vi "myRIO_BRig_RT_v0,73__PortC.vi"() -> ()   [LabVIEW 2014]
uses:
  myRIO_BRig_RT__Case_Exp_stateList.ctl
  myRIO_BRig_RT__Case_NonExp_stateList.ctl
  <vilib>/Platform/TimedLoop/XDataNode/timing_clust.ctl
  <vilib>/Platform/TimedLoop/XDataNode/nitl_modes.ctl
  <vilib>/Platform/TimedLoop/XDataNode/wakeup.ctl
  <vilib>/WebDAVClient/Advanced/SessionHandle.ctl
  <vilib>/myRIO/Common/Instrument Driver Framework/myRIO v1.0/UART/vis/myRIO v1.0 Close UART.vi
  <vilib>/FPGAPlugInAG/myRIO-1900/niLvFpga_Open_myRIO-1900.vi
  <vilib>/rvi/interface/common/dynamic/niFpgaDynamicAddResources.vi
  <vilib>/Utility/error.llb/Error Cluster From Error Code.vi
  <vilib>/rvi/errors/niLvFpgaAdjustHostInterfaceError.vi
  <vilib>/FPGAPlugInAG/Dynamic/niLvFpga_Close_Dynamic.vi
  <vilib>/myRIO/Common/Instrument Driver Framework/Utilities/vis/FPGA Ref Manager.vi
  <vilib>/myRIO/Common/Instrument Driver Framework/myRIO v1.0/myRIO v1.0 Reset FPGA.vi
  <vilib>/myRIO/Common/Instrument Driver Framework/myRIO v1.0/IRQ/vis/myRIO v1.0 IRQ Info FGV.vi
  <vilib>/myRIO/Common/Instrument Driver Framework/myRIO v1.0/IRQ/vis/myRIO v1.0 Timer IRQ Info FGV.vi
  <vilib>/myRIO/Common/Instrument Driver Framework/myRIO v1.0/IRQ/vis/myRIO v1.0 ISR Agent.vi
  <vilib>/rvi/interface/nirviOpenFPGA/nirviOpenFPGA.xnode
  myRIO_BRig_FPGA_v3,60__PortC__build.lvbitx
  myRIO_BRig_FPGA_v3,60__PortC.vi
  <vilib>/rvi/interface/nirviReadWriteControl/nirviReadWriteControl.xnode
  <vilib>/Platform/TimedLoop/XDataNode/XDataNode.xnode
  <vilib>/rvi/interface/nirviCloseFPGA/nirviCloseFPGA.xnode
  <vilib>/Platform/TimedLoop/XDataNode/XDNodeRunTimeDep.lvlib
  <vilib>/rvi/interface/Simulation/niFpgaSimulationCallBeginRW.vi
  <vilib>/myRIO/Instrument Drivers/Utilities/Utilities.lvlib
  <vilib>/WebDAVClient/NI_WebDAV.lvlib
  NiFpgaLv.dll
panel:
  in  "LC_Sel_All_Count":u16
  in  "LC_Sel_First_Count":u16
  in  "LC_Sel_All_Probability":u16
  in  "LC_Sel_All_Block":u16(slide) max=2 step=1 scale=0.0..2.0
  in  "LC_Sel_All_OnOff":bool
  in  "LC_Sel_First_Probability":u16
  in  "LC_Sel_First_Block":u16(slide) max=2 step=1 scale=0.0..2.0
  in  "LC_Sel_First_OnOff":bool
  in  "LC_Sel_All_Tdelay":u16
  in  "LC_Sel_First_Tdelay":u16
  out "I_connect_TCP":bool
  out "tempAI0":i16
  out "error out 5":errorcluster
  in  "get_countPerMS":bool
  in  "count_warmup_R_reset":bool
  in  "count_warmup_L_reset":bool
  out "count_warmup_R":u16
  out "count_warmup_L":u16
  out "SolenoidReward":bool
  in  "SolenoidProbability_L":u16=50 caption="Reward Time [ms]" min=1 max=1000 step=1
  in  "SolenoidProbability_R":u16=50 caption="Reward Time [ms]" min=1 max=1000 step=1
  out "output_PortA":dbl caption="LaserPower"
  out "error out 4":errorcluster
  in  "laser_power_step":dbl
  in  "laser_power_max":dbl
  in  "Recording":bool
  out "error out 3":errorcluster
  out "error out 2":errorcluster
  in  "laser_power_min":dbl
  in  "f_millisec2count":dbl=159.0
  in  "laser_Tshutter":dbl=2.0
  in  "laser_Freq":dbl=10.0
  in  "laser_Tpeak":dbl=2.0
  in  "laser_duration":u16
  out "error out":errorcluster
  in  "LC_Cue1_All_Count":u16
  in  "LC_Cue1_First_Count":u16
  in  "LC_Cue1_All_delayOpt":bool
  in  "LC_ENL1_All_delayOpt":bool
  in  "LC_ENL1_All_Count":u16
  in  "LC_ENL1_First_Count":u16
  in  "LC_Cue1_First_delayOpt":bool
  in  "LC_ENL1_First_delayOpt":bool
  in  "Tcycle_Cue_max":u16=1000 caption="Max" min=5 max=5000 step=5
  in  "Tcycle_Cue_min":u16=1000 caption="Min" min=5 max=5000 step=5
  in  "SendData":bool
  out "cSpout":enum16{"Left", "Right"}(ring) caption="Left or Right Spout"
  out "A4":u32 caption="LickCounter_Right"
  out "A2":u32 caption="LickCounter_Left"
  in  "laserResponse_wrong_LED":bool
  out "error_initTrial":errorcluster
  out "error_Selection_pre":errorcluster
  out "error_Selection":errorcluster
  out "SelectWrong":bool
  out "SelectReward":bool
  in  "Left(F)_or_Right(T)":bool
  in  "ignoreWrong":bool
  in  "SelectionState":bool
  in  "laserResponse_wrong":bool
  in  "laserResponse_reward":bool
  in  "laserResponse_reward_LED":bool
  out "nRewards_Right":u16 caption="# Rewards Total (Right)"
  out "nRewards_Left":u16 caption="# Rewards Total (Left)"
  out "nRewards_cur":u16 caption="# Rewards in Current Block"
  out "TpB_target":u16 caption="Target Trials Per Block"
  out "cState_NonExp":T1 caption="WarmUp State"
  out "iBlock":u16 caption="Current Block"
  out "cState":T2 caption="Experimental State"
  out "iTrial":u16 caption="Current Trial"
  in  "warmupType":u8(slide) max=2 step=1 scale=0.0..2.0
  in  "TestConnection":bool
  in  "warmup":bool caption="WarmUp"
  in  "Data Set Prefix":string="Exp1_TM2"
  out "Connected To Host?":bool
  in  "Host Password":string="sabalab"
  in  "Host UserName":string="Test2"
  in  "sp_RightSpout":u16(slide)=2 max=2 step=1 scale=0.0..2.0
  in  "sp_LeftSpout":u16(slide)=2 max=2 step=1 scale=0.0..2.0
  in  "BUR_max":u16 caption="Count Reward Structure  (0 = off)"
  in  "LC_Wrong_Probability":u16
  in  "LC_Wrong_Trial":u16(slide) max=2 step=1 scale=0.0..2.0
  in  "LC_Wrong_Block":u16(slide) max=2 step=1 scale=0.0..2.0
  in  "LC_Wrong_OnOff":bool
  in  "LC_Reward_Probability":u16
  in  "LC_Reward_Trial":u16(slide) max=2 step=1 scale=0.0..2.0
  in  "LC_Reward_Block":u16(slide) max=2 step=1 scale=0.0..2.0
  in  "LC_Reward_OnOff":bool
  in  "LC_Cue1_All_Probability":u16
  in  "LC_Cue1_All_Block":u16(slide) max=2 step=1 scale=0.0..2.0
  in  "LC_Cue1_All_OnOff":bool
  in  "LC_Cue1_First_Probability":u16
  in  "LC_Cue1_First_Block":u16(slide) max=2 step=1 scale=0.0..2.0
  in  "LC_Cue1_First_OnOff":bool
  in  "LC_ENL1_All_Probability":u16 max=100 step=1
  in  "LC_ENL1_All_Block":u16(slide) max=2 step=1 scale=0.0..2.0
  in  "LC_ENL1_All_OnOff":bool
  in  "LC_ENL1_First_Probability":u16 max=100 step=1
  in  "LC_ENL1_First_Block":u16(slide) max=2 step=1 scale=0.0..2.0
  in  "Tcycle_Timeout":u16=1000 caption="Timeout Time [ms]" min=10 max=10000 step=1
  in  "Tcycle_Wrong":u16=1000 caption="Wrong Time [ms]" min=10 max=10000 step=1
  in  "Tcycle_Selection":u16=1000 caption="Answer Time [ms]" min=1 max=10000 step=1
  in  "Tcycle_RewardPost":u16=1000 caption="Consumption Time [ms]" min=250 max=10000 step=250
  in  "Tcycle_Reward_L":u16=500 caption="Reward Time [ms]" min=1 max=1000 step=1
  in  "Tcycle_Reward_R":u16=500 caption="Reward Time [ms]" min=1 max=1000 step=1
  in  "TpB_Max_R":u16=4 caption="Max TrialsPerBlock" min=1 max=12 step=1
  in  "TpB_Min_R":u16=4 caption="Min TrialsPerBlock" min=1 max=12 step=1
  in  "TpB_Max_L":u16=4 caption="Max TrialsPerBlock" min=1 max=12 step=1
  in  "TpB_Min_L":u16=4 caption="Min TrialsPerBlock" min=1 max=12 step=1
  in  "BUR_min":u16 caption="Count Reward Structure\n(0 = off)"
  in  "TrialUntilReward":bool caption="Ignore Wrong Selection"
  in  "CueCycles":u16=1 caption="Cue Structure" min=1 max=1 step=1
  in  "MTrig_Laser_Tcycle":u16=10 caption="Time [ms]"
  in  "MTrig_Laser_trig":bool
  in  "MTrig_Audio_trig__R":bool caption="Trigger Audio"
  in  "MTrig_Audio_trig__L":bool caption="Trigger Audio"
  in  "RewCalib_Trig_R":bool caption="Calibrate_R"
  in  "RewCalib_Trig_L":bool caption="Calibrate_L"
  in  "MTrig_Solenoid_Tcycle__R":u16=300 caption="Time [ms]"
  in  "MTrig_Solenoid_Tcycle__L":u16=300 caption="Time [ms]"
  in  "MTrig_Solenoid_trig__R":bool caption="Solenoid"
  in  "MTrig_Solenoid_trig__L":bool caption="Solenoid"
  in  "STOP_abort":bool caption="Stop LabView\n(Stops myRio and FPGA)"
  in  "STOP_endBlock":bool caption="Stop Experiment\n@ End of Block"
  in  "STOP_endTrial":bool caption="Stop Experiment\n@ End of Trial"
  in  "START":bool caption="Start Experiment"
  in  "Tcycle_CuePenalty":u16=1000 caption="Penalty" min=1 max=10000 step=1
  in  "Audio_Amp__R":u16=100 caption="Amp"
  in  "Audio_Freq__R":u8=5 caption="Freq [kHz]" max=14 step=1
  in  "Audio_Amp__L":u16=100 caption="Amp"
  in  "Audio_Freq__L":u8=5 caption="Freq [kHz]" max=14 step=1
  in  "LC_Wrong_Tdelay":u16
  in  "LC_Cue1_All_Tdelay":u16
  in  "LC_ENL1_All_Tdelay":u16
  in  "LC_Reward_Tdelay":u16
  in  "LC_Cue1_First_Tdelay":u16
  in  "LC_ENL1_First_Tdelay":u16
  in  "LC_ENL1_First_OnOff":bool
  in  "Tcycle_ENLPenalty":u16=100 caption="Penalty" min=10 max=10000 step=10
  in  "Tcycle_ENL_max":u16=1000 caption="Max" min=250 max=10000 step=250
  in  "Tcycle_ENL_min":u16=1000 caption="Min" min=250 max=10000 step=250
  # "Experimental Run"
  # "Experiment Task Structure"
  # "Current State"
  # "Timing [ms]"
  # "Global Parameters\n \n   WarmUp State                                            Lick Counter"
  # "Min            Max            Penalty"
  # "(1) = Switching\n(2) = Two Choice"
  # "Enforced\nNonLick"
  # "Left                    Right"
  # "Cue"
  # "Experimental State"
  # "Communication (Host PC)"
  # "WarmUp"
  # "Selection\n \n \nReward\n    Dispense\n    Time\n \n    Dispense\n    Probability\n \n    Consumption\n    Time\n \nWrong Choice\n \n \nTimeout Penalty"
  # "Trial Parameters\n \n   Left/Right        Give Reward?        Laser Power [V]"
  # "Left                  Right"
  # "Min"
  # "Max"
  # "Block                   Trial            Target Trials       # Rewards \n                                                            Per Block             Current"
  # "Trial Per Block Structure \n               Left                        Right"
  # "Min"
  # "# Rewards Total\n                                                                  Left                    Right"
  # "Recording Rig"
  # "FPGA Conv."
  # "Cue then reward (no lick)\n \nLeft                    Right"
  # "Max"
  # "FPGA count per ms"
  # "Laser Control\n\n                               On/Off      Block        Probability [%]   Delay [ms]                              Count"
  # "Manual Control"
  # "Enforced\nNonLick\n      1"
  # "Solenoid\n \nLeft              Right"
  # "Speaker\n \nLeft                    Right"
  # "Laser"
  # "from end"
  # "Switch\nTrial"
  # "from start"
  # "from end"
  # "NonSwitch\nTrials"
  # "Time\n[ms]"
  # "Time\n[ms]"
  # "from start"
  # "Time = Cue Min"
  # "Cue 1"
  # "Power = Min"
  # "from end"
  # "Switch\nTrial"
  # "from start"
  # "Speaker Parameters"
  # "Laser Parameters"
  # "Left                  Right"
  # "from end"
  # "Frequency\n[Hz]"
  # "NonSwitch\nTrials"
  # "Frequency\n[kHz]"
  # "from start"
  # "Timing [ms]\n Duration     Peak Width   Shutter"
  # "Selection"
  # "Amp\n(0 - 32,000)"
  # "Switch\nTrial"
  # "Laser Power [V]\nMin          Max              Step"
  # "Speaker\nPattern\nDuring Cue"
  # "NonSwitch\nTrials"
  # "Selection Reward"
  # "Selection Wrong"
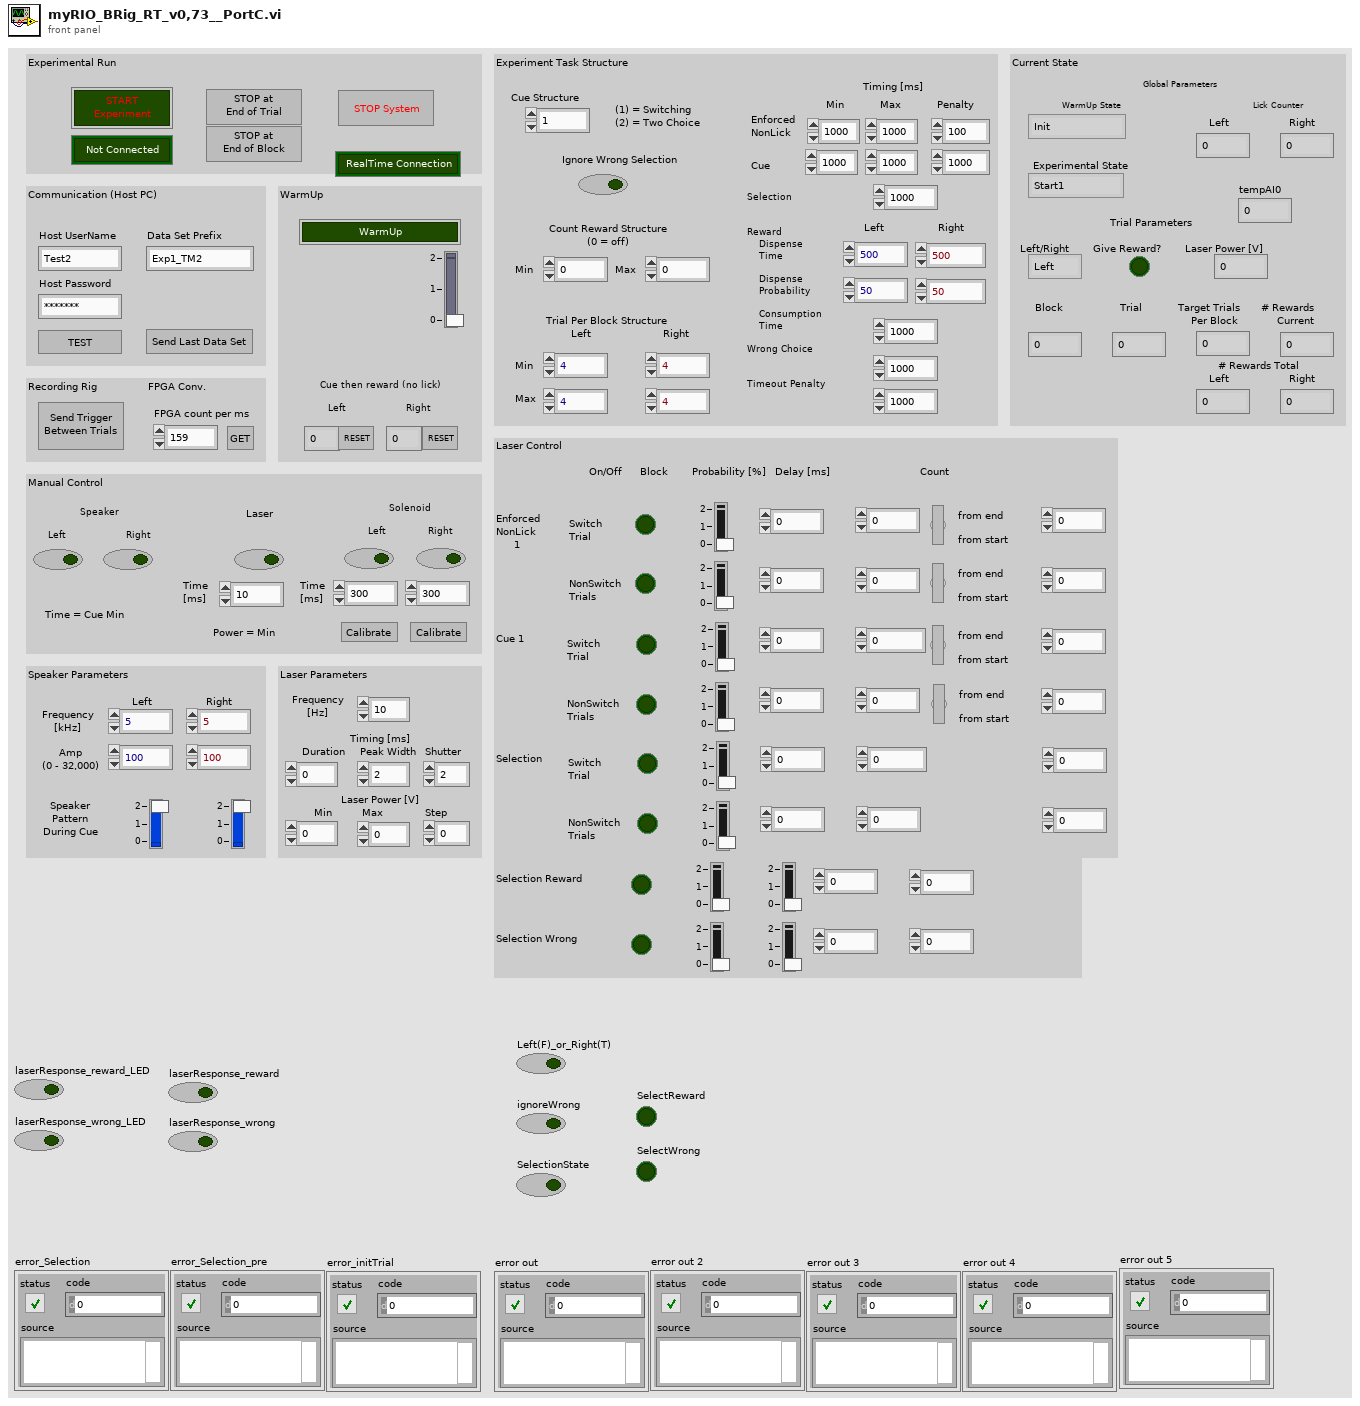
[diagram p1: front panel]
types:
  T1 = typedef "myRIO_BRig_RT__Case_NonExp_stateList.ctl" = enum16{"Init", "UploadSettings_pre", "UploadSettings_Read_dataExp", "UploadSettings_dataExp_1", "UploadSettings_Read_dataLC", "UploadSettings_dataLC_1", "UploadSettings_dataLC_2", "UploadSettings_Read_dataMTrig", "UploadSettings_dataMTrig_1", "UploadSettings_post", "Idle_pre", "IdleEmpty", "IdleEmpty2", "IdleEmpty3", "IdleEmpty4", "Idle", "Idle_2", "Idle_3", "Idle_4", "Idle_post", "Cue_pre__pre", "Cue_pre", "Cue", "Cue_post", "RewardCalibration_pre", "DispenseWater_pre__pre", "DispenseWater_pre", "DispenseWater", "DispenseWater_post", "TestConnection", "SendData", "Get_FPGA_count_per_ms", "End"}
  T2 = typedef "myRIO_BRig_RT__Case_Exp_stateList.ctl" = enum16{"Start1", "Start2", "Start3", "saveSettings1", "saveSettings2", "saveSettings3", "saveSettings4_LC_ENL", "saveSettings5_LC_Cue", "saveSettings6_LC_Other", "setSettings_Audio", "setSettings_Laser", "initBlock_pre", "initBlock", "initBlock2", "initBlock_post", "initTrial_pre", "initTrial", "initTrial2", "initTrial3", "initTrial4", "initTrial_LC_ENL1", "initTrial_LC_Cue1", "initTrial_LC_Sel", "initTrial_post", "ENL1_pre", "ENL1", "ENL1_post", "ENL1Penalty_pre", "ENL1Penalty", "ENL2_pre", "ENL2", "ENL2Penalty_pre", "ENL2Penalty", "Cue1_pre", "Cue1", "Cue1_post", "Cue1Penalty_pre", "Cue1Penalty", "Cue2_pre", "Cue2", "Cue2Penalty_pre", "Cue2Penalty", "Selection_pre", "Selection", "Select_post", "SelectReward_pre", "SelectReward", "SelectRewardPost_pre", "SelectRewardPost", "SelectWrong_pre", "SelectWrong", "SelectWrong_post", "SelectTimeout_pre", "SelectTimeout", "SelectTimeout_post", "endTrial_pre", "endTrial1", "endTrial2", "endTrial3", "endTrial_post", "endBlock_pre", "endBlock", "endBlock_post", "endExp", "commConnect", "commUpload_pre", "commUpload_dataBlock", "commUpload_dataCurrent", "commUpload_dataExp", "commUpload_dataLC", "commUpload_dataTrial", "commUpload_post", "saveData_pre", "saveData_dataBlock", "saveData_dataCurrent", "saveData_dataExp", "saveData_dataLC", "saveData_dataTrial", "saveData_post", "empty_endBlock1", "empty_endBlock2", "empty_endTrial1", "empty_endTrial2", "empty_endTrial3", "empty_endTrial4", "empty_endTrial5", "dummyState", "dummyState_endBlock"}
  T3 = typedef "XDNodeRunTimeDep.lvlib/timing_clust.ctl" = cluster{"Expected End [f-1]":u64, "Actual End [f-1]":u64, "Finished Late? [f-1]":bool, "Expected End [i-1]":u64, "Actual End [i-1]":u64, "Finished Late? [i-1]":bool, "Expected Start [i]":u64, "Actual Start [i]":u64, "Expected Start [f]":u64, "Actual Start [f]":u64, "Source Name":string, "Structure Name":string, "Period":i64, "Deadline":i64, "Offset":i64, "Start":i64, "Priority":i32, "Timeout":i32, "Mode":T4, "Wakeup Reason":T5, "Error":errorcluster, "Source Type":string, "Secondary Source Type":string, "Global End Time":u64, "Global Start Time":u64, "Frame Duration":u64, "Iteration Duration":u64, "Assigned CPU":i32, "I/O Scan Engine Mode":u32}
  T4 = typedef "XDNodeRunTimeDep.lvlib/nitl_modes.ctl" = enum32{"No Change", "Process missed periods, maintain original phase", "Discard missed periods, maintain original phase", "Process missed periods, ignore original phase", "Discard missed periods, ignore original phase"}
  T5 = typedef "XDNodeRunTimeDep.lvlib/wakeup.ctl" = enum32{"Normal", "Aborted", "Asynchronous wakeup", "Timing source error", "Timed loop error", "Timeout"}
  T6 = typedef "NI_WebDAV.lvlib/SessionHandle.ctl" = refnum<k1>
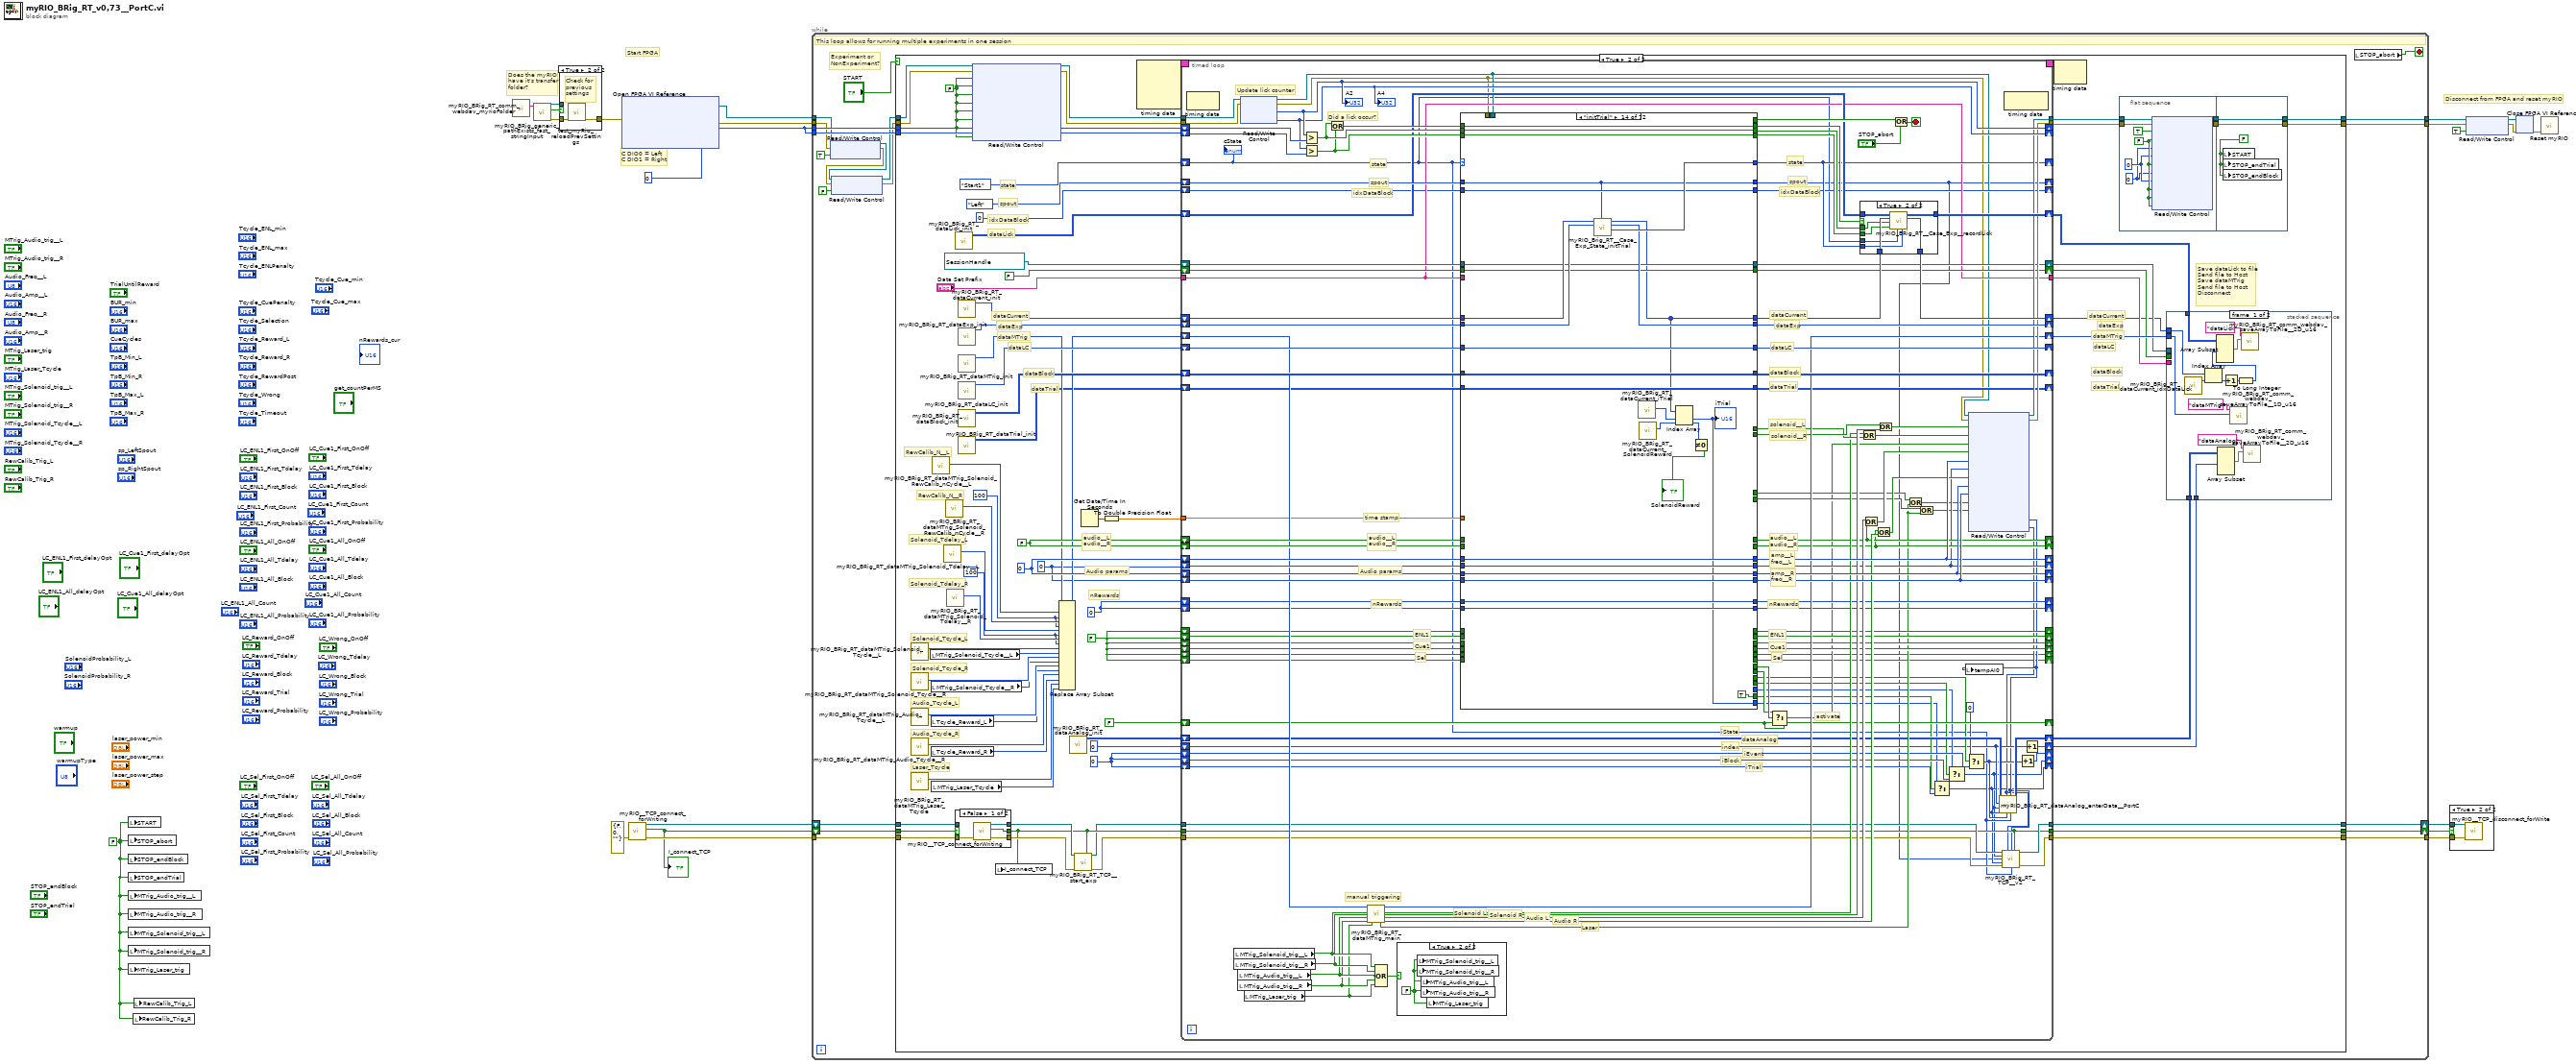
[diagram p0: block diagram]
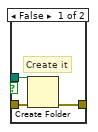
[diagram p3: hidden frame]
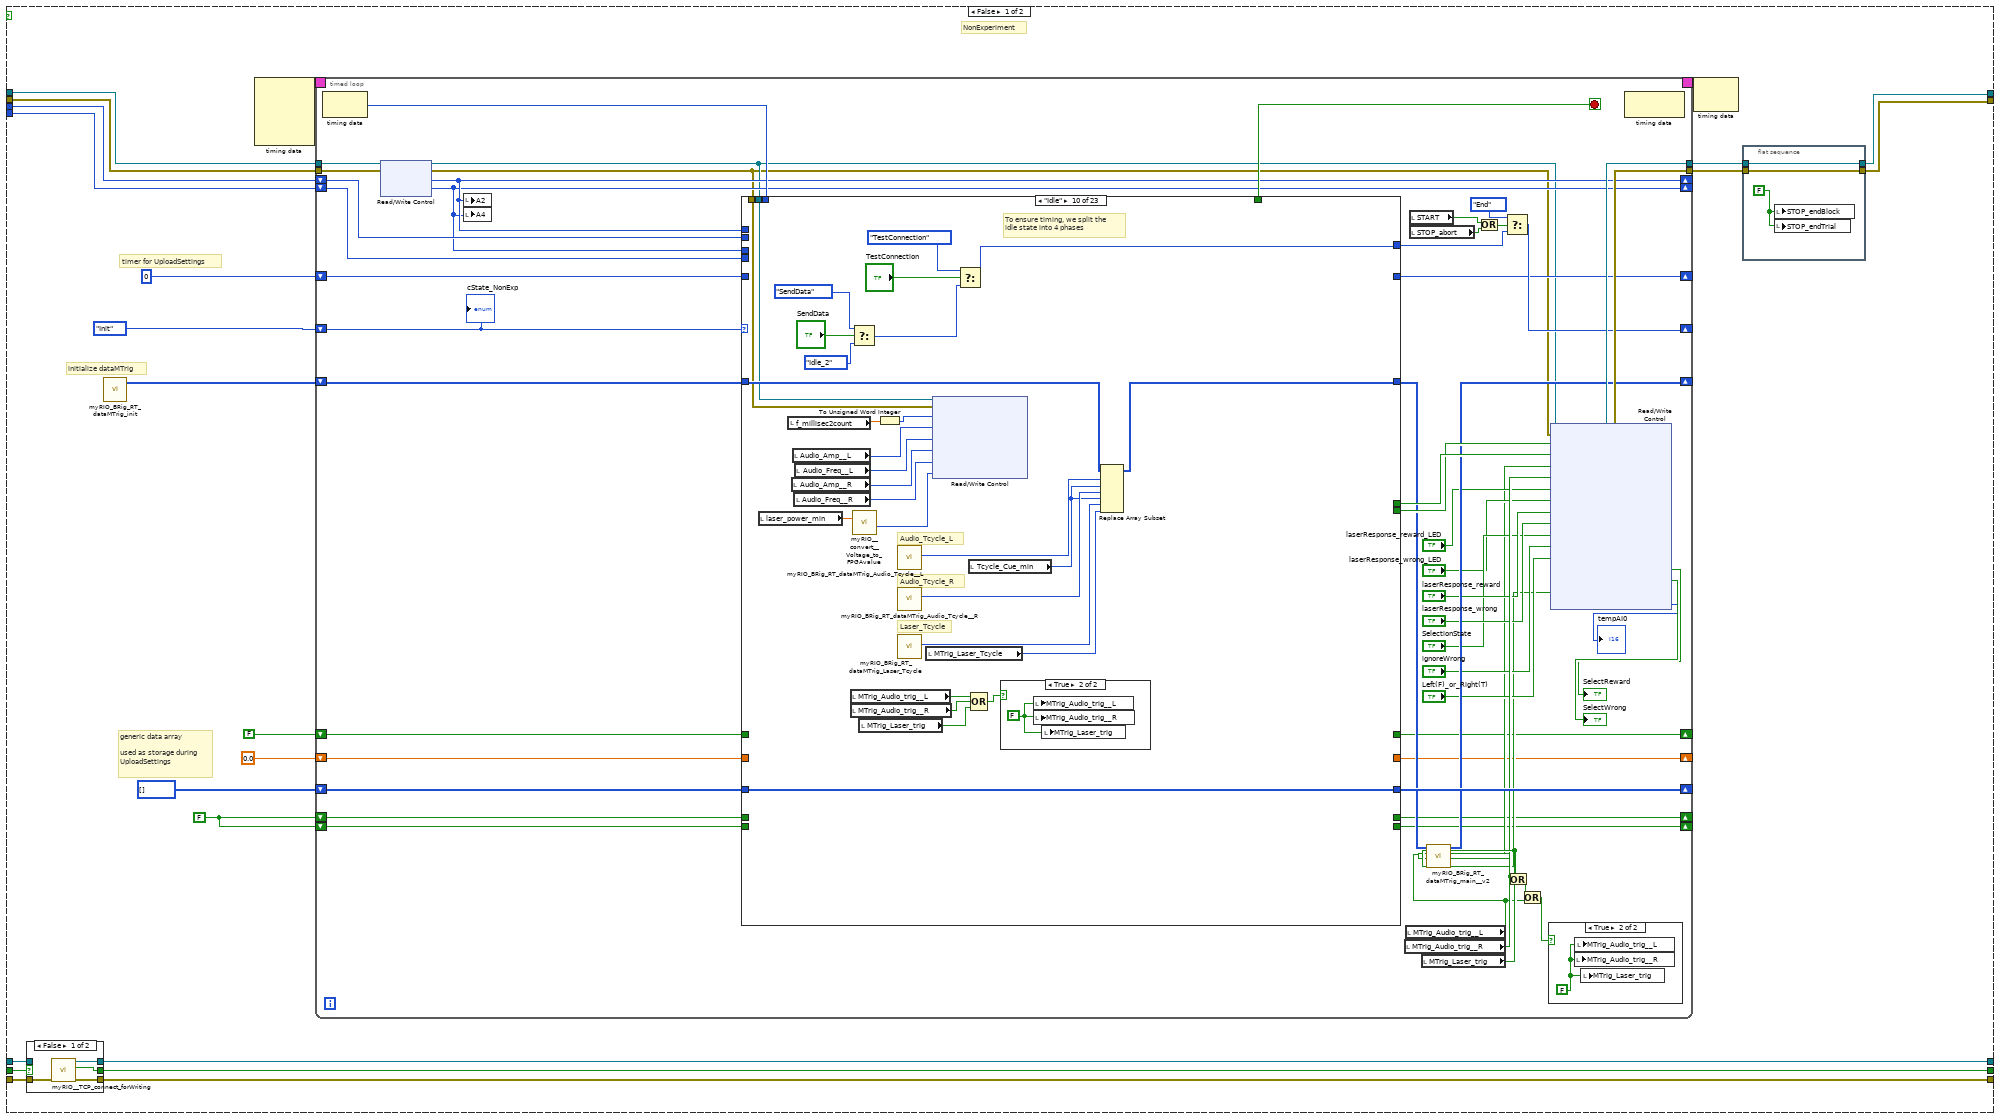
[diagram p4: hidden frame]
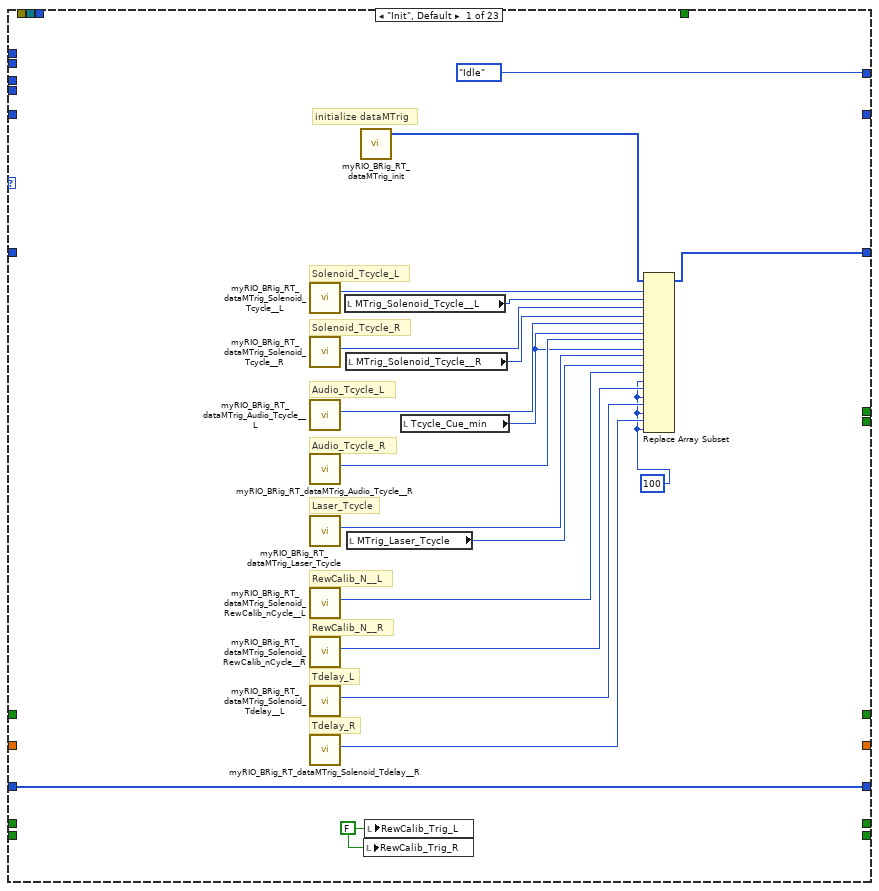
[diagram p7: hidden frame]
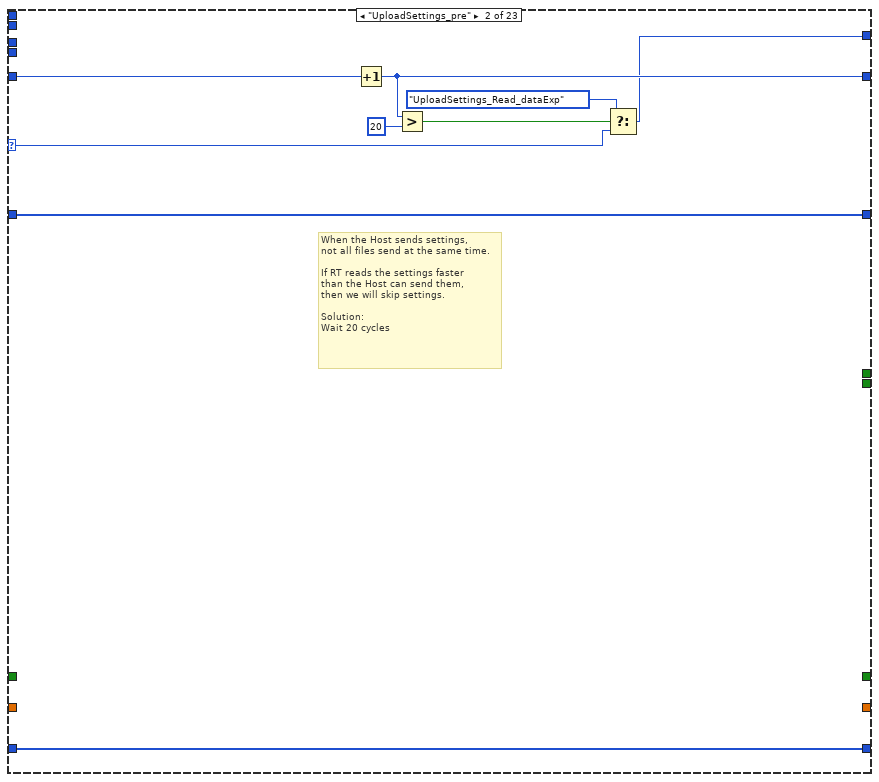
[diagram p8: hidden frame]
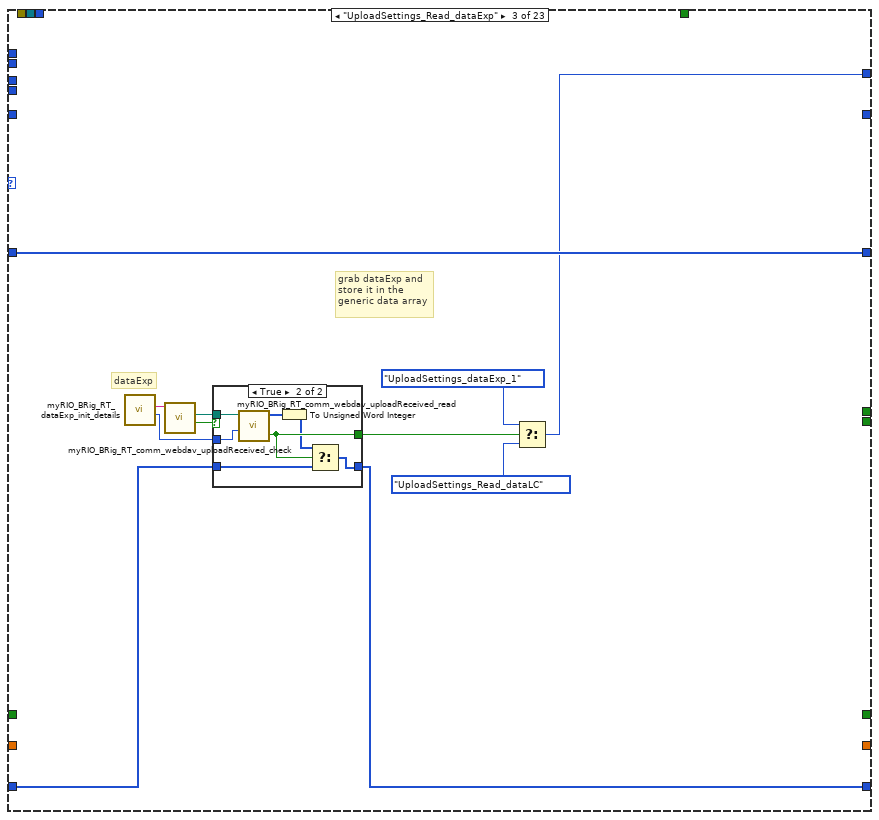
[diagram p9: hidden frame]
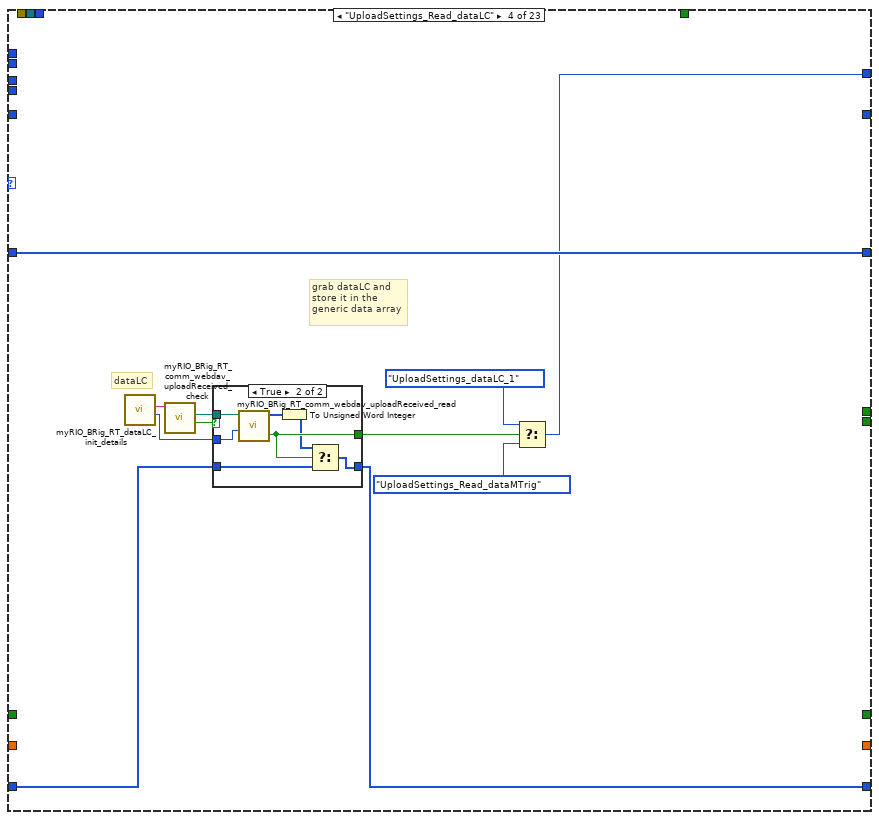
[diagram p11: hidden frame]
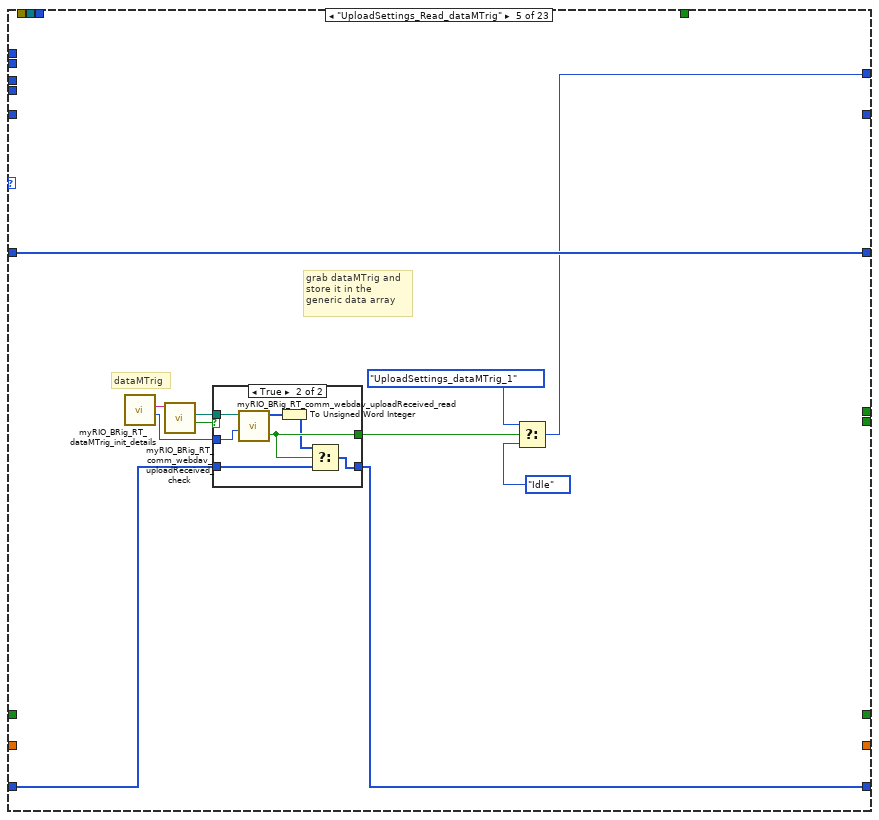
[diagram p13: hidden frame]
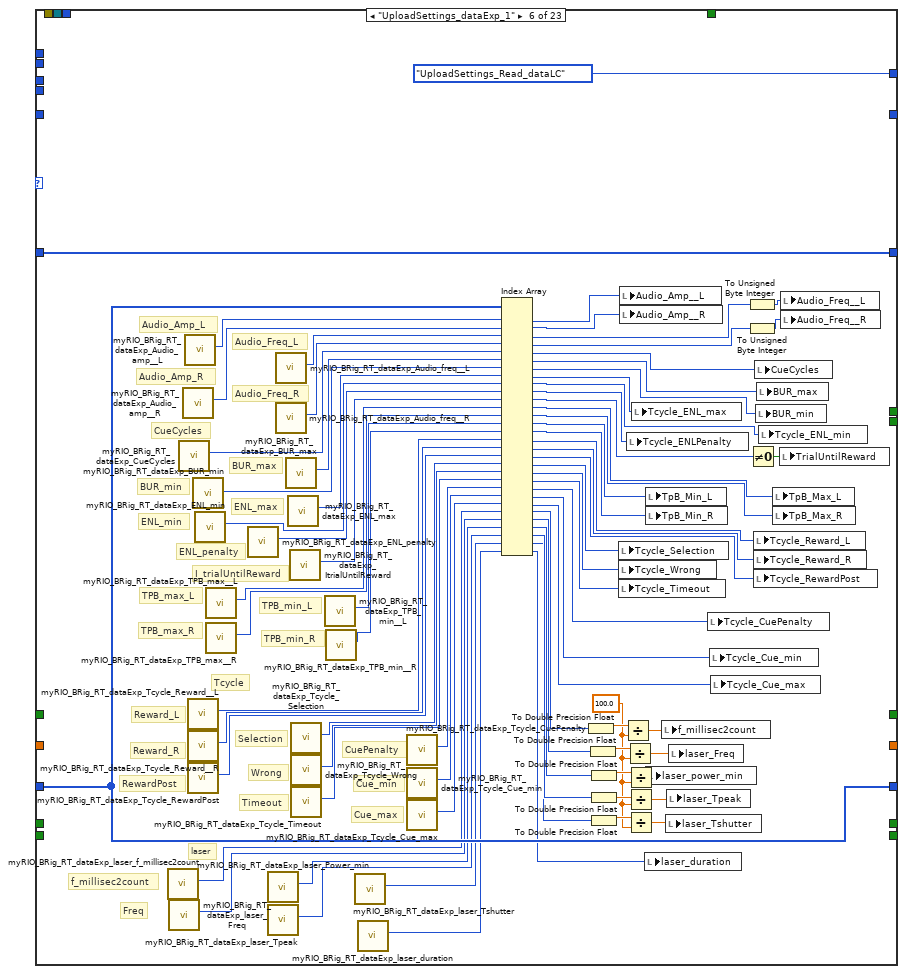
[diagram p15: hidden frame]
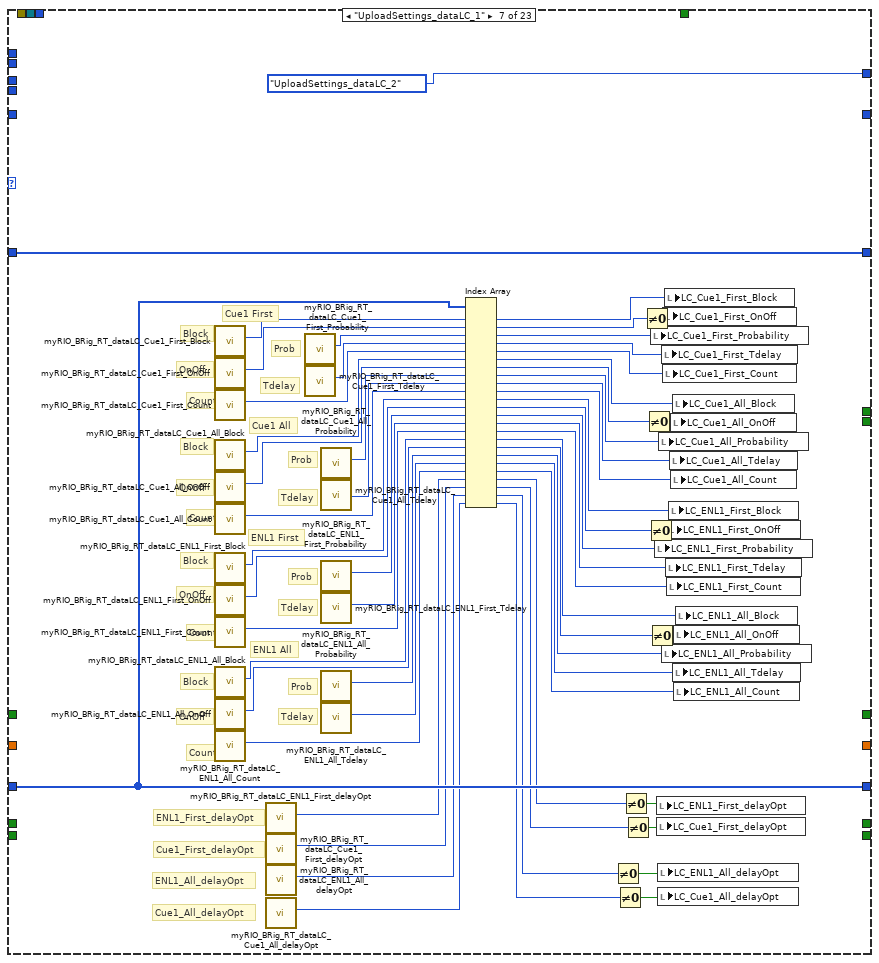
[diagram p16: hidden frame]
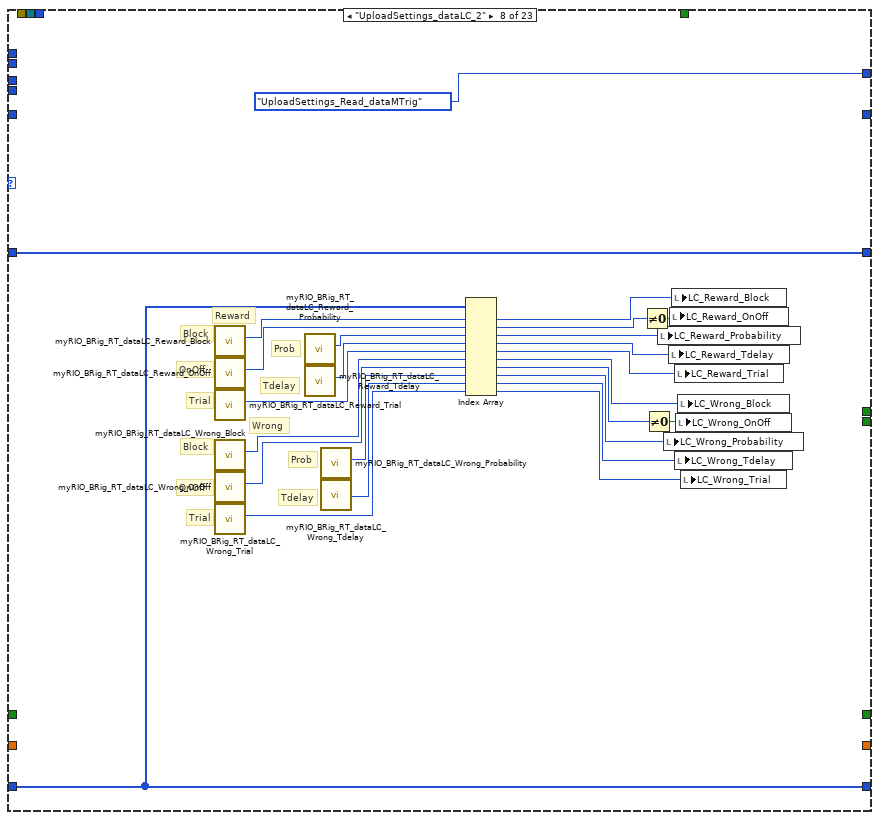
[diagram p17: hidden frame]
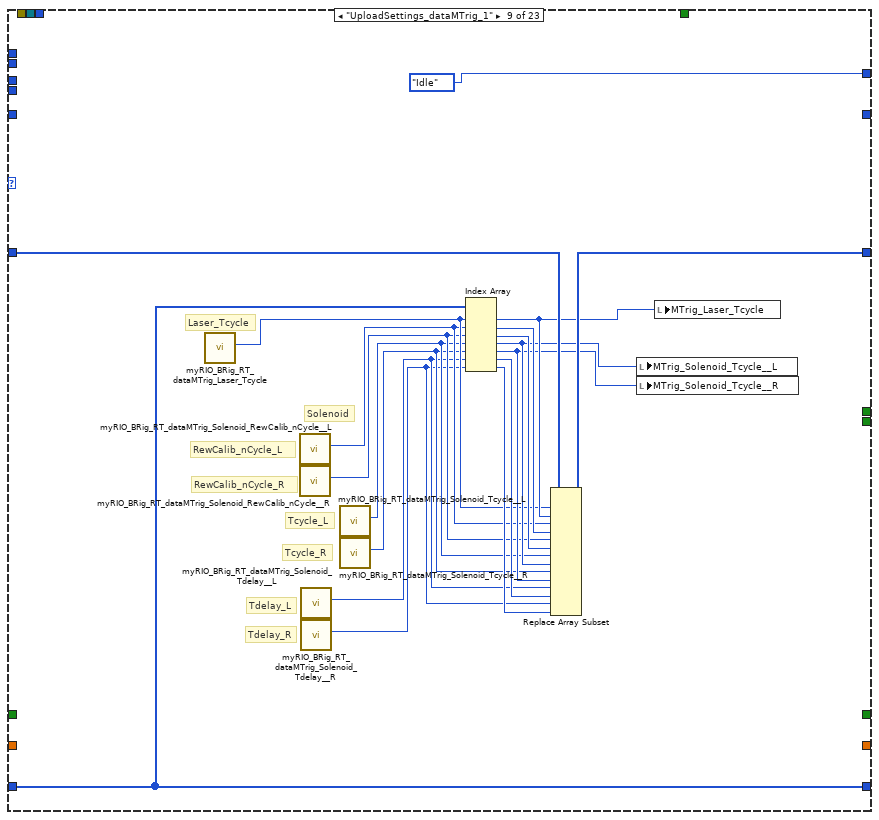
[diagram p18: hidden frame]
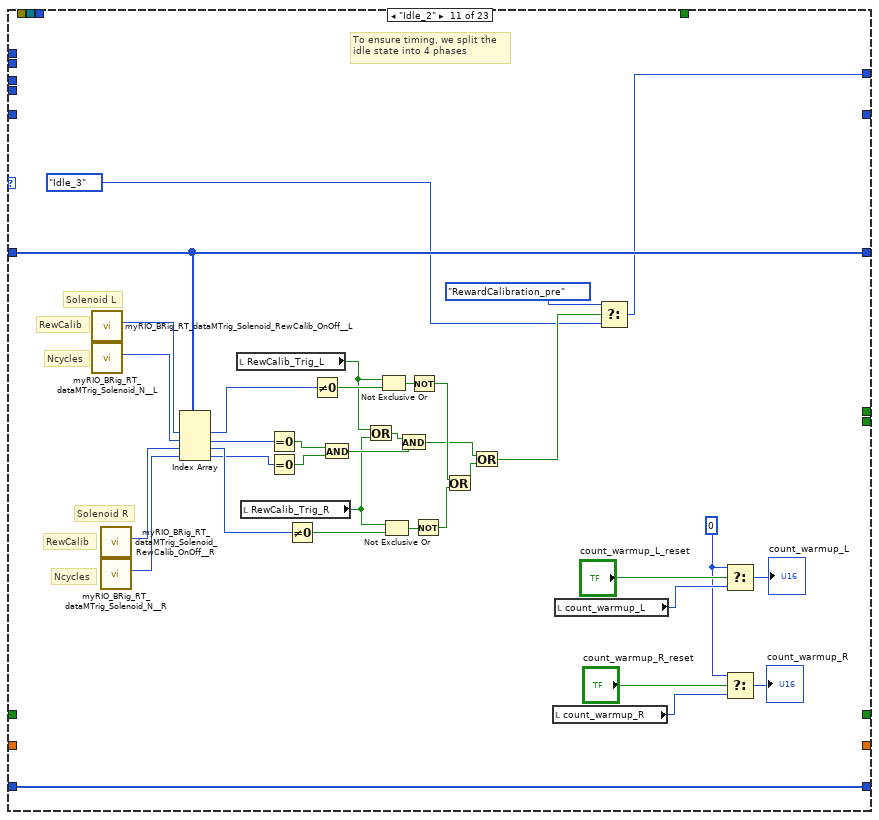
[diagram p20: hidden frame]
diagram:
  w16 = u32 0
  w13 = FALSE
  # "Does the myRIO\nhave it's transfer\nfolder?"
  # "C DIO0 = Left\nC DIO1 = Right"
  # "Start FPGA"
  # "Disconnect from FPGA and reset myRIO"
  n1 = local write "START"(w13) -> ()
  n2 = local write "STOP_abort"(w13) -> ()
  n3 = local write "STOP_endBlock"(w13) -> ()
  n4 = local write "STOP_endTrial"(w13) -> ()
  n5 = local write "MTrig_Audio_trig__L"(w13) -> ()
  n6 = local write "MTrig_Audio_trig__R"(w13) -> ()
  n7 = local write "MTrig_Solenoid_trig__L"(w13) -> ()
  n8 = local write "MTrig_Solenoid_trig__R"(w13) -> ()
  n9 = local write "MTrig_Laser_trig"(w13) -> ()
  n10 = local write "RewCalib_Trig_R"(w13) -> ()
  n11 = local write "RewCalib_Trig_L"(w13) -> ()
  n12 = call "myRIO_BRig_RT_comm_webdav_myrioFolder.vi"() -> ("output_myrioFolder"=w12:string)  [unwired: 11 in]
  n13 = call "myRIO_BRig_generic_pathExists_fast_stringInput.vi"("input_filePath"=w12) -> ("output_error"=w11:errorcluster, "output_Iexist"=w10:bool, "output_filePath"=w9:path)  [unwired: 8 in]
  n14 = case shown="True" w10 {
    tunnel: w9 -> [w25 _]
    tunnel: w11 -> [w24 w27]
    tunnel: [w23 w26] -> w7
    frame False {
      # "Create it"
      n15 = Create Folder(path (use dialog)=w25, error in=w24) -> (error out=w23:errorcluster)  [unwired: 1 in, 2 out]
    }
    frame True {
      # "Check for\nprevious\nsettings"
      n16 = call "test_myRio_reloadPrevSettings.vi"("input_error"=w27) -> ("output_error"=w26:errorcluster)  [unwired: 10 in]
    }
  }
  n17 = xnode "Open FPGA VI Reference"("error in"=w7) -> ("FPGA VI Reference Out"=w18:refnum<k20>, "error out"=w17:errorcluster)  [unwired: 1 in]
  n18 = call "myRIO__TCP_connect_forWriting.vi"("input_error"=errorcluster {"status"=FALSE, "code"=0, "source"=""}) -> ("output_error"=w5:errorcluster, "output_connected"=w4:bool, "output_hTCP"=w8:refnum<k5>)  [unwired: 8 in]
  "I_connect_TCP" <- w4
  n19 = while {
    tunnel: w18 -> [w37]
    tunnel: w17 -> [w42]
    tunnel: w16 -> [w45]
    tunnel: w16 -> [w44]
    tunnel: [w35] -> w15
    tunnel: [w34] -> w14
    shift-right: [w31] -> w3
    shift-left: w4 -> [w32]
    tunnel: w5 -> [w30]
    shift-right: [w29] -> w2
    shift-left: w8 -> [w33]
    tunnel: [w28] -> w1
    stop <- w43 stop-if-true
    # "Experiment or\nNonExperiment?"
    # "This loop allows for running multiple experiments in one session"
    n20 = xnode "Read/Write Control"("FPGA VI Reference In"=w37, "error in"=w42, "Counts_Reset"=TRUE) -> ("FPGA VI Reference Out"=w39:refnum<k20>, "error out"=w40:errorcluster)
    n21 = xnode "Read/Write Control"("FPGA VI Reference In"=w39, "error in"=w40, "Counts_Reset"=FALSE) -> ("FPGA VI Reference Out"=w36:refnum<k20>, "error out"=w38:errorcluster)
    n22 = case shown="True" "START" {
      tunnel: w45 -> [w66 w994]
      tunnel: w44 -> [w65 w993]
      tunnel: w38 -> [w63 w944]
      tunnel: w36 -> [w64 w943]
      tunnel: [w61 w990] -> w35
      tunnel: [w59 w985] -> w34
      tunnel: w33 -> [w52 w930]
      tunnel: [w50 w934] -> w29
      tunnel: w32 -> [w51 w932]
      tunnel: [w49 w933] -> w31
      tunnel: w30 -> [w53 w931]
      tunnel: [w48 w929] -> w28
      frame False {
        w56 = FALSE
        # "generic data array\n\nused as storage during\nUploadSettings"
        # "timer for UploadSettings"
        # "initialize dataMTrig"
        # "NonExperiment"
        n23 = case shown="False" w51 {
          selector: w51 -> [_ w75]
          tunnel: w53 -> [w72 w77]
          tunnel: [w73 w77] -> w48
          tunnel: w52 -> [_ w76]
          tunnel: [w74 w76] -> w50
          tunnel: [w71 w75] -> w49
          frame False {
            n24 = call "myRIO__TCP_connect_forWriting.vi"("input_error"=w72) -> ("output_error"=w73:errorcluster, "output_connected"=w71:bool, "output_hTCP"=w74:refnum<k5>)  [unwired: 8 in]
          }
          frame True {
          }
        }
        n25 = call "myRIO_BRig_RT_dataMTrig_init.vi"() -> ("output_dataMTrig"=w67:u16[])  [unwired: 5 in]
        n26 = node-c288() -> (w70:T3)  [unwired: 4 in]
        n27 = timed-loop {
          timing: w70 -> [_]
          timing-out: [_] -> w69
          shift-right: [w121] -> _
          shift-left: w67 -> [w133]
          shift-right: [w110] -> _
          shift-left: myRIO_BRig_RT__Case_NonExp_stateList."Init" ("Enum") -> [w127]
          shift-right: [w94] -> _
          shift-left: w66 -> [w95]
          shift-right: [w92] -> _
          shift-left: w65 -> [w93]
          tunnel: [w129] -> w62
          tunnel: [w128] -> w60
          tunnel: w63 -> [w131]
          tunnel: w64 -> [w130]
          shift-right: [w126] -> _
          shift-left: u16[] [] ("output_data") -> [w125]
          shift-right: [w96] -> _
          shift-left: u16 0 ("Audio_Amp__L") -> [w97]
          shift-right: [w89] -> _
          shift-left: w56 -> [w91]
          shift-right: [w88] -> _
          shift-left: w56 -> [w90]
          shift-right: [w84] -> _
          shift-left: FALSE -> [w85]
          shift-right: [w82] -> _
          shift-left: 0.0 -> [w83]
          stop <- w134 stop-if-true
          n28 = node-c288() -> (w132:i64)  [unwired: 1 in]
          n29 = xnode "Read/Write Control"("FPGA VI Reference In"=w130, "error in"=w131) -> ("FPGA VI Reference Out"=w87:refnum<k20>, "error out"=w86:errorcluster, "A2_LickL"=w94:u32, "A4_LickR"=w92:u32)
          n30 = local write "A2"(w94) -> ()
          n31 = local write "A4"(w92) -> ()
          n32 = case shown="\"Idle\"" w127 {
            selector: w127 -> [_ w159 _ _ _ _ _ _ _ _ _ _ _ _ w590 _ _ w798 _ _ _ w873 w917]
            tunnel: [myRIO_BRig_RT__Case_NonExp_stateList."Idle" ("Enum") w157 w164 w183 w202 myRIO_BRig_RT__Case_NonExp_stateList."UploadSettings_Read_dataLC" ("Enum") myRIO_BRig_RT__Case_NonExp_stateList."UploadSettings_dataLC_2" ("Enum") myRIO_BRig_RT__Case_NonExp_stateList."UploadSettings_Read_dataMTrig" ("f") myRIO_BRig_RT__Case_NonExp_stateList."Idle" ("Enum") w421 w438 w477 w558 myRIO_BRig_RT__Case_NonExp_stateList."Cue" ("t") w585 myRIO_BRig_RT__Case_NonExp_stateList."DispenseWater_pre" ("Enum") w743 w796 w819 myRIO_BRig_RT__Case_NonExp_stateList."Idle" ("Enum") myRIO_BRig_RT__Case_NonExp_stateList."Idle" ("Enum") w872 w917] -> w111
            tunnel: [w146 w156 w174 w193 w212 w297 w356 w381 w397 w425 w453 w482 w556 w574 w591 w653 w780 w803 w830 w865 w871 w884 w915] -> w122
            tunnel: [_ _ _ _ _ _ _ _ _ _ _ _ _ _ _ _ _ _ _ _ _ _ TRUE] -> w134
            tunnel: w133 -> [_ w156 w174 w193 w212 w297 w356 w381 w398 w424 w453 w483 w556 w575 w592 w639 w776 w804 w831 w865 w871 w884 w915]
            tunnel: w132 -> [_ _ _ _ _ _ _ _ _ _ _ _ _ _ _ _ _ w808 _ _ _ _ _]
            tunnel: [w139 w155 w165 w184 w203 w246 w312 w357 w382 w416 w437 w471 w555 w564 w599 w634 w728 w781 w812 w857 w869 w883 w914] -> w126
            tunnel: w125 -> [w139 w155 w166 w185 w204 w246 w312 w357 w382 w416 w437 w471 w555 w564 w599 w634 w728 w781 w812 w857 w869 w883 w914]
            tunnel: [_ _ _ _ _ _ _ _ _ _ _ _ _ _ _ _ _ w805 _ _ _ _ _] -> w124
            tunnel: [_ _ _ _ _ _ _ _ _ _ _ _ _ _ _ _ _ w787 _ _ _ _ _] -> w123
            tunnel: w97 -> [_ w163 _ _ _ _ _ _ _ _ _ _ _ _ _ _ _ _ _ _ _ _ _]
            tunnel: [_ w162 _ _ _ _ _ _ _ _ _ _ _ _ _ _ _ _ _ _ _ _ _] -> w96
            tunnel: w95 -> [_ _ _ _ _ _ _ _ _ _ _ _ _ _ w596 _ _ _ _ _ _ _ _]
            tunnel: w94 -> [_ _ _ _ _ _ _ _ _ _ _ _ _ _ w597 _ _ _ _ _ _ _ _]
            tunnel: w93 -> [_ _ _ _ _ _ _ _ _ _ _ _ _ _ w594 _ _ _ _ _ _ _ _]
            tunnel: w92 -> [_ _ _ _ _ _ _ _ _ _ _ _ _ _ w595 _ _ _ _ _ _ _ _]
            tunnel: w91 -> [_ _ _ _ _ _ _ _ _ _ _ _ _ _ w582 _ _ _ _ _ _ _ _]
            tunnel: w90 -> [_ _ _ _ _ _ _ _ _ _ _ _ _ _ w581 _ _ _ _ _ _ _ _]
            tunnel: [_ _ _ _ _ _ _ _ _ _ _ _ _ w563 w582 _ _ _ _ _ _ _ _] -> w89
            tunnel: [_ _ _ _ _ _ _ _ _ _ _ _ _ w562 w581 _ _ _ _ _ _ _ _] -> w88
            tunnel: w87 -> [_ _ _ _ _ _ _ _ _ w407 _ _ _ _ _ _ _ _ _ _ _ w878 _]
            tunnel: w86 -> [_ _ _ _ _ _ _ _ _ w406 _ _ _ _ _ _ _ _ _ _ _ w877 _]
            tunnel: w85 -> [_ _ _ _ _ _ _ _ _ _ _ _ _ _ _ _ _ _ _ _ _ w882 _]
            tunnel: [_ _ _ _ _ _ _ _ _ _ _ _ _ _ _ _ _ _ _ _ _ TRUE _] -> w84
            tunnel: w83 -> [_ _ _ _ _ _ _ _ _ _ _ _ _ _ _ _ _ _ _ _ _ w880 _]
            tunnel: [_ _ _ _ _ _ _ _ _ _ _ _ _ _ _ _ _ _ _ _ _ w879 _] -> w82
            frame "Init", Default {
              w140 = FALSE ("RewCalib_Trig_L")
              w136 = u16 100 ("new element/subarray")
              # "Tdelay_R"
              # "Tdelay_L"
              # "RewCalib_N__R"
              # "RewCalib_N__L"
              # "Solenoid_Tcycle_R"
              # "Solenoid_Tcycle_L"
              # "Laser_Tcycle"
              # "Audio_Tcycle_R"
              # "Audio_Tcycle_L"
              # "initialize dataMTrig"
              n33 = call "myRIO_BRig_RT_dataMTrig_Solenoid_Tcycle__L.vi"() -> ("output_Solenoid_Tcycle__L"=w148:i32)  [unwired: 11 in]
              n34 = call "myRIO_BRig_RT_dataMTrig_Solenoid_Tcycle__R.vi"() -> ("output_Solenoid_Tcycle__R"=w149:i32)  [unwired: 11 in]
              n35 = call "myRIO_BRig_RT_dataMTrig_Audio_Tcycle__L.vi"() -> ("output_Audio_Tcycle__L"=w150:i32)  [unwired: 11 in]
              n36 = call "myRIO_BRig_RT_dataMTrig_Audio_Tcycle__R.vi"() -> ("output_Audio_Tcycle__R"=w151:i32)  [unwired: 11 in]
              n37 = call "myRIO_BRig_RT_dataMTrig_Laser_Tcycle.vi"() -> ("output_Laser_Tcycle"=w152:i32)  [unwired: 11 in]
              n38 = call "myRIO_BRig_RT_dataMTrig_Solenoid_RewCalib_nCycle__L.vi"() -> ("output_Solenoid_RewCalib_nCycle__L"=w144:i32)  [unwired: 11 in]
              n39 = call "myRIO_BRig_RT_dataMTrig_Solenoid_RewCalib_nCycle__R.vi"() -> ("output_Solenoid_RewCalib_nCycle__R"=w143:i32)  [unwired: 11 in]
              n40 = call "myRIO_BRig_RT_dataMTrig_Solenoid_Tdelay__L.vi"() -> ("output_Solenoid_Tdelay__L"=w142:i32)  [unwired: 11 in]
              n41 = call "myRIO_BRig_RT_dataMTrig_Solenoid_Tdelay__R.vi"() -> ("output_Solenoid_Tdelay__R"=w141:i32)  [unwired: 11 in]
              n42 = local read "MTrig_Solenoid_Tcycle__L"() -> (w153:u16)
              n43 = local read "MTrig_Solenoid_Tcycle__R"() -> (w154:u16)
              n44 = local read "MTrig_Laser_Tcycle"() -> (w137:u16)
              n45 = call "myRIO_BRig_RT_dataMTrig_init.vi"() -> ("output_dataMTrig"=w147:u16[])  [unwired: 5 in]
              n46 = local write "RewCalib_Trig_R"(w140) -> ()
              n47 = local write "RewCalib_Trig_L"(w140) -> ()
              n48 = local read "Tcycle_Cue_min"() -> (w138:u16)
              n49 = Replace Array Subset(array=w147, new element #1=w153, index #1=w148, new element #2=w154, index #2=w149, new element #3=w138, index #3=w150, new element #4=w138, index #4=w151, new element #5=w137, index #5=w152, new element #6=w136, index #6=w144, new element #7=w136, index #7=w143, new element #8=w136, index #8=w142, new element #9=w136, index #9=w141) -> (w146:u16[])
            }
            frame "UploadSettings_pre" {
              # "When the Host sends settings,\nnot all files send at the same time.\n\nIf RT reads the settings faster\nthan the Host can send them,\nthen we will skip settings.\n\nSolution:\nWait 20 cycles"
              n50 = Increment(x=w163) -> (x+1=w162:u16)
              n51 = Greater?(x=w162, y=u16 20) -> (0:w160:bool)
              n52 = Select(t=myRIO_BRig_RT__Case_NonExp_stateList."UploadSettings_Read_dataExp", s=w160, f=w159) -> (s? t:f=w157:T1)
            }
            frame "UploadSettings_Read_dataExp" {
              # "grab dataExp and\nstore it in the\ngeneric data array"
              # "dataExp"
              n53 = call "myRIO_BRig_RT_dataExp_init_details.vi"() -> ("output_dataSize"=w170:i32, "output_dataName"=w173:string)  [unwired: 10 in]
              n54 = call "myRIO_BRig_RT_comm_webdav_uploadReceived_check.vi"("input_dataName"=w173) -> ("output_Iexist"=w172:bool, "output_dataPath"=w171:path)  [unwired: 9 in]
              n55 = case shown="True" w172 {
                tunnel: w171 -> [_ w182]
                tunnel: w170 -> [_ w181]
                tunnel: [_ w180] -> w169
                tunnel: w166 -> [w175 w179]
                tunnel: [w175 w176] -> w165
                frame False {
                }
                frame True {
                  n56 = call "myRIO_BRig_RT_comm_webdav_uploadReceived_read.vi"("input_dataSize"=w181, "input_filePath"=w182) -> ("output_Ivalid"=w180:bool, "output_data"=w178:i64[])  [unwired: 8 in]
                  n57 = To Unsigned Word Integer(number=w178) -> (unsigned 16bit integer=w177:u16[])
                  n58 = Select(t=w177, s=w180, f=w179) -> (s? t:f=w176:u16[])
                }
              }
              n59 = Select(t=myRIO_BRig_RT__Case_NonExp_stateList."UploadSettings_dataExp_1", s=w169, f=myRIO_BRig_RT__Case_NonExp_stateList."UploadSettings_Read_dataLC" ("t")) -> (s? t:f=w164:T1)
            }
            frame "UploadSettings_Read_dataLC" {
              # "grab dataLC and\nstore it in the\ngeneric data array"
              # "dataLC"
              n60 = call "myRIO_BRig_RT_dataLC_init_details.vi"() -> ("output_dataSize"=w189:i32, "output_dataName"=w192:string)  [unwired: 10 in]
              n61 = call "myRIO_BRig_RT_comm_webdav_uploadReceived_check.vi"("input_dataName"=w192) -> ("output_Iexist"=w191:bool, "output_dataPath"=w190:path)  [unwired: 9 in]
              n62 = case shown="True" w191 {
                tunnel: w190 -> [_ w201]
                tunnel: w189 -> [_ w200]
                tunnel: [_ w199] -> w188
                tunnel: w185 -> [w194 w198]
                tunnel: [w194 w195] -> w184
                frame False {
                }
                frame True {
                  n63 = call "myRIO_BRig_RT_comm_webdav_uploadReceived_read.vi"("input_dataSize"=w200, "input_filePath"=w201) -> ("output_Ivalid"=w199:bool, "output_data"=w197:i64[])  [unwired: 8 in]
                  n64 = To Unsigned Word Integer(number=w197) -> (unsigned 16bit integer=w196:u16[])
                  n65 = Select(t=w196, s=w199, f=w198) -> (s? t:f=w195:u16[])
                }
              }
              n66 = Select(t=myRIO_BRig_RT__Case_NonExp_stateList."UploadSettings_dataLC_1", s=w188, f=myRIO_BRig_RT__Case_NonExp_stateList."UploadSettings_Read_dataMTrig" ("t")) -> (s? t:f=w183:T1)
            }
            frame "UploadSettings_Read_dataMTrig" {
              # "grab dataMTrig and\nstore it in the\ngeneric data array"
              # "dataMTrig"
              n67 = call "myRIO_BRig_RT_dataMTrig_init_details.vi"() -> ("output_dataSize"=w208:i32, "output_dataName"=w211:string)  [unwired: 10 in]
              n68 = call "myRIO_BRig_RT_comm_webdav_uploadReceived_check.vi"("input_dataName"=w211) -> ("output_Iexist"=w210:bool, "output_dataPath"=w209:path)  [unwired: 9 in]
              n69 = case shown="True" w210 {
                tunnel: w209 -> [_ w220]
                tunnel: w208 -> [_ w219]
                tunnel: [_ w218] -> w207
                tunnel: w204 -> [w213 w217]
                tunnel: [w213 w214] -> w203
                frame False {
                }
                frame True {
                  n70 = call "myRIO_BRig_RT_comm_webdav_uploadReceived_read.vi"("input_dataSize"=w219, "input_filePath"=w220) -> ("output_Ivalid"=w218:bool, "output_data"=w216:i64[])  [unwired: 8 in]
                  n71 = To Unsigned Word Integer(number=w216) -> (unsigned 16bit integer=w215:u16[])
                  n72 = Select(t=w215, s=w218, f=w217) -> (s? t:f=w214:u16[])
                }
              }
              n73 = Select(t=myRIO_BRig_RT__Case_NonExp_stateList."UploadSettings_dataMTrig_1", s=w207, f=myRIO_BRig_RT__Case_NonExp_stateList."Idle" ("t")) -> (s? t:f=w202:T1)
            }
            frame "UploadSettings_dataExp_1" {
              w229 = 100.0 ("y")
              # "Freq"
              # "f_millisec2count"
              # "laser"
              # "Cue_max"
              # "Cue_min"
              # "CuePenalty"
              # "Timeout"
              # "Wrong"
              # "Selection"
              # "RewardPost"
              # "Reward_R"
              # "Reward_L"
              # "Tcycle"
              # "TPB_min_R"
              # "TPB_min_L"
              # "TPB_max_R"
              # "TPB_max_L"
              # "I_trialUntilReward"
              # "ENL_penalty"
              # "ENL_min"
              # "ENL_max"
              # "BUR_max"
              # "BUR_min"
              # "CueCycles"
              # "Audio_Freq_R"
              # "Audio_Freq_L"
              # "Audio_Amp_R"
              # "Audio_Amp_L"
              n74 = call "myRIO_BRig_RT_dataExp_laser_f_millisec2count.vi"() -> ("output_laser_f_millisec2count"=w243:i32)  [unwired: 11 in]
              n75 = call "myRIO_BRig_RT_dataExp_laser_Freq.vi"() -> ("output_laser_Freq"=w242:i32)  [unwired: 11 in]
              n76 = call "myRIO_BRig_RT_dataExp_CueCycles.vi"() -> ("output_CueCycles"=w289:i32)  [unwired: 11 in]
              n77 = call "myRIO_BRig_RT_dataExp_Audio_amp__R.vi"() -> ("output_Audio_amp__R"=w293:i32)  [unwired: 11 in]
              n78 = call "myRIO_BRig_RT_dataExp_Audio_amp__L.vi"() -> ("output_Audio_amp__L"=w295:i32)  [unwired: 11 in]
              n79 = call "myRIO_BRig_RT_dataExp_Tcycle_Reward__L.vi"() -> ("output_Tcycle_Reward__L"=w266:i32)  [unwired: 11 in]
              n80 = call "myRIO_BRig_RT_dataExp_Tcycle_Reward__R.vi"() -> ("output_Tcycle_Reward__R"=w265:i32)  [unwired: 11 in]
              n81 = call "myRIO_BRig_RT_dataExp_Tcycle_RewardPost.vi"() -> ("output_Tcycle_RewardPost"=w264:i32)  [unwired: 11 in]
              n82 = call "myRIO_BRig_RT_dataExp_BUR_min.vi"() -> ("output_BUR_min"=w286:i32)  [unwired: 11 in]
              n83 = call "myRIO_BRig_RT_dataExp_ENL_min.vi"() -> ("output_ENL_min"=w282:i32)  [unwired: 11 in]
              n84 = call "myRIO_BRig_RT_dataExp_TPB_max__L.vi"() -> ("output_TPB_max__L"=w274:i32)  [unwired: 11 in]
              n85 = call "myRIO_BRig_RT_dataExp_TPB_max__R.vi"() -> ("output_TPB_max__R"=w273:i32)  [unwired: 11 in]
              n86 = call "myRIO_BRig_RT_dataExp_ENL_penalty.vi"() -> ("output_ENL_penalty"=w281:i32)  [unwired: 11 in]
              n87 = call "myRIO_BRig_RT_dataExp_laser_Power_min.vi"() -> ("output_laser_Power_min"=w241:i32)  [unwired: 11 in]
              n88 = call "myRIO_BRig_RT_dataExp_laser_Tpeak.vi"() -> ("output_laser_Tpeak"=w240:i32)  [unwired: 11 in]
              n89 = call "myRIO_BRig_RT_dataExp_Audio_freq__L.vi"() -> ("output_Audio_freq__L"=w291:i32)  [unwired: 11 in]
              n90 = call "myRIO_BRig_RT_dataExp_Audio_freq__R.vi"() -> ("output_Audio_freq__R"=w290:i32)  [unwired: 11 in]
              n91 = call "myRIO_BRig_RT_dataExp_BUR_max.vi"() -> ("output_BUR_max"=w287:i32)  [unwired: 11 in]
              n92 = call "myRIO_BRig_RT_dataExp_ENL_max.vi"() -> ("output_ENL_max"=w283:i32)  [unwired: 11 in]
              n93 = call "myRIO_BRig_RT_dataExp_ItrialUntilReward.vi"() -> ("output_I_trialUntilReward"=w277:i32)  [unwired: 11 in]
              n94 = call "myRIO_BRig_RT_dataExp_Tcycle_Selection.vi"() -> ("output_Tcycle_Selection"=w263:i32)  [unwired: 11 in]
              n95 = call "myRIO_BRig_RT_dataExp_Tcycle_Wrong.vi"() -> ("output_Tcycle_Wrong"=w262:i32)  [unwired: 11 in]
              n96 = call "myRIO_BRig_RT_dataExp_Tcycle_Timeout.vi"() -> ("output_Tcycle_Timeout"=w261:i32)  [unwired: 11 in]
              n97 = call "myRIO_BRig_RT_dataExp_TPB_min__L.vi"() -> ("output_TPB_min__L"=w272:i32)  [unwired: 11 in]
              n98 = call "myRIO_BRig_RT_dataExp_TPB_min__R.vi"() -> ("output_TPB_min__R"=w271:i32)  [unwired: 11 in]
              n99 = call "myRIO_BRig_RT_dataExp_laser_Tshutter.vi"() -> ("output_laser_Tshutter"=w239:i32)  [unwired: 11 in]
              n100 = call "myRIO_BRig_RT_dataExp_laser_duration.vi"() -> ("output_laser_duration"=w238:i32)  [unwired: 11 in]
              n101 = call "myRIO_BRig_RT_dataExp_Tcycle_CuePenalty.vi"() -> ("output_Tcycle_CuePenalty"=w254:i32)  [unwired: 11 in]
              n102 = call "myRIO_BRig_RT_dataExp_Tcycle_Cue_min.vi"() -> ("output_Tcycle_Cue_min"=w253:i32)  [unwired: 11 in]
              n103 = call "myRIO_BRig_RT_dataExp_Tcycle_Cue_max.vi"() -> ("output_Tcycle_Cue_max"=w252:i32)  [unwired: 11 in]
              n104 = Index Array(array=w246, index #1=w295, index #2=w293, index #3=w291, index #4=w290, index #5=w289, index #6=w287, index #7=w286, index #8=w283, index #9=w282, index #10=w281, index #11=w277, index #12=w274, index #13=w273, index #14=w272, index #15=w271, index #16=w266, index #17=w265, index #18=w264, index #19=w263, index #20=w262, index #21=w261, index #22=w254, index #23=w253, index #24=w252, index #25=w243, index #26=w242, index #27=w241, index #28=w240, index #29=w239, index #30=w238) -> (element #1=w294:u16, element #2=w292:u16, element #3=w249:u16, element #4=w248:u16, element #5=w288:u16, element #6=w285:u16, element #7=w284:u16, element #8=w280:u16, element #9=w279:u16, element #10=w278:u16, element #11=w275:u16, element #12=w270:u16, element #13=w269:u16, element #14=w268:u16, element #15=w267:u16, element #16=w260:u16, element #17=w259:u16, element #18=w258:u16, element #19=w257:u16, element #20=w256:u16, element #21=w255:u16, element #22=w251:u16, element #23=w245:u16, element #24=w244:u16, element #25=w237:u16, element #26=w228:u16, element #27=w227:u16, element #28=w226:u16, element #29=w225:u16, element #30=w221:u16)
              n105 = To Double Precision Float(number=w237) -> (double precision float=w236:dbl)
              n106 = To Double Precision Float(number=w228) -> (double precision float=w234:dbl)
              n107 = To Double Precision Float(number=w227) -> (double precision float=w232:dbl)
              n108 = To Double Precision Float(number=w226) -> (double precision float=w231:dbl)
              n109 = To Double Precision Float(number=w225) -> (double precision float=w230:dbl)
              n110 = local write "Tcycle_Selection"(w257) -> ()
              n111 = local write "Tcycle_Wrong"(w256) -> ()
              n112 = local write "Tcycle_Timeout"(w255) -> ()
              n113 = local write "Audio_Amp__L"(w294) -> ()
              n114 = local write "Audio_Amp__R"(w292) -> ()
              n115 = Divide(x=w236, y=w229) -> (x/y=w235:dbl)
              n116 = Divide(x=w234, y=w229) -> (x/y=w233:dbl)
              n117 = Divide(x=w232, y=w229) -> (x/y=w224:dbl)
              n118 = Divide(x=w231, y=w229) -> (x/y=w223:dbl)
              n119 = Divide(x=w230, y=w229) -> (x/y=w222:dbl)
              n120 = local write "Tcycle_ENLPenalty"(w278) -> ()
              n121 = local write "Tcycle_ENL_max"(w280) -> ()
              n122 = local write "laser_duration"(w221) -> ()
              n123 = local write "TpB_Min_L"(w268) -> ()
              n124 = local write "TpB_Min_R"(w267) -> ()
              n125 = local write "laser_power_min"(w224) -> ()
              n126 = local write "f_millisec2count"(w235) -> ()
              n127 = local write "laser_Tshutter"(w222) -> ()
              n128 = local write "laser_Tpeak"(w223) -> ()
              n129 = local write "laser_Freq"(w233) -> ()
              n130 = local write "Tcycle_CuePenalty"(w251) -> ()
              n131 = local write "Tcycle_Cue_min"(w245) -> ()
              n132 = local write "Tcycle_Cue_max"(w244) -> ()
              n133 = To Unsigned Byte Integer(number=w249) -> (unsigned 8bit integer=w250:u8)
              n134 = To Unsigned Byte Integer(number=w248) -> (unsigned 8bit integer=w247:u8)
              n135 = Not Equal To 0?(x=w275) -> (x != 0?=w276:bool)
              n136 = local write "Tcycle_Reward_L"(w260) -> ()
              n137 = local write "Tcycle_Reward_R"(w259) -> ()
              n138 = local write "Tcycle_RewardPost"(w258) -> ()
              n139 = local write "CueCycles"(w288) -> ()
              n140 = local write "BUR_min"(w284) -> ()
              n141 = local write "BUR_max"(w285) -> ()
              n142 = local write "Tcycle_ENL_min"(w279) -> ()
              n143 = local write "TpB_Max_L"(w270) -> ()
              n144 = local write "TpB_Max_R"(w269) -> ()
              n145 = local write "TrialUntilReward"(w276) -> ()
              n146 = local write "Audio_Freq__L"(w250) -> ()
              n147 = local write "Audio_Freq__R"(w247) -> ()
            }
            frame "UploadSettings_dataLC_1" {
              # "Cue1_All_delayOpt"
              # "ENL1_All_delayOpt"
              # "Cue1_First_delayOpt"
              # "ENL1_First_delayOpt"
              # "ENL1 First"
              # "Cue1 All"
              # "Cue1 First"
              # "Count"
              # "Tdelay"
              # "Prob"
              # "OnOff"
              # "Block"
              # "ENL1 All"
              # "Count"
              # "Tdelay"
              # "Prob"
              # "OnOff"
              # "Block"
              # "Count"
              # "Tdelay"
              # "Prob"
              # "Block"
              # "OnOff"
              # "Count"
              # "Tdelay"
              # "Prob"
              # "OnOff"
              # "Block"
              n148 = call "myRIO_BRig_RT_dataLC_Cue1_First_Block.vi"() -> ("output_Cue1_First_Block"=w354:i32)  [unwired: 11 in]
              n149 = call "myRIO_BRig_RT_dataLC_Cue1_First_OnOff.vi"() -> ("output_Cue1_First_OnOff"=w352:i32)  [unwired: 11 in]
              n150 = call "myRIO_BRig_RT_dataLC_Cue1_First_Count.vi"() -> ("output_Cue1_First_Count"=w349:i32)  [unwired: 11 in]
              n151 = call "myRIO_BRig_RT_dataLC_Cue1_All_Block.vi"() -> ("output_Cue1_All_Block"=w336:i32)  [unwired: 11 in]
              n152 = call "myRIO_BRig_RT_dataLC_Cue1_All_OnOff.vi"() -> ("output_Cue1_All_OnOff"=w335:i32)  [unwired: 11 in]
              n153 = call "myRIO_BRig_RT_dataLC_Cue1_All_Count.vi"() -> ("output_Cue1_All_Count"=w346:i32)  [unwired: 11 in]
              n154 = call "myRIO_BRig_RT_dataLC_ENL1_First_Block.vi"() -> ("output_ENL1_First_Block"=w334:i32)  [unwired: 11 in]
              n155 = call "myRIO_BRig_RT_dataLC_ENL1_First_OnOff.vi"() -> ("output_ENL1_First_OnOff"=w345:i32)  [unwired: 11 in]
              n156 = call "myRIO_BRig_RT_dataLC_ENL1_First_Count.vi"() -> ("output_ENL1_First_Count"=w342:i32)  [unwired: 11 in]
              n157 = call "myRIO_BRig_RT_dataLC_ENL1_All_Block.vi"() -> ("output_ENL1_All_Block"=w341:i32)  [unwired: 11 in]
              n158 = call "myRIO_BRig_RT_dataLC_ENL1_All_OnOff.vi"() -> ("output_ENL1_All_OnOff"=w340:i32)  [unwired: 11 in]
              n159 = call "myRIO_BRig_RT_dataLC_ENL1_All_Count.vi"() -> ("output_ENL1_All_Count"=w337:i32)  [unwired: 11 in]
              n160 = call "myRIO_BRig_RT_dataLC_ENL1_First_delayOpt.vi"() -> ("output_ENL1_First_delayOpt"=w311:i32)  [unwired: 11 in]
              n161 = call "myRIO_BRig_RT_dataLC_Cue1_First_delayOpt.vi"() -> ("output_Cue1_First_delayOpt"=w310:i32)  [unwired: 11 in]
              n162 = call "myRIO_BRig_RT_dataLC_ENL1_All_delayOpt.vi"() -> ("output_ENL1_All_delayOpt"=w303:i32)  [unwired: 11 in]
              n163 = call "myRIO_BRig_RT_dataLC_Cue1_All_delayOpt.vi"() -> ("output_Cue1_All_delayOpt"=w302:i32)  [unwired: 11 in]
              n164 = call "myRIO_BRig_RT_dataLC_Cue1_First_Probability.vi"() -> ("output_Cue1_First_Probability"=w351:i32)  [unwired: 11 in]
              n165 = call "myRIO_BRig_RT_dataLC_Cue1_First_Tdelay.vi"() -> ("output_Cue1_First_Tdelay"=w350:i32)  [unwired: 11 in]
              n166 = call "myRIO_BRig_RT_dataLC_Cue1_All_Probability.vi"() -> ("output_Cue1_All_Probability"=w348:i32)  [unwired: 11 in]
              n167 = call "myRIO_BRig_RT_dataLC_Cue1_All_Tdelay.vi"() -> ("output_Cue1_All_Tdelay"=w347:i32)  [unwired: 11 in]
              n168 = call "myRIO_BRig_RT_dataLC_ENL1_First_Probability.vi"() -> ("output_ENL1_First_Probability"=w344:i32)  [unwired: 11 in]
              n169 = call "myRIO_BRig_RT_dataLC_ENL1_First_Tdelay.vi"() -> ("output_ENL1_First_Tdelay"=w343:i32)  [unwired: 11 in]
              n170 = call "myRIO_BRig_RT_dataLC_ENL1_All_Probability.vi"() -> ("output_ENL1_All_Probability"=w339:i32)  [unwired: 11 in]
              n171 = call "myRIO_BRig_RT_dataLC_ENL1_All_Tdelay.vi"() -> ("output_ENL1_All_Tdelay"=w338:i32)  [unwired: 11 in]
              n172 = Index Array(array=w312, index #1=w354, index #2=w352, index #3=w351, index #4=w350, index #5=w349, index #6=w336, index #7=w335, index #8=w348, index #9=w347, index #10=w346, index #11=w334, index #12=w345, index #13=w344, index #14=w343, index #15=w342, index #16=w341, index #17=w340, index #18=w339, index #19=w338, index #20=w337, index #21=w311, index #22=w310, index #23=w303, index #24=w302) -> (element #1=w353:u16, element #2=w332:u16, element #3=w331:u16, element #4=w330:u16, element #5=w329:u16, element #6=w325:u16, element #7=w324:u16, element #8=w323:u16, element #9=w322:u16, element #10=w321:u16, element #11=w320:u16, element #12=w319:u16, element #13=w318:u16, element #14=w317:u16, element #15=w304:u16, element #16=w316:u16, element #17=w315:u16, element #18=w314:u16, element #19=w313:u16, element #20=w305:u16, element #21=w308:u16, element #22=w306:u16, element #23=w299:u16, element #24=w298:u16)
              n173 = Not Equal To 0?(x=w299) -> (x != 0?=w301:bool)
              n174 = Not Equal To 0?(x=w298) -> (x != 0?=w300:bool)
              n175 = Not Equal To 0?(x=w308) -> (x != 0?=w309:bool)
              n176 = Not Equal To 0?(x=w306) -> (x != 0?=w307:bool)
              n177 = Not Equal To 0?(x=w332) -> (x != 0?=w333:bool)
              n178 = Not Equal To 0?(x=w324) -> (x != 0?=w328:bool)
              n179 = Not Equal To 0?(x=w319) -> (x != 0?=w327:bool)
              n180 = Not Equal To 0?(x=w315) -> (x != 0?=w326:bool)
              n181 = local write "LC_Cue1_First_Probability"(w331) -> ()
              n182 = local write "LC_ENL1_First_Probability"(w318) -> ()
              n183 = local write "LC_ENL1_First_delayOpt"(w309) -> ()
              n184 = local write "LC_Cue1_First_delayOpt"(w307) -> ()
              n185 = local write "LC_ENL1_All_delayOpt"(w301) -> ()
              n186 = local write "LC_Cue1_All_delayOpt"(w300) -> ()
              n187 = local write "LC_Cue1_All_Probability"(w323) -> ()
              n188 = local write "LC_Cue1_First_Tdelay"(w330) -> ()
              n189 = local write "LC_ENL1_All_Probability"(w314) -> ()
              n190 = local write "LC_Cue1_First_OnOff"(w333) -> ()
              n191 = local write "LC_Cue1_First_Count"(w329) -> ()
              n192 = local write "LC_Cue1_First_Block"(w353) -> ()
              n193 = local write "LC_ENL1_First_Tdelay"(w317) -> ()
              n194 = local write "LC_ENL1_First_OnOff"(w327) -> ()
              n195 = local write "LC_ENL1_First_Count"(w304) -> ()
              n196 = local write "LC_ENL1_First_Block"(w320) -> ()
              n197 = local write "LC_Cue1_All_Tdelay"(w322) -> ()
              n198 = local write "LC_Cue1_All_OnOff"(w328) -> ()
              n199 = local write "LC_Cue1_All_Count"(w321) -> ()
              n200 = local write "LC_Cue1_All_Block"(w325) -> ()
              n201 = local write "LC_ENL1_All_Tdelay"(w313) -> ()
              n202 = local write "LC_ENL1_All_OnOff"(w326) -> ()
              n203 = local write "LC_ENL1_All_Count"(w305) -> ()
              n204 = local write "LC_ENL1_All_Block"(w316) -> ()
            }
            frame "UploadSettings_dataLC_2" {
              # "Wrong"
              # "Reward"
              # "Trial"
              # "Tdelay"
              # "Prob"
              # "Block"
              # "OnOff"
              # "Trial"
              # "Tdelay"
              # "Prob"
              # "OnOff"
              # "Block"
              n205 = call "myRIO_BRig_RT_dataLC_Reward_Block.vi"() -> ("output_Reward_Block"=w379:i32)  [unwired: 11 in]
              n206 = call "myRIO_BRig_RT_dataLC_Reward_OnOff.vi"() -> ("output_Reward_OnOff"=w377:i32)  [unwired: 11 in]
              n207 = call "myRIO_BRig_RT_dataLC_Reward_Trial.vi"() -> ("output_Reward_Trial"=w374:i32)  [unwired: 11 in]
              n208 = call "myRIO_BRig_RT_dataLC_Wrong_Block.vi"() -> ("output_Wrong_Block"=w370:i32)  [unwired: 11 in]
              n209 = call "myRIO_BRig_RT_dataLC_Wrong_OnOff.vi"() -> ("output_Wrong_OnOff"=w369:i32)  [unwired: 11 in]
              n210 = call "myRIO_BRig_RT_dataLC_Wrong_Trial.vi"() -> ("output_Wrong_Trial"=w371:i32)  [unwired: 11 in]
              n211 = call "myRIO_BRig_RT_dataLC_Reward_Probability.vi"() -> ("output_Reward_Probability"=w376:i32)  [unwired: 11 in]
              n212 = call "myRIO_BRig_RT_dataLC_Reward_Tdelay.vi"() -> ("output_Reward_Tdelay"=w375:i32)  [unwired: 11 in]
              n213 = call "myRIO_BRig_RT_dataLC_Wrong_Probability.vi"() -> ("output_Wrong_Probability"=w373:i32)  [unwired: 11 in]
              n214 = call "myRIO_BRig_RT_dataLC_Wrong_Tdelay.vi"() -> ("output_Wrong_Tdelay"=w372:i32)  [unwired: 11 in]
              n215 = Index Array(array=w357, index #1=w379, index #2=w377, index #3=w376, index #4=w375, index #5=w374, index #6=w370, index #7=w369, index #8=w373, index #9=w372, index #10=w371) -> (element #1=w378:u16, element #2=w367:u16, element #3=w366:u16, element #4=w365:u16, element #5=w364:u16, element #6=w362:u16, element #7=w361:u16, element #8=w360:u16, element #9=w359:u16, element #10=w358:u16)
              n216 = Not Equal To 0?(x=w367) -> (x != 0?=w368:bool)
              n217 = Not Equal To 0?(x=w361) -> (x != 0?=w363:bool)
              n218 = local write "LC_Reward_Probability"(w366) -> ()
              n219 = local write "LC_Wrong_Probability"(w360) -> ()
              n220 = local write "LC_Reward_Tdelay"(w365) -> ()
              n221 = local write "LC_Reward_OnOff"(w368) -> ()
              n222 = local write "LC_Reward_Block"(w378) -> ()
              n223 = local write "LC_Reward_Trial"(w364) -> ()
              n224 = local write "LC_Wrong_Tdelay"(w359) -> ()
              n225 = local write "LC_Wrong_OnOff"(w363) -> ()
              n226 = local write "LC_Wrong_Block"(w362) -> ()
              n227 = local write "LC_Wrong_Trial"(w358) -> ()
            }
            frame "UploadSettings_dataMTrig_1" {
              # "Tdelay_R"
              # "Tdelay_L"
              # "Tcycle_R"
              # "Tcycle_L"
              # "RewCalib_nCycle_R"
              # "RewCalib_nCycle_L"
              # "Solenoid"
              # "Laser_Tcycle"
              n228 = call "myRIO_BRig_RT_dataMTrig_Laser_Tcycle.vi"() -> ("output_Laser_Tcycle"=w389:i32)  [unwired: 11 in]
              n229 = call "myRIO_BRig_RT_dataMTrig_Solenoid_RewCalib_nCycle__L.vi"() -> ("output_Solenoid_RewCalib_nCycle__L"=w388:i32)  [unwired: 11 in]
              n230 = call "myRIO_BRig_RT_dataMTrig_Solenoid_RewCalib_nCycle__R.vi"() -> ("output_Solenoid_RewCalib_nCycle__R"=w387:i32)  [unwired: 11 in]
              n231 = call "myRIO_BRig_RT_dataMTrig_Solenoid_Tdelay__L.vi"() -> ("output_Solenoid_Tdelay__L"=w384:i32)  [unwired: 11 in]
              n232 = call "myRIO_BRig_RT_dataMTrig_Solenoid_Tdelay__R.vi"() -> ("output_Solenoid_Tdelay__R"=w383:i32)  [unwired: 11 in]
              n233 = call "myRIO_BRig_RT_dataMTrig_Solenoid_Tcycle__L.vi"() -> ("output_Solenoid_Tcycle__L"=w386:i32)  [unwired: 11 in]
              n234 = call "myRIO_BRig_RT_dataMTrig_Solenoid_Tcycle__R.vi"() -> ("output_Solenoid_Tcycle__R"=w385:i32)  [unwired: 11 in]
              n235 = Index Array(array=w382, index #1=w389, index #2=w388, index #3=w387, index #4=w386, index #5=w385, index #6=w384, index #7=w383) -> (element #1=w396:u16, element #2=w395:u16, element #3=w394:u16, element #4=w393:u16, element #5=w392:u16, element #6=w391:u16, element #7=w390:u16)
              n236 = Replace Array Subset(array=w398, new element #1=w396, index #1=w389, new element #2=w395, index #2=w388, new element #3=w394, index #3=w387, new element #4=w393, index #4=w386, new element #5=w392, index #5=w385, new element #6=w391, index #6=w384, new element #7=w390, index #7=w383) -> (w397:u16[])
              n237 = local write "MTrig_Solenoid_Tcycle__L"(w393) -> ()
              n238 = local write "MTrig_Solenoid_Tcycle__R"(w392) -> ()
              n239 = local write "MTrig_Laser_Tcycle"(w396) -> ()
            }
            frame "Idle" {
              # "To ensure timing, we split the\nidle state into 4 phases"
              # "Laser_Tcycle"
              # "Audio_Tcycle_R"
              # "Audio_Tcycle_L"
              n240 = local read "laser_power_min"() -> (w401:dbl)
              n241 = local read "f_millisec2count"() -> (w409:dbl)
              n242 = local read "Audio_Amp__R"() -> (w403:u16)
              n243 = local read "Audio_Amp__L"() -> (w405:u16)
              n244 = local read "Audio_Freq__R"() -> (w402:u8)
              n245 = local read "Audio_Freq__L"() -> (w404:u8)
              n246 = local read "MTrig_Audio_trig__L"() -> (w417:bool)
              n247 = local read "MTrig_Audio_trig__R"() -> (w419:bool)
              n248 = Select(t=myRIO_BRig_RT__Case_NonExp_stateList."SendData" ("Enum"), s="SendData", f=myRIO_BRig_RT__Case_NonExp_stateList."Idle_2" ("Enum")) -> (s? t:f=w412:T1)
              n249 = call "myRIO__convert__Voltage_to_FPGAvalue.vi"("input_voltage"=w401) -> ("output_PortC"=w400:i16)  [unwired: 9 in, 1 out]
              n250 = local read "MTrig_Laser_trig"() -> (w418:bool)
              n251 = To Unsigned Word Integer(number=w409) -> (unsigned 16bit integer=w408:u16)
              n252 = call "myRIO_BRig_RT_dataMTrig_Audio_Tcycle__L.vi"() -> ("output_Audio_Tcycle__L"=w428:i32)  [unwired: 11 in]
              n253 = call "myRIO_BRig_RT_dataMTrig_Audio_Tcycle__R.vi"() -> ("output_Audio_Tcycle__R"=w427:i32)  [unwired: 11 in]
              n254 = call "myRIO_BRig_RT_dataMTrig_Laser_Tcycle.vi"() -> ("output_Laser_Tcycle"=w426:i32)  [unwired: 11 in]
              n255 = local read "MTrig_Laser_Tcycle"() -> (w410:u16)
              n256 = xnode "Read/Write Control"("FPGA VI Reference In"=w407, "error in"=w406, "k1__counter_per_ms"=w408, "audioAmp_L"=w405, "audioFreq_L_kHz"=w404, "audioAmp_R"=w403, "audioFreq_R_kHz"=w402, "AnaOut_0"=w400) -> ()  [unwired: 2 out]
              n257 = Select(t=myRIO_BRig_RT__Case_NonExp_stateList."TestConnection" ("Enum"), s="TestConnection", f=w412) -> (s? t:f=w421:T1)
              n258 = local read "Tcycle_Cue_min"() -> (w411:u16)
              n259 = Compound Arithmetic op=OR(w417, w419, w418) -> (w420:bool)
              n260 = case shown="True" w420 {
                frame False {
                }
                frame True {
                  w429 = FALSE
                  n261 = local write "MTrig_Audio_trig__L"(w429) -> ()
                  n262 = local write "MTrig_Audio_trig__R"(w429) -> ()
                  n263 = local write "MTrig_Laser_trig"(w429) -> ()
                }
              }
              n264 = Replace Array Subset(array=w424, new element #1=w411, index #1=w428, new element #2=w411, index #2=w427, new element #3=w410, index #3=w426) -> (w425:u16[])
            }
            frame "Idle_2" {
              w431 = u16 0 ("t")
              # "To ensure timing, we split the\nidle state into 4 phases"
              # "Ncycles"
              # "Ncycles"
              # "RewCalib"
              # "RewCalib"
              # "Solenoid R"
              # "Solenoid L"
              n265 = call "myRIO_BRig_RT_dataMTrig_Solenoid_RewCalib_OnOff__L.vi"() -> ("output_Solenoid_RewCalib_OnOff__L"=w462:i32)  [unwired: 11 in]
              n266 = call "myRIO_BRig_RT_dataMTrig_Solenoid_N__L.vi"() -> ("output_Solenoid_N__L"=w450:i32)  [unwired: 11 in]
              n267 = call "myRIO_BRig_RT_dataMTrig_Solenoid_RewCalib_OnOff__R.vi"() -> ("output_Solenoid_RewCalib_OnOff__R"=w447:i32)  [unwired: 11 in]
              n268 = call "myRIO_BRig_RT_dataMTrig_Solenoid_N__R.vi"() -> ("output_Solenoid_N__R"=w446:i32)  [unwired: 11 in]
              n269 = Index Array(array=w453, index #1=w462, index #2=w450, index #3=w447, index #4=w446) -> (element #1=w449:u16, element #2=w444:u16, element #3=w445:u16, element #4=w443:u16)
              n270 = local read "RewCalib_Trig_L"() -> (w442:bool)
              n271 = local read "RewCalib_Trig_R"() -> (w441:bool)
              n272 = Equal To 0?(x=w444) -> (x = 0?=w452:bool)
              n273 = Equal To 0?(x=w443) -> (x = 0?=w451:bool)
              n274 = Not Equal To 0?(x=w445) -> (x != 0?=w463:bool)
              n275 = Not Equal To 0?(x=w449) -> (x != 0?=w464:bool)
              n276 = And(x=w452, y=w451) -> (x .and. y?=w456:bool)
              n277 = Or(x=w442, y=w441) -> (x .or. y?=w457:bool)
              n278 = Not Exclusive Or(1:w464, 2:w442) -> (0:w459:bool)
              n279 = Not Exclusive Or(1:w463, 2:w441) -> (0:w461:bool)
              n280 = And(x=w457, y=w456) -> (x .and. y?=w439:bool)
              n281 = Not(x=w459) -> (.not. x?=w458:bool)
              n282 = Not(x=w461) -> (.not. x?=w460:bool)
              n283 = Or(x=w458, y=w460) -> (x .or. y?=w440:bool)
              n284 = Or(x=w439, y=w440) -> (x .or. y?=w455:bool)
              n285 = local read "count_warmup_R"() -> (w430:u16)
              n286 = local read "count_warmup_L"() -> (w435:u16)
              n287 = Select(t=myRIO_BRig_RT__Case_NonExp_stateList."RewardCalibration_pre" ("Enum"), s=w455, f=myRIO_BRig_RT__Case_NonExp_stateList."Idle_3" ("Enum")) -> (s? t:f=w438:T1)
              n288 = Select(t=w431, s="count_warmup_L_reset", f=w435) -> (s? t:f=→"count_warmup_L":u16)
              n289 = Select(t=w431, s="count_warmup_R_reset", f=w430) -> (s? t:f=→"count_warmup_R":u16)
            }
            frame "Idle_3" {
              w487 = u8 0 ("f")
              # "To ensure timing, we split the\nidle state into 4 phases"
              n290 = local read "MTrig_Solenoid_trig__L"() -> (w478:bool)
              n291 = local read "MTrig_Solenoid_trig__R"() -> (w488:bool)
              n292 = local read "warmupType"() -> (w470:u8)
              n293 = local read "warmup"() -> (w480:bool)
              n294 = Not Equal To 0?(x=w470) -> (x != 0?=w469:bool)
              n295 = Not(x=w469) -> (.not. x?=w481:bool)
              n296 = Select(t=u8 1, s=w478, f=w487) -> (s? t:f=w486:u8)
              n297 = Select(t=u8 2, s=w488, f=w487) -> (s? t:f=w485:u8)
              n298 = And(x=w480, y=w481) -> (x .and. y?=w479:bool)
              n299 = And(x=w480, y=w469) -> (x .and. y?=w474:bool)
              n300 = Add(x=w486, y=w485) -> (x+y=w484:u8)
              n301 = case shown="3" w484 {
                tunnel: w483 -> [w491 w495 w513 w531]
                tunnel: [w491 w494 w512 w530] -> w482
                tunnel: w479 -> [_ w493 w511 w529]
                tunnel: [_ TRUE TRUE TRUE] -> w476
                frame 0, Default {
                }
                frame 1 {
                  n302 = case shown="True" w493 {
                    tunnel: w495 -> [w504 w509]
                    tunnel: [w503 w508] -> w494
                    frame True {
                      # "Audio_L"
                      # "Solenoid_L"
                      n303 = call "myRIO_BRig_RT_dataMTrig_Solenoid_N__L.vi"() -> ("output_Solenoid_N__L"=w500:i32)  [unwired: 11 in]
                      n304 = call "myRIO_BRig_RT_dataMTrig_Audio_N__L.vi"() -> ("output_Audio_N__L"=w498:i32)  [unwired: 11 in]
                      n305 = Index Array(array=w504, index #1=w500, index #2=w498) -> (element #1=w502:u16, element #2=w501:u16)
                      n306 = Increment(x=w502) -> (x+1=w499:u16)
                      n307 = Increment(x=w501) -> (x+1=w497:u16)
                      n308 = Replace Array Subset(array=w504, new element #1=w499, index #1=w500, new element #2=w497, index #2=w498) -> (w503:u16[])
                    }
                    frame False {
                      # "Solenoid_L"
                      n309 = call "myRIO_BRig_RT_dataMTrig_Solenoid_N__L.vi"() -> ("output_Solenoid_N__L"=w506:i32)  [unwired: 11 in]
                      n310 = Index Array(array=w509, index=w506) -> (element=w507:u16)
                      n311 = Increment(x=w507) -> (x+1=w505:u16)
                      n312 = Replace Array Subset(array=w509, new element=w505, index=w506) -> (w508:u16[])
                    }
                  }
                  n313 = local write "MTrig_Solenoid_trig__L"(FALSE) -> ()
                }
                frame 2 {
                  n314 = case shown="True" w511 {
                    tunnel: w513 -> [w522 w527]
                    tunnel: [w521 w526] -> w512
                    frame True {
                      # "Audio_R"
                      # "Solenoid_R"
                      n315 = call "myRIO_BRig_RT_dataMTrig_Solenoid_N__R.vi"() -> ("output_Solenoid_N__R"=w518:i32)  [unwired: 11 in]
                      n316 = call "myRIO_BRig_RT_dataMTrig_Audio_N__R.vi"() -> ("output_Audio_N__R"=w517:i32)  [unwired: 11 in]
                      n317 = Index Array(array=w522, index #1=w518, index #2=w517) -> (element #1=w520:u16, element #2=w519:u16)
                      n318 = Increment(x=w519) -> (x+1=w515:u16)
                      n319 = Increment(x=w520) -> (x+1=w516:u16)
                      n320 = Replace Array Subset(array=w522, new element #1=w516, index #1=w518, new element #2=w515, index #2=w517) -> (w521:u16[])
                    }
                    frame False {
                      # "Solenoid_R"
                      n321 = call "myRIO_BRig_RT_dataMTrig_Solenoid_N__R.vi"() -> ("output_Solenoid_N__R"=w523:i32)  [unwired: 11 in]
                      n322 = Index Array(array=w527, index=w523) -> (element=w525:u16)
                      n323 = Increment(x=w525) -> (x+1=w524:u16)
                      n324 = Replace Array Subset(array=w527, new element=w524, index=w523) -> (w526:u16[])
                    }
                  }
                  n325 = local write "MTrig_Solenoid_trig__R"(FALSE) -> ()
                }
                frame 3 {
                  w532 = FALSE
                  n326 = case shown="True" w529 {
                    tunnel: w531 -> [w546 w554]
                    tunnel: [w545 w553] -> w530
                    frame True {
                      # "Audio_R"
                      # "Solenoid_R"
                      # "Audio_L"
                      # "Solenoid_L"
                      n327 = call "myRIO_BRig_RT_dataMTrig_Solenoid_N__L.vi"() -> ("output_Solenoid_N__L"=w540:i32)  [unwired: 11 in]
                      n328 = call "myRIO_BRig_RT_dataMTrig_Audio_N__L.vi"() -> ("output_Audio_N__L"=w538:i32)  [unwired: 11 in]
                      n329 = call "myRIO_BRig_RT_dataMTrig_Solenoid_N__R.vi"() -> ("output_Solenoid_N__R"=w536:i32)  [unwired: 11 in]
                      n330 = call "myRIO_BRig_RT_dataMTrig_Audio_N__R.vi"() -> ("output_Audio_N__R"=w535:i32)  [unwired: 11 in]
                      n331 = Index Array(array=w546, index #1=w540, index #2=w538, index #3=w536, index #4=w535) -> (element #1=w544:u16, element #2=w543:u16, element #3=w542:u16, element #4=w541:u16)
                      n332 = Increment(x=w541) -> (x+1=w533:u16)
                      n333 = Increment(x=w544) -> (x+1=w539:u16)
                      n334 = Increment(x=w543) -> (x+1=w537:u16)
                      n335 = Increment(x=w542) -> (x+1=w534:u16)
                      n336 = Replace Array Subset(array=w546, new element #1=w539, index #1=w540, new element #2=w537, index #2=w538, new element #3=w534, index #3=w536, new element #4=w533, index #4=w535) -> (w545:u16[])
                    }
                    frame False {
                      # "Solenoid_R"
                      # "Solenoid_L"
                      n337 = call "myRIO_BRig_RT_dataMTrig_Solenoid_N__L.vi"() -> ("output_Solenoid_N__L"=w550:i32)  [unwired: 11 in]
                      n338 = call "myRIO_BRig_RT_dataMTrig_Solenoid_N__R.vi"() -> ("output_Solenoid_N__R"=w547:i32)  [unwired: 11 in]
                      n339 = Index Array(array=w554, index #1=w550, index #2=w547) -> (element #1=w552:u16, element #2=w551:u16)
                      n340 = Increment(x=w552) -> (x+1=w549:u16)
                      n341 = Increment(x=w551) -> (x+1=w548:u16)
                      n342 = Replace Array Subset(array=w554, new element #1=w549, index #1=w550, new element #2=w548, index #2=w547) -> (w553:u16[])
                    }
                  }
                  n343 = local write "MTrig_Solenoid_trig__L"(w532) -> ()
                  n344 = local write "MTrig_Solenoid_trig__R"(w532) -> ()
                }
              }
              n345 = local read "get_countPerMS"() -> (w468:bool)
              n346 = Select(t=myRIO_BRig_RT__Case_NonExp_stateList."Get_FPGA_count_per_ms" ("Enum"), s=w468, f=myRIO_BRig_RT__Case_NonExp_stateList."Idle_4" ("Enum")) -> (s? t:f=w466:T1)
              n347 = Select(t=myRIO_BRig_RT__Case_NonExp_stateList."Cue_pre", s=w474, f=myRIO_BRig_RT__Case_NonExp_stateList."DispenseWater_pre" ("Enum")) -> (s? t:f=w472:T1)
              n348 = Select(t=w472, s=w476, f=w466) -> (s? t:f=w477:T1)
            }
            frame "Idle_4" {
              # "use dataMTrig as it is one of the last to transfer"
              # "To ensure timing, we split the\nidle state into 4 phases"
              n349 = call "myRIO_BRig_RT_comm_webdav_uploadReceived_check_v2,0.vi"("input_dataName"="dataMTrig") -> ("output_Iexist"=w560:bool)  [unwired: 9 in, 1 out]
              n350 = Select(t=myRIO_BRig_RT__Case_NonExp_stateList."UploadSettings_pre" ("Enum"), s=w560, f=myRIO_BRig_RT__Case_NonExp_stateList."Idle") -> (s? t:f=w558:T1)
            }
            frame "Cue_pre" {
              w570 = u16 1 ("t")
              w569 = u16 0 ("new element/subarray")
              w566 = u16 0 ("new element/subarray")
              # "Ncycle"
              # "count"
              # "Audio_R"
              # "Solenoid_R"
              # "Solenoid_L"
              # "Ncycle"
              # "count"
              # "Audio_L"
              n351 = call "myRIO_BRig_RT_dataMTrig_Solenoid_N__L.vi"() -> ("output_Solenoid_N__L"=w579:i32)  [unwired: 11 in]
              n352 = call "myRIO_BRig_RT_dataMTrig_Solenoid_N__R.vi"() -> ("output_Solenoid_N__R"=w578:i32)  [unwired: 11 in]
              n353 = Index Array(array=w575, index #1=w579, index #2=w578) -> (element #1=w577:u16, element #2=w576:u16)
              n354 = Not Equal To 0?(x=w576) -> (x != 0?=w562:bool)
              n355 = Not Equal To 0?(x=w577) -> (x != 0?=w563:bool)
              n356 = Select(t=w570, s=w563, f=w569) -> (s? t:f=w571:u16)
              n357 = Select(t=w570, s=w562, f=w569) -> (s? t:f=w565:u16)
              n358 = call "myRIO_BRig_RT_dataMTrig_Audio_c__L.vi"() -> ("output_Audio_c__L"=w573:i32)  [unwired: 11 in]
              n359 = call "myRIO_BRig_RT_dataMTrig_Audio_N__L.vi"() -> ("output_Audio_N__L"=w572:i32)  [unwired: 11 in]
              n360 = call "myRIO_BRig_RT_dataMTrig_Audio_c__R.vi"() -> ("output_Audio_c__R"=w568:i32)  [unwired: 11 in]
              n361 = call "myRIO_BRig_RT_dataMTrig_Audio_N__R.vi"() -> ("output_Audio_N__R"=w567:i32)  [unwired: 11 in]
              n362 = Replace Array Subset(array=w575, new element #1=w566, index #1=w573, new element #2=w571, index #2=w572, new element #3=w566, index #3=w568, new element #4=w565, index #4=w567) -> (w574:u16[])
            }
            frame "Cue" {
              # "lick did not occur or warmupType==1"
              # "lick occurred?"
              # "Ncycle"
              # "Audio_R"
              # "Ncycle"
              # "Audio_L"
              n363 = local read "warmupType"() -> (w589:u8)
              n364 = Greater?(x=w595, y=w594) -> (0:w598:bool)
              n365 = Greater?(x=w597, y=w596) -> (0:w593:bool)
              n366 = Or(x=w593, y=w598) -> (x .or. y?=w587:bool)
              n367 = Equal?(x=w589, y=u8 1) -> (x = y?=w583:bool)
              n368 = Not(x=w587) -> (.not. x?=w586:bool)
              n369 = call "myRIO_BRig_RT_dataMTrig_Audio_N__L.vi"() -> ("output_Audio_N__L"=w601:i32)  [unwired: 11 in]
              n370 = call "myRIO_BRig_RT_dataMTrig_Audio_N__R.vi"() -> ("output_Audio_N__R"=w600:i32)  [unwired: 11 in]
              n371 = Or(x=w586, y=w583) -> (x .or. y?=w584:bool)
              n372 = case shown="True" w584 {
                tunnel: w601 -> [w607 w625]
                tunnel: w600 -> [w606 w624]
                tunnel: w592 -> [w609 w619]
                tunnel: [w608 w619] -> w591
                tunnel: w590 -> [_ w617]
                tunnel: [myRIO_BRig_RT__Case_NonExp_stateList."Idle" ("t") w616] -> w585
                tunnel: w583 -> [_ w615]
                tunnel: w582 -> [_ w611]
                tunnel: w581 -> [_ w610]
                frame False {
                  w602 = u16 0 ("new element/subarray")
                  # "lick occurred and warmupType==2"
                  n373 = call "myRIO_BRig_RT_dataMTrig_Solenoid_N__R.vi"() -> ("output_Solenoid_N__R"=w603:i32)  [unwired: 11 in]
                  n374 = call "myRIO_BRig_RT_dataMTrig_Solenoid_N__L.vi"() -> ("output_Solenoid_N__L"=w604:i32)  [unwired: 11 in]
                  n375 = Replace Array Subset(array=w609, new element #1=w602, index #1=w607, new element #2=w602, index #2=w606, new element #3=w602, index #3=w604, new element #4=w602, index #4=w603) -> (w608:u16[])
                }
                frame True {
                  n376 = Not(x=w615) -> (.not. x?=w614:bool)
                  n377 = Index Array(array=w619, index #1=w625, index #2=w624) -> (element #1=w623:u16, element #2=w622:u16)
                  n378 = Equal To 0?(x=w623) -> (x = 0?=w621:bool)
                  n379 = Equal To 0?(x=w622) -> (x = 0?=w620:bool)
                  n380 = And(x=w621, y=w620) -> (x .and. y?=w613:bool)
                  n381 = And(x=w613, y=w614) -> (x .and. y?=w612:bool)
                  n382 = case shown="True" w612 {
                    tunnel: w611 -> [_ w633]
                    tunnel: w610 -> [_ w628]
                    frame False {
                    }
                    frame True {
                      n383 = local read "count_warmup_R"() -> (w626:u16)
                      n384 = local read "count_warmup_L"() -> (w631:u16)
                      n385 = Increment(x=w626) -> (x+1=w629:u16)
                      n386 = Increment(x=w631) -> (x+1=w632:u16)
                      n387 = Select(t=w629, s=w628, f=w626) -> (s? t:f=w627:u16)
                      n388 = Select(t=w632, s=w633, f=w631) -> (s? t:f=w630:u16)
                      n389 = local write "count_warmup_R"(w627) -> ()
                      n390 = local write "count_warmup_L"(w630) -> ()
                    }
                  }
                  n391 = Select(t=myRIO_BRig_RT__Case_NonExp_stateList."DispenseWater_pre", s=w613, f=w617) -> (s? t:f=w616:T1)
                }
              }
            }
            frame "RewardCalibration_pre" {
              (unwired) FALSE
              w635 = FALSE
              w646 = u8 0
              w662 = u8 0
              # "Are we starting a RewardCalibration?\nOr are we stopping a RewardCalibration?\nOr is a RewardCalibration over?"
              # "RewCalib\nOnOff"
              # "N"
              # "Solenoid R"
              # "RewCalib\nOnOff"
              # "N"
              # "Solenoid L"
              n392 = local read "RewCalib_Trig_L"() -> (w669:bool)
              n393 = local read "RewCalib_Trig_R"() -> (w638:bool)
              n394 = call "myRIO_BRig_RT_dataMTrig_Solenoid_N__R.vi"() -> ("output_Solenoid_N__R"=w640:i32)  [unwired: 11 in]
              n395 = call "myRIO_BRig_RT_dataMTrig_Solenoid_RewCalib_OnOff__R.vi"() -> ("output_Solenoid_RewCalib_OnOff__R"=w637:i32)  [unwired: 11 in]
              n396 = call "myRIO_BRig_RT_dataMTrig_Solenoid_N__L.vi"() -> ("output_Solenoid_N__L"=w655:i32)  [unwired: 11 in]
              n397 = call "myRIO_BRig_RT_dataMTrig_Solenoid_RewCalib_OnOff__L.vi"() -> ("output_Solenoid_RewCalib_OnOff__L"=w656:i32)  [unwired: 11 in]
              n398 = Index Array(array=w639, index #1=w640, index #2=w637) -> (element #1=w650:u16, element #2=w645:u16)
              n399 = Index Array(array=w639, index #1=w655, index #2=w656) -> (element #1=w666:u16, element #2=w661:u16)
              n400 = Equal To 0?(x=w650) -> (x = 0?=w651:bool)
              n401 = Not Equal To 0?(x=w645) -> (x != 0?=w648:bool)
              n402 = Equal To 0?(x=w666) -> (x = 0?=w667:bool)
              n403 = Not Equal To 0?(x=w661) -> (x != 0?=w664:bool)
              n404 = local write "MTrig_Solenoid_trig__L"(w635) -> ()
              n405 = local write "MTrig_Solenoid_trig__R"(w635) -> ()
              n406 = Select(t=u8 1, s=w638, f=w646) -> (s? t:f=w642:u8)
              n407 = Select(t=u8 1, s=w669, f=w662) -> (s? t:f=w658:u8)
              n408 = Select(t=u8 2, s=w651, f=w646) -> (s? t:f=w643:u8)
              n409 = Select(t=u8 4, s=w648, f=w646) -> (s? t:f=w644:u8)
              n410 = Select(t=u8 2, s=w667, f=w662) -> (s? t:f=w659:u8)
              n411 = Select(t=u8 4, s=w664, f=w662) -> (s? t:f=w660:u8)
              n412 = Compound Arithmetic op=ADD(w642, w643, w644) -> (w641:u8)
              n413 = Compound Arithmetic op=ADD(w658, w659, w660) -> (w657:u8)
              n414 = case shown="7" w657 {
                tunnel: w639 -> [w699 w704 w706 w711 w716 w718 w721 w726]
                tunnel: [w699 w705 w706 w712 w717 w718 w722 w727] -> w654
                tunnel: w656 -> [_ w702 _ w709 w714 _ w720 w725]
                tunnel: w655 -> [_ w703 _ w710 w715 _ _ _]
                frame 0, Default {
                }
                frame 1 {
                  n415 = Replace Array Subset(array=w704, new element #1=u16 100 ("new element/subarray"), index #1=w703, new element #2=u16 1 ("new element/subarray"), index #2=w702) -> (w705:u16[])
                }
                frame 2 {
                }
                frame 3 {
                  n416 = Replace Array Subset(array=w711, new element #1=u16 100 ("new element/subarray"), index #1=w710, new element #2=u16 1 ("new element/subarray"), index #2=w709) -> (w712:u16[])
                }
                frame 4 {
                  w713 = u16 0 ("new element/subarray")
                  n417 = Replace Array Subset(array=w716, new element #1=w713, index #1=w715, new element #2=w713, index #2=w714) -> (w717:u16[])
                }
                frame 5 {
                }
                frame 6 {
                  n418 = Replace Array Subset(array=w721, new element=u16 0 ("new element/subarray"), index=w720) -> (w722:u16[])
                }
                frame 7 {
                  n419 = local write "RewCalib_Trig_L"(FALSE ("RewCalib_Trig_L")) -> ()
                  n420 = Replace Array Subset(array=w726, new element=u16 0 ("new element/subarray"), index=w725) -> (w727:u16[])
                }
              }
              n421 = case shown="7" w641 {
                tunnel: w654 -> [w670 w675 w677 w682 w687 w689 w692 w697]
                tunnel: [w670 w676 w677 w683 w688 w689 w693 w698] -> w653
                tunnel: w637 -> [_ w673 _ w680 w685 _ w691 w696]
                tunnel: w640 -> [_ w674 _ w681 w686 _ _ _]
                frame 0, Default {
                }
                frame 1 {
                  n422 = Replace Array Subset(array=w675, new element #1=u16 100 ("new element/subarray"), index #1=w674, new element #2=u16 1 ("new element/subarray"), index #2=w673) -> (w676:u16[])
                }
                frame 2 {
                }
                frame 3 {
                  n423 = Replace Array Subset(array=w682, new element #1=u16 100 ("new element/subarray"), index #1=w681, new element #2=u16 1 ("new element/subarray"), index #2=w680) -> (w683:u16[])
                }
                frame 4 {
                  w684 = u16 0 ("new element/subarray")
                  n424 = Replace Array Subset(array=w687, new element #1=w684, index #1=w686, new element #2=w684, index #2=w685) -> (w688:u16[])
                }
                frame 5 {
                }
                frame 6 {
                  n425 = Replace Array Subset(array=w692, new element=u16 0 ("new element/subarray"), index=w691) -> (w693:u16[])
                }
                frame 7 {
                  n426 = local write "RewCalib_Trig_R"(FALSE ("RewCalib_Trig_L")) -> ()
                  n427 = Replace Array Subset(array=w697, new element=u16 0 ("new element/subarray"), index=w696) -> (w698:u16[])
                }
              }
            }
            frame "DispenseWater_pre" {
              w734 = u16 0 ("t")
              w777 = u16 0 ("new element/subarray")
              # "just trust me on this one"
              # "RewCalib\nOnOff"
              # "RewCalib\nOnOff"
              # "nCycle"
              # "Solenoid__R"
              # "Tdelay"
              # "delay"
              # "nCycle"
              # "Solenoid__L"
              # "Tdelay"
              # "delay"
              # "Solenoid__R"
              # "count"
              # "Solenoid_Tcycle_R"
              # "Solenoid_Tcycle_L"
              # "Solenoid__L"
              # "count"
              n428 = call "myRIO_BRig_RT_dataMTrig_Solenoid_RewCalib_OnOff__L.vi"() -> ("output_Solenoid_RewCalib_OnOff__L"=w741:i32)  [unwired: 11 in]
              n429 = call "myRIO_BRig_RT_dataMTrig_Solenoid_N__L.vi"() -> ("output_Solenoid_N__L"=w732:i32)  [unwired: 11 in]
              n430 = call "myRIO_BRig_RT_dataMTrig_Solenoid_delay__L.vi"() -> ("output_Solenoid_delay__L"=w775:i32)  [unwired: 11 in]
              n431 = call "myRIO_BRig_RT_dataMTrig_Solenoid_Tdelay__L.vi"() -> ("output_Solenoid_Tdelay__L"=w774:i32)  [unwired: 11 in]
              n432 = call "myRIO_BRig_RT_dataMTrig_Solenoid_N__R.vi"() -> ("output_Solenoid_N__R"=w730:i32)  [unwired: 11 in]
              n433 = call "myRIO_BRig_RT_dataMTrig_Solenoid_delay__R.vi"() -> ("output_Solenoid_delay__R"=w764:i32)  [unwired: 11 in]
              n434 = call "myRIO_BRig_RT_dataMTrig_Solenoid_Tdelay__R.vi"() -> ("output_Solenoid_Tdelay__R"=w763:i32)  [unwired: 11 in]
              n435 = call "myRIO_BRig_RT_dataMTrig_Solenoid_RewCalib_OnOff__R.vi"() -> ("output_Solenoid_RewCalib_OnOff__R"=w737:i32)  [unwired: 11 in]
              n436 = Index Array(array=w776, index #1=w732, index #2=w775, index #3=w774, index #4=w730, index #5=w764, index #6=w763, index #7=w741, index #8=w737) -> (element #1=w733:u16, element #2=w773:u16, element #3=w768:u16, element #4=w736:u16, element #5=w758:u16, element #6=w757:u16, element #7=w742:u16, element #8=w739:u16)
              n437 = Equal To 0?(x=w773) -> (x = 0?=w772:bool)
              n438 = Equal To 0?(x=w758) -> (x = 0?=w762:bool)
              n439 = local read "RewCalib_Trig_L"() -> (w753:bool)
              n440 = local read "RewCalib_Trig_R"() -> (w748:bool)
              n441 = Not Equal To 0?(x=w733) -> (x != 0?=w771:bool)
              n442 = Not Equal To 0?(x=w736) -> (x != 0?=w761:bool)
              n443 = local read "MTrig_Solenoid_Tcycle__L"() -> (w770:u16)
              n444 = local read "MTrig_Solenoid_Tcycle__R"() -> (w756:u16)
              n445 = Not Equal To 0?(x=w742) -> (x != 0?=w752:bool)
              n446 = Not Equal To 0?(x=w739) -> (x != 0?=w750:bool)
              n447 = Not(x=w753) -> (.not. x?=w751:bool)
              n448 = Not(x=w748) -> (.not. x?=w749:bool)
              n449 = And(x=w752, y=w751) -> (x .and. y?=w747:bool)
              n450 = And(x=w750, y=w749) -> (x .and. y?=w746:bool)
              n451 = call "myRIO_BRig_RT_dataMTrig_Solenoid_c__L.vi"() -> ("output_Solenoid_c__L"=w779:i32)  [unwired: 11 in]
              n452 = call "myRIO_BRig_RT_dataMTrig_Solenoid_c__R.vi"() -> ("output_Solenoid_c__R"=w778:i32)  [unwired: 11 in]
              n453 = Select(t=w770, s=w771, f=u16 0) -> (s? t:f=w767:u16)
              n454 = Or(x=w747, y=w746) -> (x .or. y?=w735:bool)
              n455 = Select(t=w756, s=w761, f=u16 0) -> (s? t:f=w759:u16)
              n456 = Select(t=w767, s=w772, f=w768) -> (s? t:f=w765:u16)
              n457 = Select(t=w759, s=w762, f=w757) -> (s? t:f=w754:u16)
              n458 = call "myRIO_BRig_RT_dataMTrig_Solenoid_Tcycle__L.vi"() -> ("output_Solenoid_Tcycle__L"=w766:i32)  [unwired: 11 in]
              n459 = call "myRIO_BRig_RT_dataMTrig_Solenoid_Tcycle__R.vi"() -> ("output_Solenoid_Tcycle__R"=w755:i32)  [unwired: 11 in]
              n460 = Select(t=w734, s=w735, f=w733) -> (s? t:f=w731:u16)
              n461 = Select(t=w734, s=w735, f=w736) -> (s? t:f=w729:u16)
              n462 = Select(t=myRIO_BRig_RT__Case_NonExp_stateList."Idle" ("Enum"), s=w735, f=myRIO_BRig_RT__Case_NonExp_stateList."DispenseWater" ("Enum")) -> (s? t:f=w743:T1)
              n463 = Select(t=w734, s=w735, f=w742) -> (s? t:f=w740:u16)
              n464 = Select(t=w734, s=w735, f=w739) -> (s? t:f=w738:u16)
              n465 = Replace Array Subset(array=w776, new element #1=w777, index #1=w779, new element #2=w777, index #2=w778, new element #3=w765, index #3=w766, new element #4=w754, index #4=w755, new element #5=w740, index #5=w741, new element #6=w738, index #6=w737, new element #7=w731, index #7=w732, new element #8=w729, index #8=w730) -> (w780:u16[])
            }
            frame "DispenseWater" {
              # "D"
              # "C"
              # "B"
              # "A"
              # "(A) Add COUNT and INCREMENT\n(B) Is (A) smaller than Tcycle?\n(C) Are we dispensing water or in the delay phase?\n(D) If (A) is smaller than Tcycle   AND   if we are dispensing water\n      then send TRUE to solenoid"
              # "delay"
              # "Tcycle"
              # "Solenoid__R"
              # "count"
              # "delay"
              # "Tcycle"
              # "Solenoid__L"
              # "count"
              n466 = To Unsigned Word Integer(number=w808) -> (unsigned 16bit integer=w790:u16)
              n467 = call "myRIO_BRig_RT_dataMTrig_Solenoid_delay__R.vi"() -> ("output_Solenoid_delay__R"=w794:i32)  [unwired: 11 in]
              n468 = call "myRIO_BRig_RT_dataMTrig_Solenoid_c__R.vi"() -> ("output_Solenoid_c__R"=w793:i32)  [unwired: 11 in]
              n469 = call "myRIO_BRig_RT_dataMTrig_Solenoid_Tcycle__R.vi"() -> ("output_Solenoid_Tcycle__R"=w795:i32)  [unwired: 11 in]
              n470 = call "myRIO_BRig_RT_dataMTrig_Solenoid_delay__L.vi"() -> ("output_Solenoid_delay__L"=w810:i32)  [unwired: 11 in]
              n471 = call "myRIO_BRig_RT_dataMTrig_Solenoid_c__L.vi"() -> ("output_Solenoid_c__L"=w802:i32)  [unwired: 11 in]
              n472 = call "myRIO_BRig_RT_dataMTrig_Solenoid_Tcycle__L.vi"() -> ("output_Solenoid_Tcycle__L"=w811:i32)  [unwired: 11 in]
              n473 = Index Array(array=w804, index #1=w802, index #2=w811, index #3=w810, index #4=w793, index #5=w795, index #6=w794) -> (element #1=w809:u16, element #2=w799:u16, element #3=w807:u16, element #4=w789:u16, element #5=w786:u16, element #6=w785:u16)
              n474 = Add(x=w809, y=w790) -> (x+y=w800:u16)
              n475 = Add(x=w789, y=w790) -> (x+y=w791:u16)
              n476 = Less?(x=w800, y=w799) -> (x < y?=w783:bool)
              n477 = Equal To 0?(x=w807) -> (x = 0?=w806:bool)
              n478 = Less?(x=w791, y=w786) -> (x < y?=w784:bool)
              n479 = Equal To 0?(x=w785) -> (x = 0?=w792:bool)
              n480 = And(x=w783, y=w806) -> (x .and. y?=w805:bool)
              n481 = Or(x=w783, y=w784) -> (x .or. y?=w782:bool)
              n482 = And(x=w784, y=w792) -> (x .and. y?=w787:bool)
              n483 = Select(t=w800, s=w783, f=w799) -> (s? t:f=w801:u16)
              n484 = Select(t=w791, s=w784, f=w786) -> (s? t:f=w788:u16)
              n485 = Replace Array Subset(array=w804, new element #1=w801, index #1=w802, new element #2=w788, index #2=w793) -> (w803:u16[])
              n486 = Select(t=w798, s=w782, f=myRIO_BRig_RT__Case_NonExp_stateList."DispenseWater_post" ("Enum")) -> (s? t:f=w796:T1)
            }
            frame "DispenseWater_post" {
              # "nCycle"
              # "delay"
              # "Solenoid__R"
              # "nCycle"
              # "delay"
              # "Solenoid__L"
              n487 = call "myRIO_BRig_RT_dataMTrig_Solenoid_N__L.vi"() -> ("output_Solenoid_N__L"=w829:i32)  [unwired: 11 in]
              n488 = call "myRIO_BRig_RT_dataMTrig_Solenoid_delay__L.vi"() -> ("output_Solenoid_delay__L"=w828:i32)  [unwired: 11 in]
              n489 = call "myRIO_BRig_RT_dataMTrig_Solenoid_N__R.vi"() -> ("output_Solenoid_N__R"=w825:i32)  [unwired: 11 in]
              n490 = call "myRIO_BRig_RT_dataMTrig_Solenoid_delay__R.vi"() -> ("output_Solenoid_delay__R"=w824:i32)  [unwired: 11 in]
              n491 = Index Array(array=w831, index #1=w829, index #2=w828, index #3=w825, index #4=w824) -> (element #1=w833:u16, element #2=w832:u16, element #3=w816:u16, element #4=w818:u16)
              n492 = Not Equal To 0?(x=w833) -> (x != 0?=w834:bool)
              n493 = Not Equal To 0?(x=w816) -> (x != 0?=w817:bool)
              n494 = case shown="True" w817 {
                selector: w817 -> [_ w838]
                tunnel: w816 -> [w836 w844]
                tunnel: w818 -> [_ w845]
                tunnel: [w836 w842] -> w815
                tunnel: [u16 0 w841] -> w814
                tunnel: [_ w838] -> w813
                frame False {
                }
                frame True {
                  n495 = Equal To 0?(x=w845) -> (x = 0?=w837:bool)
                  n496 = Decrement(x=w844) -> (x-1=w843:u16)
                  n497 = Select(t=w843, s=w837, f=w844) -> (s? t:f=w842:u16)
                  n498 = Select(t=u16 1, s=w837, f=u16 0) -> (s? t:f=w841:u16)
                }
              }
              n499 = case shown="True" w834 {
                selector: w834 -> [_ w849]
                tunnel: w833 -> [w847 w855]
                tunnel: w832 -> [_ w856]
                tunnel: [w847 w853] -> w827
                tunnel: [u16 0 w852] -> w826
                tunnel: [_ w849] -> w823
                frame False {
                }
                frame True {
                  n500 = Equal To 0?(x=w856) -> (x = 0?=w848:bool)
                  n501 = Decrement(x=w855) -> (x-1=w854:u16)
                  n502 = Select(t=w854, s=w848, f=w855) -> (s? t:f=w853:u16)
                  n503 = Select(t=u16 1, s=w848, f=u16 0) -> (s? t:f=w852:u16)
                }
              }
              n504 = Or(x=w823, y=w813) -> (x .or. y?=w822:bool)
              n505 = Replace Array Subset(array=w831, new element #1=w827, index #1=w829, new element #2=w826, index #2=w828, new element #3=w815, index #3=w825, new element #4=w814, index #4=w824) -> (w830:u16[])
              n506 = Select(t=myRIO_BRig_RT__Case_NonExp_stateList."DispenseWater_pre" ("Enum"), s=w822, f=myRIO_BRig_RT__Case_NonExp_stateList."Idle" ("Enum")) -> (s? t:f=w819:T1)
            }
            frame "TestConnection" {
              n507 = local read "Host Password"() -> (w863:string)
              n508 = local read "Host UserName"() -> (w864:string)
              n509 = call "myRIO_BRig_RT_comm_webdav_testConnect.vi"("input_password"=w863, "input_username"=w864) -> ("output_Iconnected"=w861:bool)  [unwired: 9 in]
              n510 = Select(t="Connection accepted!" ("message"), s=w861, f="Error!") -> (s? t:f=w859:string)
              n511 = One Button Dialog(message=w859) -> ()  [unwired: 1 in, 1 out]
            }
            frame "SendData" {
              n512 = local read "Data Set Prefix"() -> (w866:string)
              n513 = local read "Host Password"() -> (w867:string)
              n514 = local read "Host UserName"() -> (w868:string)
              n515 = call "myRIO_BRig_RT_comm_webdav_sendData_all.vi"("Host Filename Prefix"=w866, "Host Password"=w867, "Host UserName"=w868) -> ()  [unwired: 9 in]
            }
            frame "Get_FPGA_count_per_ms" {
              n516 = case shown="False" w882 {
                selector: w882 -> [w885 _]
                tunnel: w880 -> [_ w898]
                tunnel: [w889 w898] -> w879
                tunnel: w878 -> [w888 w896]
                tunnel: w877 -> [w887 w895]
                tunnel: [w886 w893] -> w876
                tunnel: [w885 w892] -> w875
                frame False {
                  n517 = Get Date/Time In Seconds() -> (seconds since 1Jan1904=w890:timestamp)
                  n518 = xnode "Read/Write Control"("FPGA VI Reference In"=w888, "error in"=w887, "timeTrial"=TRUE) -> ("error out"=w886:errorcluster)  [unwired: 1 out]
                  n519 = To Double Precision Float(number=w890) -> (double precision float=w889:dbl)
                  n520 = local write "get_countPerMS"(w885) -> ()
                }
                frame True {
                  w894 = 1.0
                  n521 = Get Date/Time In Seconds() -> (seconds since 1Jan1904=w899:timestamp)
                  n522 = To Double Precision Float(number=w899) -> (double precision float=w900:dbl)
                  n523 = Subtract(x=w900, y=w898) -> (x-y=w897:dbl)
                  n524 = Less Or Equal?(x=w894, y=w897) -> (x <= y?=w892:bool)
                  n525 = case shown="True" w892 {
                    tunnel: w896 -> [_ w913]
                    tunnel: w895 -> [w901 w912]
                    tunnel: w894 -> [_ w903]
                    tunnel: [w901 w902] -> w893
                    frame False {
                    }
                    frame True {
                      n526 = xnode "Read/Write Control"("FPGA VI Reference In"=w913, "error in"=w912) -> ("FPGA VI Reference Out"=w910:refnum<k20>, "error out"=w909:errorcluster, "count_timeTrial"=w904:u32)
                      n527 = Multiply(x=w903, y=1000.0) -> (x*y=w907:dbl)
                      n528 = To Double Precision Float(number=w904) -> (double precision float=w906:dbl)
                      n529 = Divide(x=w906, y=w907) -> (x/y=w908:dbl)
                      n530 = local write "f_millisec2count"(w908) -> ()
                      n531 = xnode "Read/Write Control"("FPGA VI Reference In"=w910, "error in"=w909, "timeTrial"=FALSE) -> ("error out"=w902:errorcluster)  [unwired: 1 out]
                    }
                  }
                }
              }
              "error out 5" <- w876
              n532 = Select(t=myRIO_BRig_RT__Case_NonExp_stateList."Idle" ("Enum"), s=w875, f=w873) -> (s? t:f=w872:T1)
            }
            frame "End" {
            }
          }
          n533 = local read "MTrig_Audio_trig__R"() -> (w119:bool)
          n534 = local read "MTrig_Audio_trig__L"() -> (w118:bool)
          n535 = local read "START"() -> (w114:bool)
          n536 = local read "STOP_abort"() -> (w113:bool)
          n537 = local read "MTrig_Laser_trig"() -> (w120:bool)
          n538 = call "myRIO_BRig_RT_dataMTrig_main__v2.vi"("input_dataMTrig"=w122, "input_Audio_trig_L"=w118, "input_Audio_trig_R"=w119, "input_Laser_trig"=w120) -> ("output_dataMTrig"=w121:u16[], "output_Audio_L"=w98:bool, "output_Audio_R"=w109:bool, "output_Laser"=w101:bool)  [unwired: 12 in]
          n539 = Or(x=w114, y=w113) -> (x .or. y?=w112:bool)
          n540 = Select(t=myRIO_BRig_RT__Case_NonExp_stateList."End" ("Enum"), s=w112, f=w111) -> (s? t:f=w110:T1)
          n541 = Or(x=w119, y=w120) -> (x .or. y?=w117:bool)
          n542 = Or(x=w117, y=w118) -> (x .or. y?=w116:bool)
          n543 = case shown="True" w116 {
            frame False {
            }
            frame True {
              w135 = FALSE
              n544 = local write "MTrig_Audio_trig__R"(w135) -> ()
              n545 = local write "MTrig_Audio_trig__L"(w135) -> ()
              n546 = local write "MTrig_Laser_trig"(w135) -> ()
            }
          }
          n547 = xnode "Read/Write Control"("FPGA VI Reference In"=w87, "error in"=w86, "A1_SR"=w123, "A3_SL"=w124, "audioTrigger_L"=w98, "audioTrigger_R"=w109, "laserResponse_reward_LED"="laserResponse_reward_LED", "laserResponse_wrong_LED"="laserResponse_wrong_LED", "laserResponse_reward"="laserResponse_reward", "laserResponse_wrong"="laserResponse_wrong", "SelectionState"="SelectionState", "ignoreWrong"="ignoreWrong", "Left(F)_or_Right(T)"="Left(F)_or_Right(T)", "laserMTrig"=w101) -> ("FPGA VI Reference Out"=w129:refnum<k20>, "error out"=w128:errorcluster, "SelectReward"=→"SelectReward":bool, "SelectWrong"=→"SelectWrong":bool, "AnaIn_0"=→"tempAI0":i16)
          n548 = node-c288() -> ()  [unwired: 1 in, 1 out]
          "cState_NonExp" <- w127
        }
        n549 = node-c288(w69) -> ()  [unwired: 1 out]
        n550 = flat-sequence {
          tunnel: w62 -> [w80]
          tunnel: [w80] -> w61
          tunnel: w60 -> [w79]
          tunnel: [w79] -> w59
          frame #0 {
            w78 = FALSE
            n551 = local write "STOP_endBlock"(w78) -> ()
            n552 = local write "STOP_endTrial"(w78) -> ()
          }
        }
      }
      frame True {
        w938 = u16 0
        w941 = u8 0
        w942 = FALSE ("SelectionState")
        w947 = u16 0 ("idxDataBlock")
        w949 = u16 100 ("new element/subarray")
        w950 = u16 100 ("new element/subarray")
        w970 = T6 refnum items=["Session NI_WebDAV"] ("output_hSession")
        w979 = FALSE
        w980 = u16 0
        w928 = FALSE
        # "audio__L\naudio__R"
        # "Audio params"
        # "nRewards"
        # "idxDataBlock"
        # "Solenoid_Tdelay_R"
        # "Solenoid_Tdelay_L"
        # "RewCalib_N__R"
        # "RewCalib_N__L"
        # "Save dataLick to file\nSend file to Host\nSave dataMTrig\nSend file to Host\nDisconnect"
        # "dataTrial"
        # "dataTrial"
        # "Solenoid_Tcycle_R"
        # "Solenoid_Tcycle_L"
        # "Laser_Tcycle"
        # "Audio_Tcycle_R"
        # "Audio_Tcycle_L"
        # "dataLick"
        # "dataLC"
        # "dataLC"
        # "dataBlock"
        # "dataBlock"
        # "dataMTrig"
        # "dataMTrig"
        # "dataExp"
        # "dataCurrent"
        # "dataExp"
        # "dataCurrent"
        # "spout"
        # "state"
        n553 = call "myRIO_BRig_RT_dataMTrig_Solenoid_Tcycle__L.vi"() -> ("output_Solenoid_Tcycle__L"=w976:i32)  [unwired: 11 in]
        n554 = call "myRIO_BRig_RT_dataMTrig_Solenoid_Tcycle__R.vi"() -> ("output_Solenoid_Tcycle__R"=w975:i32)  [unwired: 11 in]
        n555 = call "myRIO_BRig_RT_dataMTrig_Audio_Tcycle__L.vi"() -> ("output_Audio_Tcycle__L"=w974:i32)  [unwired: 11 in]
        n556 = call "myRIO_BRig_RT_dataMTrig_Audio_Tcycle__R.vi"() -> ("output_Audio_Tcycle__R"=w973:i32)  [unwired: 11 in]
        n557 = call "myRIO_BRig_RT_dataMTrig_Laser_Tcycle.vi"() -> ("output_Laser_Tcycle"=w972:i32)  [unwired: 11 in]
        n558 = local read "MTrig_Solenoid_Tcycle__L"() -> (w955:u16)
        n559 = local read "MTrig_Solenoid_Tcycle__R"() -> (w954:u16)
        n560 = local read "Tcycle_Reward_L"() -> (w951:u16)
        n561 = local read "Tcycle_Reward_R"() -> (w952:u16)
        n562 = local read "MTrig_Laser_Tcycle"() -> (w953:u16)
        n563 = call "myRIO_BRig_RT_dataMTrig_Solenoid_RewCalib_nCycle__L.vi"() -> ("output_Solenoid_RewCalib_nCycle__L"=w958:i32)  [unwired: 11 in]
        n564 = call "myRIO_BRig_RT_dataMTrig_Solenoid_Tdelay__L.vi"() -> ("output_Solenoid_Tdelay__L"=w960:i32)  [unwired: 11 in]
        n565 = call "myRIO_BRig_RT_dataMTrig_Solenoid_RewCalib_nCycle__R.vi"() -> ("output_Solenoid_RewCalib_nCycle__R"=w959:i32)  [unwired: 11 in]
        n566 = call "myRIO_BRig_RT_dataMTrig_Solenoid_Tdelay__R.vi"() -> ("output_Solenoid_Tdelay__R"=w961:i32)  [unwired: 11 in]
        n567 = case shown="False" w932 {
          selector: w932 -> [_ w1002]
          tunnel: w931 -> [w999 w1004]
          tunnel: [w1000 w1004] -> w926
          tunnel: w930 -> [_ w1003]
          tunnel: [w1001 w1003] -> w927
          tunnel: [w998 w1002] -> w925
          frame False {
            n568 = call "myRIO__TCP_connect_forWriting.vi"("input_error"=w999) -> ("output_error"=w1000:errorcluster, "output_connected"=w998:bool, "output_hTCP"=w1001:refnum<k5>)  [unwired: 8 in]
          }
          frame True {
          }
        }
        n569 = call "myRIO_BRig_RT_dataLick_init.vi"() -> ("output_dataLick"=w982:u16[][])  [unwired: 11 in]
        n570 = call "myRIO_BRig_RT_dataCurrent_init.vi"() -> ("output_dataCurrent"=w989:u16[])  [unwired: 11 in]
        n571 = call "myRIO_BRig_RT_dataExp_init.vi"() -> ("output_dataExp"=w988:u16[])  [unwired: 11 in]
        n572 = call "myRIO_BRig_RT_dataMTrig_init.vi"() -> ("output_dataMTrig"=w978:u16[])  [unwired: 5 in]
        n573 = call "myRIO_BRig_RT_dataLC_init.vi"() -> ("output_dataLC"=w986:u16[])  [unwired: 11 in]
        n574 = call "myRIO_BRig_RT_dataBlock_init.vi"() -> ("output_dataBlock"=w987:u16[][])  [unwired: 11 in]
        n575 = call "myRIO_BRig_RT_dataTrial_init.vi"() -> ("output_dataTrial"=w971:u16[][])  [unwired: 11 in]
        n576 = xnode "Read/Write Control"("FPGA VI Reference In"=w943, "error in"=w944, "SelectionState"=w942, "laserResponse_reward"=w942, "laserResponse_wrong"=w942, "laserResponse_reward_LED"=w942, "laserResponse_wrong_LED"=w942, "Left(F)_or_Right(T)"=w942, "ignoreWrong"=w942, "SelectionState"=w942) -> ("FPGA VI Reference Out"=w945:refnum<k20>, "error out"=w946:errorcluster)
        n577 = local write "I_connect_TCP"(w925) -> ()
        n578 = Replace Array Subset(array=w978, new element #1=w950, index #1=w958, new element #2=w950, index #2=w959, new element #3=w949, index #3=w960, new element #4=w949, index #4=w961, new element #5=w955, index #5=w976, new element #6=w954, index #6=w975, new element #7=w951, index #7=w974, new element #8=w952, index #8=w973, new element #9=w953, index #9=w972) -> (w977:u16[])
        n579 = call "myRIO_BRig_RT_dataAnalog_init.vi"() -> ("output_dataAnalog"=w937:u16[][])  [unwired: 11 in]
        n580 = call "myRIO_BRig_RT_TCP__start_exp.vi"("input_hTCP"=w927, "input_I_connected_TCP"=w925, "input_error"=w926) -> ("output_hTCP"=w924:refnum<k5>, "output_error"=w923:errorcluster)  [unwired: 11 in]
        n581 = Get Date/Time In Seconds() -> (seconds since 1Jan1904=w957:timestamp)
        n582 = To Double Precision Float(number=w957) -> (double precision float=w956:dbl)
        n583 = node-c288() -> (w997:T3)  [unwired: 4 in]
        n584 = timed-loop {
          timing: w997 -> [_]
          timing-out: [_] -> w996
          shift-right: [w1117] -> _
          shift-left: myRIO_BRig_RT__Case_Exp_stateList."Start1" ("Enum") -> [w1049]
          shift-right: [w1046] -> _
          shift-left: enum16{"Left", "Right"}."Left" -> [w1168]
          tunnel: w945 -> [w1166]
          tunnel: w946 -> [w1165]
          shift-right: [w1160] -> _
          shift-left: w994 -> [w1164]
          shift-right: [w1159] -> _
          shift-left: w993 -> [w1163]
          tunnel: [w1142] -> w991
          tunnel: [w1143] -> w992
          shift-right: [w1144] -> w962
          shift-left: w989 -> [w1109]
          shift-right: [w1158] -> _
          shift-left: w988 -> [w1104]
          shift-right: [w1131] -> w966
          shift-left: w977 -> [w1132]
          shift-right: [w1156] -> _
          shift-left: w987 -> [w1157]
          shift-right: [w1154] -> _
          shift-left: w986 -> [w1155]
          shift-right: [w1146] -> w968
          shift-left: w982 -> [w1147]
          shift-right: [w1133] -> _
          shift-left: w980 -> [w1141]
          shift-right: [w1101] -> _
          shift-left: w941 -> [w1140]
          shift-right: [w1134] -> _
          shift-left: w980 -> [w1139]
          shift-right: [w1135] -> _
          shift-left: w941 -> [w1138]
          shift-right: [w1102] -> _
          shift-left: w979 -> [w1136]
          shift-right: [w1103] -> _
          shift-left: w979 -> [w1137]
          shift-right: [w1115] -> _
          shift-left: w971 -> [w1116]
          shift-right: [w1114] -> w964
          shift-left: w970 -> [w1112]
          shift-right: [w1113] -> w965
          shift-left: FALSE ("output_Iconnected") -> [w1111]
          tunnel: "Data Set Prefix" -> [w1110]
          tunnel: [w1110] -> w963
          shift-right: [w1086] -> _
          shift-left: w928 -> [w1108]
          tunnel: w956 -> [w1105]
          shift-right: [w1099] -> _
          shift-left: 0 ("idxDataBlock") -> [w1100]
          shift-right: [w1096] -> _
          shift-left: w947 -> [w1098]
          shift-right: [w1095] -> _
          shift-left: w947 -> [w1097]
          shift-right: [w1085] -> _
          shift-left: w928 -> [w1091]
          shift-right: [w1088] -> _
          shift-left: w928 -> [w1090]
          shift-right: [w1087] -> _
          shift-left: w928 -> [w1089]
          shift-right: [w1073] -> w935
          shift-left: 0 -> [w1057]
          shift-right: [w1047] -> _
          shift-left: w938 -> [w1068]
          shift-right: [w1048] -> _
          shift-left: w938 -> [w1064]
          shift-right: [w1077] -> _
          shift-left: FALSE -> [w1077]
          shift-right: [w1063] -> _
          shift-left: w938 -> [w1071]
          shift-right: [w1074] -> w936
          shift-left: w937 -> [w1075]
          tunnel: w924 -> [w1062]
          tunnel: [w1061] -> w934
          tunnel: w925 -> [w1058]
          tunnel: [w1058] -> w933
          tunnel: w923 -> [w1060]
          tunnel: [w1059] -> w929
          shift-right: [w1052] -> _
          shift-left: w928 -> [w1053]
          shift-right: [w1050] -> _
          shift-left: w928 -> [w1051]
          stop <- w1153 stop-if-true
          # "Sel"
          # "Sel"
          # "Cue1"
          # "Cue1"
          # "ENL1"
          # "ENL1"
          # "iState"
          # "dataAnalog"
          # "index"
          # "iEvent"
          # "iBlock"
          # "iTrial"
          # "Laser"
          # "Audio R"
          # "Audio L"
          # "Solenoid R"
          # "Solenoid L"
          # "manual triggering"
          # "dataTrial"
          # "dataBlock"
          # "nRewards"
          # "dataExp"
          # "dataCurrent"
          # "audio__L\naudio__R"
          # "time stamp"
          # "Audio params"
          # "nRewards"
          # "idxDataBlock"
          # "idxDataBlock"
          # "activate"
          # "audio__L\naudio__R"
          # "amp__R\nfreq__R"
          # "amp__L\nfreq__L"
          # "dataLC"
          # "solenoid__R"
          # "solenoid__L"
          # "Did a lick occur?"
          # "Update lick counter"
          # "spout"
          # "spout"
          # "state"
          # "state"
          n585 = node-c288() -> ()  [unwired: 1 in, 1 out]
          n586 = local read "MTrig_Solenoid_trig__L"() -> (w1129:bool)
          n587 = local read "MTrig_Solenoid_trig__R"() -> (w1128:bool)
          n588 = local read "MTrig_Audio_trig__L"() -> (w1127:bool)
          n589 = local read "MTrig_Audio_trig__R"() -> (w1126:bool)
          n590 = xnode "Read/Write Control"("FPGA VI Reference In"=w1166, "error in"=w1165) -> ("FPGA VI Reference Out"=w1094:refnum<k20>, "error out"=w1093:errorcluster, "A2_LickL"=w1160:u32, "A4_LickR"=w1159:u32)
          "A2" <- w1160
          "A4" <- w1159
          n591 = local read "MTrig_Laser_trig"() -> (w1125:bool)
          n592 = Greater?(x=w1160, y=w1164) -> (0:w1162:bool)
          n593 = Greater?(x=w1159, y=w1163) -> (0:w1161:bool)
          n594 = Or(x=w1162, y=w1161) -> (x .or. y?=w1167:bool)
          n595 = call "myRIO_BRig_RT_dataMTrig_main.vi"("input_dataMTrig"=w1132, "input_Solenoid_trig_L"=w1129, "input_Solenoid_trig_R"=w1128, "input_Audio_trig_L"=w1127, "input_Audio_trig_R"=w1126, "input_Laser_trig"=w1125) -> ("output_Laser"=w1083:bool, "output_dataMTrig"=w1131:u16[], "output_Solenoid_L"=w1119:bool, "output_Solenoid_R"=w1121:bool, "output_Audio_L"=w1123:bool, "output_Audio_R"=w1124:bool)  [unwired: 8 in]
          n596 = Compound Arithmetic op=OR(w1129, w1128, w1127, w1126, w1125) -> (w1130:bool)
          n597 = case shown="True" w1130 {
            frame False {
            }
            frame True {
              w1169 = FALSE
              n598 = local write "MTrig_Solenoid_trig__L"(w1169) -> ()
              n599 = local write "MTrig_Solenoid_trig__R"(w1169) -> ()
              n600 = local write "MTrig_Audio_trig__L"(w1169) -> ()
              n601 = local write "MTrig_Audio_trig__R"(w1169) -> ()
              n602 = local write "MTrig_Laser_trig"(w1169) -> ()
            }
          }
          n603 = case shown="\"initTrial\"" w1049 {
            selector: w1049 -> [_ _ _ _ _ _ _ _ _ _ _ _ _ _ _ _ _ _ _ _ _ w1962 _ w2027 _ _ _ _ _ w2168 _ w2245 _ _ _ _ _ w2400 _ w2474 _ w2538 _ w2582 _ _ w2652 _ _ _ _ _ w2823 _ _ _ _ _ _ _ _ _ _ _ _ _ _ _ _ _ _ _]
            tunnel: [myRIO_BRig_RT__Case_Exp_stateList."Start2" ("Enum") myRIO_BRig_RT__Case_Exp_stateList."Start3" ("Enum") myRIO_BRig_RT__Case_Exp_stateList."saveSettings1" ("Enum") myRIO_BRig_RT__Case_Exp_stateList."saveSettings2" ("Enum") myRIO_BRig_RT__Case_Exp_stateList."saveSettings3" ("Enum") myRIO_BRig_RT__Case_Exp_stateList."saveSettings4_LC_ENL" ("Enum") myRIO_BRig_RT__Case_Exp_stateList."saveSettings5_LC_Cue" ("Enum") myRIO_BRig_RT__Case_Exp_stateList."saveSettings6_LC_Other" ("Enum") myRIO_BRig_RT__Case_Exp_stateList."setSettings_Audio" ("Enum") myRIO_BRig_RT__Case_Exp_stateList."setSettings_Laser" ("Enum") myRIO_BRig_RT__Case_Exp_stateList."commConnect" ("Enum") w1692 myRIO_BRig_RT__Case_Exp_stateList."initTrial" ("Enum") w1737 myRIO_BRig_RT__Case_Exp_stateList."initTrial3" ("Enum") myRIO_BRig_RT__Case_Exp_stateList."initTrial_LC_ENL1" ("Enum") myRIO_BRig_RT__Case_Exp_stateList."ENL1_pre" ("Enum") myRIO_BRig_RT__Case_Exp_stateList."initTrial_LC_Cue1" ("Enum") myRIO_BRig_RT__Case_Exp_stateList."initTrial_LC_Sel" ("Enum") myRIO_BRig_RT__Case_Exp_stateList."initTrial4" ("Enum") w1922 w1959 myRIO_BRig_RT__Case_Exp_stateList."ENL1Penalty" ("Enum") w2028 myRIO_BRig_RT__Case_Exp_stateList."endExp" ("Enum") myRIO_BRig_RT__Case_Exp_stateList."endExp" ("Enum") myRIO_BRig_RT__Case_Exp_stateList."endExp" ("Enum") myRIO_BRig_RT__Case_Exp_stateList."endExp" ("Enum") w2123 w2167 myRIO_BRig_RT__Case_Exp_stateList."Cue1Penalty" ("Enum") w2243 myRIO_BRig_RT__Case_Exp_stateList."endExp" ("Enum") myRIO_BRig_RT__Case_Exp_stateList."endExp" ("Enum") myRIO_BRig_RT__Case_Exp_stateList."endExp" ("Enum") myRIO_BRig_RT__Case_Exp_stateList."endExp" ("Enum") w2340 w2406 myRIO_BRig_RT__Case_Exp_stateList."SelectReward" ("Enum") w2475 myRIO_BRig_RT__Case_Exp_stateList."SelectRewardPost" ("Enum") w2539 myRIO_BRig_RT__Case_Exp_stateList."SelectWrong" ("Enum") w2578 myRIO_BRig_RT__Case_Exp_stateList."endTrial1" ("Enum") myRIO_BRig_RT__Case_Exp_stateList."SelectTimeout" ("Enum") w2654 myRIO_BRig_RT__Case_Exp_stateList."endTrial1" ("Enum") myRIO_BRig_RT__Case_Exp_stateList."endTrial2" ("Enum") myRIO_BRig_RT__Case_Exp_stateList."saveData_dataBlock" ("Enum") w2736 w2806 w2823 myRIO_BRig_RT__Case_Exp_stateList."initBlock" ("Enum") w2850 myRIO_BRig_RT__Case_Exp_stateList."commUpload_dataCurrent" ("Enum") myRIO_BRig_RT__Case_Exp_stateList."commUpload_dataExp" ("Enum") myRIO_BRig_RT__Case_Exp_stateList."commUpload_dataLC" ("Enum") myRIO_BRig_RT__Case_Exp_stateList."commUpload_dataTrial" ("Enum") myRIO_BRig_RT__Case_Exp_stateList."endTrial3" ("Enum") myRIO_BRig_RT__Case_Exp_stateList."saveData_dataCurrent" ("Enum") myRIO_BRig_RT__Case_Exp_stateList."saveData_dataExp" ("Enum") myRIO_BRig_RT__Case_Exp_stateList."saveData_dataLC" ("Enum") myRIO_BRig_RT__Case_Exp_stateList."saveData_dataTrial" ("Enum") myRIO_BRig_RT__Case_Exp_stateList."commUpload_pre" ("Enum") myRIO_BRig_RT__Case_Exp_stateList."initBlock" ("Enum") myRIO_BRig_RT__Case_Exp_stateList."initBlock" ("Enum") myRIO_BRig_RT__Case_Exp_stateList."empty_endTrial2" ("Enum") myRIO_BRig_RT__Case_Exp_stateList."empty_endTrial3" ("Enum") myRIO_BRig_RT__Case_Exp_stateList."empty_endTrial4" ("Enum") myRIO_BRig_RT__Case_Exp_stateList."initTrial" ("Enum") myRIO_BRig_RT__Case_Exp_stateList."initTrial" ("Enum")] -> w1117
            tunnel: [w1195 w1214 w1236 w1291 w1339 w1406 w1470 w1534 w1578 w1604 w1663 w1669 w1700 w1719 w1753 w1783 w1818 w1842 w1868 w1897 w1938 w1975 w2005 w2032 w2048 w2070 w2089 w2108 w2142 w2189 w2214 w2242 w2263 w2284 w2303 w2322 w2351 w2424 w2449 w2472 w2486 w2536 w2560 w2592 w2613 w2633 w2664 w2687 w2699 w2718 w2760 w2779 w2822 w2839 w2853 w2887 w2908 w2929 w2950 w2971 w2999 w3019 w3046 w3066 w3091 w3110 w3129 w3148 w3167 w3186 w3205 w3224] -> w1046
            tunnel: w1168 -> [w1195 w1214 w1236 w1291 w1339 w1406 w1470 w1534 w1578 w1604 w1663 w1691 w1700 w1719 w1753 w1783 w1818 w1842 w1868 w1897 w1938 w1975 w2005 w2032 w2048 w2070 w2089 w2108 w2142 w2189 w2214 w2242 w2263 w2284 w2303 w2322 w2351 w2424 w2449 w2472 w2486 w2536 w2560 w2592 w2613 w2633 w2664 w2687 w2699 w2718 w2760 w2779 w2822 w2839 w2853 w2887 w2908 w2929 w2950 w2971 w2999 w3019 w3046 w3066 w3091 w3110 w3129 w3148 w3167 w3186 w3205 w3224]
            tunnel: w1167 -> [w1198 w1217 w1233 w1294 w1342 w1409 w1473 w1537 w1581 w1607 w1666 w1685 w1711 w1738 w1771 w1799 w1832 w1855 w1881 w1910 w1925 w1956 w2008 w2035 w2054 w2073 w2092 w2111 w2122 w2166 w2222 w2249 w2268 w2287 w2306 w2325 w2349 w2422 w2459 w2482 w2517 w2544 w2571 w2595 w2612 w2645 w2669 w2684 w2707 w2717 w2771 w2805 w2826 w2836 w2862 w2890 w2911 w2932 w2953 w2974 w3002 w3022 w3049 w3069 w3094 w3113 w3132 w3151 w3170 w3189 w3208 w3227]
            tunnel: w1162 -> [w1197 w1216 w1234 w1293 w1341 w1408 w1472 w1536 w1580 w1606 w1665 w1684 w1710 w1739 w1770 w1800 w1833 w1856 w1882 w1911 w1948 w1977 w2007 w2034 w2053 w2072 w2091 w2110 w2156 w2190 w2221 w2248 w2267 w2286 w2305 w2324 w2350 w2421 w2458 w2481 w2516 w2543 w2570 w2594 w2611 w2644 w2668 w2685 w2708 w2716 w2770 w2804 w2825 w2837 w2863 w2889 w2910 w2931 w2952 w2973 w3001 w3021 w3048 w3068 w3093 w3112 w3131 w3150 w3169 w3188 w3207 w3226]
            tunnel: w1161 -> [w1196 w1215 w1235 w1292 w1340 w1407 w1471 w1535 w1579 w1605 w1664 w1683 w1709 w1740 w1769 w1801 w1834 w1857 w1883 w1912 w1947 w1976 w2006 w2033 w2052 w2071 w2090 w2109 w2155 w2191 w2220 w2247 w2266 w2285 w2304 w2323 w2368 w2425 w2457 w2480 w2515 w2542 w2569 w2593 w2610 w2643 w2667 w2686 w2709 w2715 w2769 w2803 w2824 w2838 w2864 w2888 w2909 w2930 w2951 w2972 w3000 w3020 w3047 w3067 w3092 w3111 w3130 w3149 w3168 w3187 w3206 w3225]
            tunnel: [w1198 w1217 w1233 w1294 w1342 w1409 w1473 w1537 w1581 w1607 w1666 w1685 w1711 w1738 w1771 w1799 w1832 w1855 w1881 w1910 w1925 w1956 w2008 w2035 w2054 w2073 w2092 w2111 w2122 w2166 w2222 w2249 w2268 w2287 w2306 w2325 w2349 w2422 w2459 w2482 w2517 w2544 w2571 w2595 w2612 w2645 w2669 w2684 w2707 w2717 w2771 w2805 w2826 w2836 w2862 w2890 w2911 w2932 w2953 w2974 w3002 w3022 w3049 w3069 w3094 w3113 w3132 w3151 w3170 w3189 w3208 w3227] -> w1150
            tunnel: [w1197 w1216 w1234 w1293 w1341 w1408 w1472 w1536 w1580 w1606 w1665 w1684 w1710 w1739 w1770 w1800 w1833 w1856 w1882 w1911 w1948 w1977 w2007 w2034 w2053 w2072 w2091 w2110 w2156 w2190 w2221 w2248 w2267 w2286 w2305 w2324 w2350 w2421 w2458 w2481 w2516 w2543 w2570 w2594 w2611 w2644 w2668 w2685 w2708 w2716 w2770 w2804 w2825 w2837 w2863 w2889 w2910 w2931 w2952 w2973 w3001 w3021 w3048 w3068 w3093 w3112 w3131 w3150 w3169 w3188 w3207 w3226] -> w1149
            tunnel: [w1196 w1215 w1235 w1292 w1340 w1407 w1471 w1535 w1579 w1605 w1664 w1683 w1709 w1740 w1769 w1801 w1834 w1857 w1883 w1912 w1947 w1976 w2006 w2033 w2052 w2071 w2090 w2109 w2155 w2191 w2220 w2247 w2266 w2285 w2304 w2323 w2368 w2425 w2457 w2480 w2515 w2542 w2569 w2593 w2610 w2643 w2667 w2686 w2709 w2715 w2769 w2803 w2824 w2838 w2864 w2888 w2909 w2930 w2951 w2972 w3000 w3020 w3047 w3067 w3092 w3111 w3130 w3149 w3168 w3187 w3206 w3225] -> w1148
            tunnel: w1109 -> [w1194 w1213 w1232 w1258 w1315 w1383 w1469 w1533 w1577 w1602 w1623 w1690 w1699 w1736 w1742 w1784 w1813 w1839 w1867 w1896 w1937 w1961 w1999 w2031 w2049 w2069 w2088 w2107 w2126 w2186 w2213 w2246 w2264 w2283 w2302 w2321 w2335 w2402 w2441 w2477 w2488 w2541 w2561 w2591 w2609 w2634 w2666 w2683 w2696 w2720 w2740 w2777 w2821 w2840 w2865 w2884 w2905 w2926 w2947 w2958 w2988 w3007 w3031 w3063 w3080 w3100 w3119 w3138 w3157 w3176 w3195 w3214]
            tunnel: w1104 -> [w1193 w1212 w1231 w1289 w1337 w1403 w1467 w1531 w1575 w1595 w1659 w1689 w1708 w1735 w1750 w1782 w1820 w1845 w1871 w1900 w1940 w1974 w1998 w2029 w2051 w2068 w2087 w2106 w2144 w2188 w2211 w2241 w2265 w2282 w2301 w2320 w2361 w2423 w2455 w2479 w2509 w2537 w2562 w2589 w2608 w2636 w2663 w2682 w2706 w2723 w2739 w2796 w2820 w2841 w2866 w2883 w2904 w2925 w2946 w2959 w2996 w3016 w3027 w3062 w3088 w3107 w3126 w3145 w3164 w3183 w3202 w3221]
            tunnel: [w1194 w1213 w1232 w1258 w1315 w1382 w1469 w1533 w1577 w1602 w1645 w1674 w1699 w1724 w1742 w1784 w1813 w1838 w1866 w1895 w1941 w1960 w2000 w2030 w2049 w2069 w2088 w2107 w2151 w2185 w2212 w2244 w2264 w2283 w2302 w2321 w2362 w2399 w2456 w2476 w2510 w2540 w2563 w2590 w2609 w2637 w2665 w2683 w2695 w2719 w2740 w2775 w2821 w2840 w2865 w2884 w2905 w2926 w2947 w2958 w2988 w3007 w3031 w3063 w3080 w3100 w3119 w3138 w3157 w3176 w3195 w3214] -> w1145
            tunnel: [w1193 w1212 w1231 w1288 w1336 w1398 w1467 w1531 w1575 w1595 w1659 w1688 w1708 w1734 w1750 w1782 w1820 w1845 w1871 w1900 w1940 w1974 w1998 w2029 w2051 w2068 w2087 w2106 w2144 w2188 w2211 w2241 w2265 w2282 w2301 w2320 w2361 w2423 w2455 w2479 w2509 w2537 w2562 w2589 w2608 w2636 w2663 w2682 w2706 w2723 w2739 w2796 w2820 w2841 w2866 w2883 w2904 w2925 w2946 w2959 w2996 w3016 w3030 w3062 w3088 w3107 w3126 w3145 w3164 w3183 w3202 w3221] -> w1158
            tunnel: [_ _ _ _ _ _ _ _ _ _ _ _ _ _ _ _ _ _ _ _ _ _ _ _ _ _ _ _ _ _ _ _ _ _ _ _ _ _ _ w2470 _ _ _ _ _ _ _ _ _ _ _ _ _ _ _ _ _ _ _ _ _ _ _ _ _ _ _ _ _ _ _ _] -> w1120
            tunnel: [_ _ _ _ _ _ _ _ _ _ _ _ _ _ _ _ _ _ _ _ _ _ _ _ _ _ _ _ _ _ _ _ _ _ _ _ _ _ _ w2471 _ _ _ _ _ _ _ _ _ _ _ _ _ _ _ _ _ _ _ _ _ _ _ _ _ _ _ _ _ _ _ _] -> w1122
            tunnel: w1157 -> [w1191 w1210 w1229 w1260 w1317 w1404 w1468 w1532 w1576 w1600 w1660 w1686 w1701 w1732 w1762 w1797 w1830 w1835 w1863 w1892 w1939 w1973 w1995 w2025 w2050 w2066 w2085 w2104 w2150 w2187 w2210 w2239 w2261 w2280 w2299 w2318 w2360 w2419 w2447 w2478 w2490 w2534 w2559 w2587 w2606 w2635 w2662 w2680 w2698 w2725 w2767 w2788 w2818 w2843 w2868 w2881 w2902 w2923 w2944 w2968 w2982 w3009 w3037 w3056 w3082 w3101 w3120 w3139 w3158 w3177 w3196 w3215]
            tunnel: [w1191 w1210 w1229 w1260 w1317 w1404 w1468 w1532 w1576 w1600 w1660 w1686 w1698 w1732 w1762 w1797 w1830 w1835 w1863 w1892 w1939 w1973 w1995 w2025 w2050 w2066 w2085 w2104 w2150 w2187 w2210 w2239 w2261 w2280 w2299 w2318 w2360 w2419 w2447 w2478 w2489 w2534 w2559 w2587 w2606 w2635 w2662 w2680 w2697 w2725 w2767 w2788 w2818 w2843 w2868 w2881 w2902 w2923 w2944 w2968 w2982 w3009 w3037 w3056 w3082 w3101 w3120 w3139 w3158 w3177 w3196 w3215] -> w1156
            tunnel: w1155 -> [w1192 w1211 w1230 w1259 w1316 w1405 w1465 w1529 w1573 w1601 w1661 w1687 w1707 w1733 w1741 w1798 w1831 w1843 w1869 w1898 w1936 w1955 w1996 w2026 w2047 w2067 w2086 w2105 w2149 w2165 w2209 w2240 w2262 w2281 w2300 w2319 w2359 w2420 w2448 w2473 w2507 w2535 w2558 w2588 w2607 w2632 w2661 w2681 w2705 w2724 w2768 w2795 w2819 w2842 w2867 w2882 w2903 w2924 w2945 w2969 w2995 w3015 w3043 w3054 w3087 w3106 w3125 w3144 w3163 w3182 w3201 w3220]
            tunnel: [w1192 w1211 w1230 w1259 w1316 w1405 w1466 w1530 w1574 w1601 w1661 w1687 w1707 w1733 w1741 w1798 w1831 w1843 w1869 w1898 w1936 w1955 w1996 w2026 w2047 w2067 w2086 w2105 w2149 w2165 w2209 w2240 w2262 w2281 w2300 w2319 w2359 w2420 w2448 w2473 w2507 w2535 w2558 w2588 w2607 w2632 w2661 w2681 w2705 w2724 w2768 w2795 w2819 w2842 w2867 w2882 w2903 w2924 w2945 w2969 w2995 w3015 w3043 w3054 w3087 w3106 w3125 w3144 w3163 w3182 w3201 w3220] -> w1154
            tunnel: [_ _ _ _ _ _ _ _ _ _ _ _ _ _ _ _ _ _ _ _ _ _ _ _ _ _ _ _ _ _ _ _ _ _ _ _ _ _ _ _ _ _ _ _ _ _ _ _ _ _ _ _ TRUE _ _ _ _ _ _ _ _ _ _ _ _ _ _ _ _ _ _ _] -> w1151
            tunnel: w1141 -> [w1189 w1208 w1227 w1250 w1310 w1393 w1452 w1516 w1545 _ w1651 w1682 w1706 w1731 w1761 w1796 w1829 w1854 w1880 w1909 w1935 w1972 w1993 w2024 w2045 w2064 w2083 w2102 w2148 w2182 w2207 w2238 w2259 w2278 w2297 w2316 w2358 w2418 w2437 w2469 w2505 w2533 w2556 w2586 w2605 w2630 w2660 w2679 w2703 w2729 w2766 w2792 w2816 w2834 w2861 w2879 w2900 w2921 w2942 w2966 w2993 w3013 w3041 w3060 w3086 w3105 w3124 w3143 w3162 w3181 w3200 w3219]
            tunnel: w1140 -> [w1188 w1207 w1226 w1249 w1309 w1392 w1451 w1515 w1546 _ w1650 w1681 w1705 w1730 w1760 w1795 w1828 w1853 w1879 w1908 w1934 w1971 w1992 w2023 w2044 w2063 w2082 w2101 w2147 w2181 w2206 w2237 w2258 w2277 w2296 w2315 w2357 w2417 w2436 w2468 w2504 w2532 w2555 w2585 w2604 w2629 w2659 w2678 w2702 w2728 w2765 w2791 w2815 w2833 w2860 w2878 w2899 w2920 w2941 w2965 w2992 w3012 w3040 w3059 w3085 w3104 w3123 w3142 w3161 w3180 w3199 w3218]
            tunnel: w1139 -> [w1187 w1206 w1225 w1248 w1308 w1391 w1450 w1514 w1547 _ w1649 w1680 w1704 w1729 w1759 w1794 w1827 w1852 w1878 w1907 w1933 w1970 w1991 w2022 w2043 w2062 w2081 w2100 w2146 w2180 w2205 w2236 w2257 w2276 w2295 w2314 w2356 w2416 w2435 w2467 w2503 w2531 w2554 w2584 w2603 w2628 w2658 w2677 w2701 w2727 w2764 w2790 w2814 w2832 w2859 w2877 w2898 w2919 w2940 w2964 w2991 w3011 w3039 w3058 w3084 w3103 w3122 w3141 w3160 w3179 w3198 w3217]
            tunnel: w1138 -> [w1186 w1205 w1224 w1247 w1307 w1390 w1449 w1513 w1548 _ w1648 w1679 w1703 w1728 w1758 w1793 w1826 w1851 w1877 w1906 w1932 w1969 w1990 w2021 w2042 w2061 w2080 w2099 w2145 w2179 w2204 w2235 w2256 w2275 w2294 w2313 w2355 w2415 w2434 w2466 w2502 w2530 w2553 w2583 w2602 w2627 w2657 w2676 w2700 w2726 w2763 w2789 w2813 w2831 w2858 w2876 w2897 w2918 w2939 w2963 w2990 w3010 w3038 w3057 w3083 w3102 w3121 w3140 w3159 w3178 w3197 w3216]
            tunnel: w1137 -> [_ _ _ _ _ _ _ _ _ _ _ _ _ _ _ _ _ _ _ _ _ _ _ _ _ _ _ _ _ w2184 _ _ _ _ _ _ _ _ _ _ _ _ _ _ _ _ _ _ _ _ _ _ _ _ _ _ _ _ _ _ _ _ _ _ _ _ _ _ _ _ _ _]
            tunnel: w1136 -> [_ _ _ _ _ _ _ _ _ _ _ _ _ _ _ _ _ _ _ _ _ _ _ _ _ _ _ _ _ w2183 _ _ _ _ _ _ _ _ _ _ _ _ _ _ _ _ _ _ _ _ _ _ _ _ _ _ _ _ _ _ _ _ _ _ _ _ _ _ _ _ _ _]
            tunnel: [w1189 w1208 w1227 w1250 w1310 w1393 w1452 w1516 w1545 w1594 w1651 w1682 w1706 w1731 w1761 w1796 w1829 w1854 w1880 w1909 w1935 w1972 w1993 w2024 w2045 w2064 w2083 w2102 w2148 w2182 w2207 w2238 w2259 w2278 w2297 w2316 w2358 w2418 w2437 w2469 w2505 w2533 w2556 w2586 w2605 w2630 w2660 w2679 w2703 w2729 w2766 w2792 w2816 w2834 w2861 w2879 w2900 w2921 w2942 w2966 w2993 w3013 w3041 w3060 w3086 w3105 w3124 w3143 w3162 w3181 w3200 w3219] -> w1133
            tunnel: [w1188 w1207 w1226 w1249 w1309 w1392 w1451 w1515 w1546 w1585 w1650 w1681 w1705 w1730 w1760 w1795 w1828 w1853 w1879 w1908 w1934 w1971 w1992 w2023 w2044 w2063 w2082 w2101 w2147 w2181 w2206 w2237 w2258 w2277 w2296 w2315 w2357 w2417 w2436 w2468 w2504 w2532 w2555 w2585 w2604 w2629 w2659 w2678 w2702 w2728 w2765 w2791 w2815 w2833 w2860 w2878 w2899 w2920 w2941 w2965 w2992 w3012 w3040 w3059 w3085 w3104 w3123 w3142 w3161 w3180 w3199 w3218] -> w1101
            tunnel: [w1187 w1206 w1225 w1248 w1308 w1391 w1450 w1514 w1547 w1593 w1649 w1680 w1704 w1729 w1759 w1794 w1827 w1852 w1878 w1907 w1933 w1970 w1991 w2022 w2043 w2062 w2081 w2100 w2146 w2180 w2205 w2236 w2257 w2276 w2295 w2314 w2356 w2416 w2435 w2467 w2503 w2531 w2554 w2584 w2603 w2628 w2658 w2677 w2701 w2727 w2764 w2790 w2814 w2832 w2859 w2877 w2898 w2919 w2940 w2964 w2991 w3011 w3039 w3058 w3084 w3103 w3122 w3141 w3160 w3179 w3198 w3217] -> w1134
            tunnel: [w1186 w1205 w1224 w1247 w1307 w1390 w1449 w1513 w1548 w1583 w1648 w1679 w1703 w1728 w1758 w1793 w1826 w1851 w1877 w1906 w1932 w1969 w1990 w2021 w2042 w2061 w2080 w2099 w2145 w2179 w2204 w2235 w2256 w2275 w2294 w2313 w2355 w2415 w2434 w2466 w2502 w2530 w2553 w2583 w2602 w2627 w2657 w2676 w2700 w2726 w2763 w2789 w2813 w2831 w2858 w2876 w2897 w2918 w2939 w2963 w2990 w3010 w3038 w3057 w3083 w3102 w3121 w3140 w3159 w3178 w3197 w3216] -> w1135
            tunnel: [_ _ _ _ _ _ _ _ _ _ _ _ _ _ _ _ _ _ _ _ _ _ _ _ _ _ _ _ w2135 w2184 _ _ _ _ _ _ _ _ _ _ _ _ _ _ _ _ _ _ _ _ _ _ _ _ _ _ _ _ _ _ _ _ _ _ _ _ _ _ _ _ _ _] -> w1103
            tunnel: [_ _ _ _ _ _ _ _ _ _ _ _ _ _ _ _ _ _ _ _ _ _ _ _ _ _ _ _ w2134 w2183 _ _ _ _ _ _ _ _ _ _ _ _ _ _ _ _ _ _ _ _ _ _ _ _ _ _ _ _ _ _ _ _ _ _ _ _ _ _ _ _ _ _] -> w1102
            tunnel: w1116 -> [w1185 w1204 w1223 w1246 w1306 w1389 w1448 w1512 w1544 w1592 w1658 w1678 w1702 w1727 w1744 w1786 w1812 w1837 w1865 w1894 w1931 w1968 w1989 w2020 w2041 w2060 w2079 w2098 w2133 w2178 w2203 w2234 w2255 w2274 w2293 w2312 w2354 w2414 w2431 w2465 w2501 w2529 w2550 w2577 w2601 w2624 w2651 w2675 w2694 w2722 w2756 w2787 w2812 w2844 w2869 w2880 w2901 w2922 w2943 w2967 w2994 w3014 w3042 w3061 w3077 w3099 w3118 w3137 w3156 w3175 w3194 w3213]
            tunnel: [w1185 w1204 w1223 w1246 w1306 w1389 w1448 w1512 w1544 w1592 w1658 w1678 w1702 w1727 w1743 w1785 w1805 w1836 w1864 w1893 w1931 w1968 w1989 w2020 w2041 w2060 w2079 w2098 w2133 w2178 w2203 w2234 w2255 w2274 w2293 w2312 w2354 w2414 w2431 w2465 w2501 w2529 w2550 w2577 w2601 w2624 w2651 w2675 w2694 w2721 w2756 w2787 w2812 w2844 w2869 w2880 w2901 w2922 w2943 w2967 w2994 w3014 w3042 w3061 w3077 w3099 w3118 w3137 w3156 w3175 w3194 w3213] -> w1115
            tunnel: [w1184 w1203 w1222 w1245 w1305 w1388 w1447 w1511 w1543 w1591 w1657 w1677 w1713 w1726 w1764 w1792 w1825 w1850 w1876 w1905 w1930 w1967 w1988 w2019 w2040 w2059 w2078 w2097 w2132 w2177 w2202 w2233 w2254 w2273 w2292 w2311 w2353 w2413 w2430 w2464 w2500 w2528 w2549 w2576 w2600 w2623 w2650 w2674 w2693 w2714 w2762 w2786 w2810 w2845 w2855 w2875 w2896 w2917 w2938 w2962 w2998 w3018 w3045 w3065 w3090 w3109 w3128 w3147 w3166 w3185 w3204 w3223] -> w1114
            tunnel: [w1183 w1202 w1221 w1244 w1304 w1387 w1446 w1510 w1542 w1590 w1656 w1676 w1712 w1725 w1763 w1791 w1824 w1849 w1875 w1904 w1929 w1966 w1987 w2018 w2039 w2058 w2077 w2096 w2131 w2176 w2201 w2232 w2253 w2272 w2291 w2310 w2352 w2412 w2429 w2463 w2499 w2527 w2548 w2575 w2599 w2622 w2649 w2673 w2692 w2713 w2761 w2785 w2811 w2827 w2852 w2885 w2906 w2927 w2948 w2970 w2997 w3017 w3044 w3064 w3089 w3108 w3127 w3146 w3165 w3184 w3203 w3222] -> w1113
            tunnel: w1112 -> [w1184 w1203 w1222 w1245 w1305 w1388 w1447 w1511 w1543 w1591 w1657 w1677 w1713 w1726 w1764 w1792 w1825 w1850 w1876 w1905 w1930 w1967 w1988 w2019 w2040 w2059 w2078 w2097 w2132 w2177 w2202 w2233 w2254 w2273 w2292 w2311 w2353 w2413 w2430 w2464 w2500 w2528 w2549 w2576 w2600 w2623 w2650 w2674 w2693 w2714 w2762 w2786 w2810 _ w2855 w2875 w2896 w2917 w2938 w2962 w2998 w3018 w3045 w3065 w3090 w3109 w3128 w3147 w3166 w3185 w3204 w3223]
            tunnel: w1111 -> [w1183 w1202 w1221 w1244 w1304 w1387 w1446 w1510 w1542 w1590 w1656 w1676 w1712 w1725 w1763 w1791 w1824 w1849 w1875 w1904 w1929 w1966 w1987 w2018 w2039 w2058 w2077 w2096 w2131 w2176 w2201 w2232 w2253 w2272 w2291 w2310 w2352 w2412 w2429 w2463 w2499 w2527 w2548 w2575 w2599 w2622 w2649 w2673 w2692 w2713 w2761 w2785 w2811 _ w2852 w2885 w2906 w2927 w2948 w2970 w2997 w3017 w3044 w3064 w3089 w3108 w3127 w3146 w3165 w3184 w3203 w3222]
            tunnel: w1110 -> [_ _ _ _ _ _ _ _ _ _ _ _ _ _ _ _ _ _ _ _ _ _ _ _ _ _ _ _ _ _ _ _ _ _ _ _ _ _ _ _ _ _ _ _ _ _ _ _ _ _ _ _ _ _ _ w2873 w2894 w2915 w2936 w2960 _ _ _ _ _ _ _ _ _ _ _ _]
            tunnel: w1108 -> [_ _ _ _ _ _ _ _ _ _ _ _ _ _ _ _ w1817 _ w1860 w1891 w1919 w1954 w1981 w2011 _ _ _ _ w2115 w2160 w2197 w2226 _ _ _ _ _ _ _ _ _ _ _ _ _ _ _ _ _ _ _ _ _ _ _ _ _ _ _ _ _ _ _ _ _ _ _ _ _ _ _ _]
            tunnel: w1105 -> [_ _ _ _ _ _ _ _ _ _ _ _ _ _ _ _ _ _ _ _ _ _ _ _ _ _ _ _ _ _ _ _ _ _ _ _ _ _ _ _ _ _ _ _ _ _ _ _ _ _ _ _ _ _ _ _ _ _ _ _ _ _ w3032 _ _ _ _ _ _ _ _ _]
            tunnel: [w1182 w1201 w1220 w1243 w1303 w1386 w1445 w1509 w1541 w1589 w1655 w1672 w1696 w1722 w1765 w1790 w1823 w1848 w1874 w1903 w1928 w1965 w1986 w2017 w2038 w2057 w2076 w2095 w2130 w2175 w2200 w2231 w2252 w2271 w2290 w2309 w2348 w2411 w2428 w2462 w2484 w2526 w2547 w2574 w2598 w2621 w2648 w2672 w2691 w2712 w2759 w2772 w2809 w2830 w2854 w2872 w2893 w2914 w2935 w2957 w2977 w3006 w3026 w3053 w3073 w3098 w3117 w3136 w3155 w3174 w3193 w3212] -> w1099
            tunnel: w1100 -> [w1182 w1201 w1220 w1243 w1303 w1386 w1445 w1509 w1541 w1589 w1655 w1672 _ w1722 w1765 w1790 w1823 w1848 w1874 w1903 w1928 w1965 w1986 w2017 w2038 w2057 w2076 w2095 w2130 w2175 w2200 w2231 w2252 w2271 w2290 w2309 w2348 w2411 w2428 w2462 w2484 w2526 w2547 w2574 w2598 w2621 w2648 w2672 w2691 w2712 w2759 w2773 w2809 w2830 w2854 w2872 w2893 w2914 w2935 w2957 w2977 w3006 w3026 w3053 w3073 w3098 w3117 w3136 w3155 w3174 w3193 w3212]
            tunnel: w1098 -> [w1181 w1200 w1219 w1242 w1302 w1385 w1444 w1508 w1540 w1588 w1654 w1671 w1695 w1721 w1757 w1789 w1822 w1847 w1873 w1902 w1927 w1964 w1985 w2016 w2037 w2056 w2075 w2094 w2129 w2174 w2199 w2230 w2251 w2270 w2289 w2308 w2347 w2410 w2427 w2461 w2498 w2525 w2546 w2573 w2597 w2620 w2647 w2671 w2690 w2711 w2758 w2784 w2808 w2829 w2857 w2871 w2892 w2913 w2934 w2956 w2976 w3005 w3025 w3052 w3072 w3097 w3116 w3135 w3154 w3173 w3192 w3211]
            tunnel: w1097 -> [w1180 w1199 w1218 w1241 w1301 w1384 w1443 w1507 w1539 w1587 w1653 w1670 w1694 w1720 w1756 w1788 w1821 w1846 w1872 w1901 w1926 w1963 w1984 w2015 w2036 w2055 w2074 w2093 w2128 w2173 w2198 w2229 w2250 w2269 w2288 w2307 w2346 w2409 w2426 w2460 w2495 w2524 w2545 w2572 w2596 w2619 w2646 w2670 w2689 w2710 w2757 w2783 w2807 w2828 w2856 w2870 w2891 w2912 w2933 w2955 w2975 w3004 w3024 w3051 w3071 w3096 w3115 w3134 w3153 w3172 w3191 w3210]
            tunnel: [w1181 w1200 w1219 w1242 w1302 w1385 w1444 w1508 w1540 w1588 w1654 w1671 w1695 w1721 w1757 w1789 w1822 w1847 w1873 w1902 w1927 w1964 w1985 w2016 w2037 w2056 w2075 w2094 w2129 w2174 w2199 w2230 w2251 w2270 w2289 w2308 w2347 w2410 w2427 w2461 w2497 w2525 w2546 w2573 w2597 w2620 w2647 w2671 w2690 w2711 w2758 w2784 w2808 w2829 w2857 w2871 w2892 w2913 w2934 w2956 w2976 w3005 w3025 w3052 w3072 w3097 w3116 w3135 w3154 w3173 w3192 w3211] -> w1096
            tunnel: [w1180 w1199 w1218 w1241 w1301 w1384 w1443 w1507 w1539 w1587 w1653 w1670 w1694 w1720 w1756 w1788 w1821 w1846 w1872 w1901 w1926 w1963 w1984 w2015 w2036 w2055 w2074 w2093 w2128 w2173 w2198 w2229 w2250 w2269 w2288 w2307 w2346 w2409 w2426 w2460 w2496 w2524 w2545 w2572 w2596 w2619 w2646 w2670 w2689 w2710 w2757 w2783 w2807 w2828 w2856 w2870 w2891 w2912 w2933 w2955 w2975 w3004 w3024 w3051 w3071 w3096 w3115 w3134 w3153 w3172 w3191 w3210] -> w1095
            tunnel: w1094 -> [_ _ _ _ _ _ _ _ _ _ w1646 _ _ _ w1768 w1778 _ _ _ _ _ _ _ _ _ _ _ _ _ w2170 _ _ _ _ _ _ w2344 w2408 _ _ _ _ _ _ _ w2618 _ _ _ _ w2734 _ _ _ _ _ _ _ _ _ _ _ _ _ _ _ _ _ _ _ _ _]
            tunnel: w1093 -> [_ _ _ _ _ _ _ _ _ _ w1647 _ _ _ w1767 w1777 _ _ _ _ _ _ _ _ _ _ _ _ _ w2169 _ _ _ _ _ _ w2345 w2407 _ _ _ _ _ _ _ w2617 _ _ _ _ w2733 _ _ _ _ _ _ _ _ _ _ _ _ _ _ _ _ _ _ _ _ _]
            tunnel: w1091 -> [_ _ _ _ _ _ _ _ _ _ _ _ _ _ _ _ w1816 _ w1859 w1890 w1918 w1953 w1980 w2012 _ _ _ _ w2114 w2159 w2196 w2225 _ _ _ _ _ _ _ _ _ _ _ _ _ _ _ _ _ _ _ _ _ _ _ _ _ _ _ _ _ _ _ _ _ _ _ _ _ _ _ _]
            tunnel: w1090 -> [_ _ _ _ _ _ _ _ _ _ _ _ _ _ _ _ w1815 _ _ w1887 w1921 w1958 w1983 w2013 _ _ _ _ w2120 w2164 w2195 w2228 _ _ _ _ _ _ _ _ _ _ _ _ _ _ _ _ _ _ _ _ _ _ _ _ _ _ _ _ _ _ _ _ _ _ _ _ _ _ _ _]
            tunnel: w1089 -> [_ _ _ _ _ _ _ _ _ _ _ _ _ _ _ _ w1814 _ _ w1886 w1920 w1957 w1982 w2014 _ _ _ _ w2119 w2163 w2194 w2227 _ _ _ _ _ _ _ _ _ _ _ _ _ _ _ _ _ _ _ _ _ _ _ _ _ _ _ _ _ _ _ _ _ _ _ _ _ _ _ _]
            tunnel: [_ _ _ _ _ _ _ _ _ _ _ _ _ _ _ _ w1815 _ w1862 w1887 w1921 w1958 w1983 w2013 _ _ _ _ w2120 w2164 w2195 w2228 _ _ _ _ _ _ _ _ _ _ _ _ _ _ _ _ _ _ _ _ _ _ _ _ _ _ _ _ _ _ _ _ _ _ _ _ _ _ _ _] -> w1088
            tunnel: [_ _ _ _ _ _ _ _ _ _ _ _ _ _ _ _ w1814 _ w1861 w1886 w1920 w1957 w1982 w2014 _ _ _ _ w2119 w2163 w2194 w2227 _ _ _ _ _ _ _ _ _ _ _ _ _ _ _ _ _ _ _ _ _ _ _ _ _ _ _ _ _ _ _ _ _ _ _ _ _ _ _ _] -> w1087
            tunnel: [_ _ _ _ _ _ _ _ _ _ _ _ _ _ _ _ w1817 w1840 w1860 w1891 w1919 w1954 w1981 w2011 _ _ _ _ w2115 w2160 w2197 w2226 _ _ _ _ _ _ _ _ _ _ _ _ _ _ _ _ _ _ _ _ _ _ _ _ _ _ _ _ _ _ _ _ _ _ _ _ _ _ _ _] -> w1086
            tunnel: [_ _ _ _ _ _ _ _ _ _ _ _ _ _ _ _ w1816 w1841 w1859 w1890 w1918 w1953 w1980 w2012 _ _ _ _ w2114 w2159 w2196 w2225 _ _ _ _ _ _ _ _ _ _ _ _ _ _ _ _ _ _ _ _ _ _ _ _ _ _ _ _ _ _ _ _ _ _ _ _ _ _ _ _] -> w1085
            tunnel: [_ _ _ _ _ _ _ _ _ _ _ _ _ _ _ _ _ _ _ _ _ w1952 _ _ _ _ _ _ _ w2161 _ _ _ _ _ _ w2327 w2386 _ _ _ _ _ _ _ _ _ _ _ _ _ _ _ _ _ _ _ _ _ _ _ _ _ _ _ _ _ _ _ _ _ _] -> w1082
            tunnel: [_ _ _ _ _ _ _ _ _ _ _ _ _ _ _ _ _ _ _ _ _ w1951 _ _ _ _ _ _ _ w2162 _ _ _ _ _ _ w2326 w2387 _ _ _ _ _ _ _ _ _ _ _ _ _ _ _ _ _ _ _ _ _ _ _ _ _ _ _ _ _ _ _ _ _ _] -> w1084
            tunnel: [_ _ _ _ _ _ _ _ _ _ _ _ _ _ _ _ _ _ w1858 w1889 _ _ _ _ _ _ _ _ _ _ _ _ _ _ _ _ _ _ _ _ _ _ _ _ _ _ _ _ _ _ _ _ _ _ _ _ _ _ _ _ _ _ _ _ _ _ _ _ _ _ _ _] -> w1079
            tunnel: [_ _ _ _ _ _ _ _ _ _ _ _ _ _ _ _ _ _ _ TRUE ("Recording") _ _ _ _ _ _ _ _ _ _ _ _ _ _ _ _ _ _ _ _ _ _ _ _ _ _ _ _ _ _ _ _ _ _ _ _ _ _ _ _ _ _ _ _ _ _ _ _ _ _ _ _] -> w1076
            tunnel: [_ _ _ _ _ _ _ _ _ _ _ _ _ _ _ _ _ _ w1858 _ _ _ _ _ _ _ _ _ _ _ _ _ _ _ _ _ _ _ _ _ _ _ _ _ _ _ _ _ _ _ _ _ _ _ _ _ _ _ _ _ _ _ _ _ _ _ _ _ _ _ _ _] -> w1072
            tunnel: [_ _ _ _ _ _ _ _ _ _ _ TRUE _ _ _ _ _ _ _ _ _ _ _ _ _ _ _ _ _ _ _ _ _ _ _ _ _ _ _ _ _ _ _ _ _ _ _ _ _ _ _ _ _ _ _ _ _ _ _ _ _ _ _ _ _ _ _ _ _ _ _ _] -> w1069
            tunnel: [_ _ _ _ _ _ _ _ _ _ _ w1667 _ _ _ _ _ _ _ _ _ _ _ _ _ _ _ _ _ _ _ _ _ _ _ _ _ _ _ _ _ _ _ _ _ _ _ _ _ _ _ _ _ _ _ _ _ _ _ _ _ _ _ _ _ _ _ _ _ _ _ _] -> w1067
            tunnel: [_ _ _ _ _ _ _ _ _ _ _ _ _ TRUE _ _ _ _ _ _ _ _ _ _ _ _ _ _ _ _ _ _ _ _ _ _ _ _ _ _ _ _ _ _ _ _ _ _ _ _ _ _ _ _ _ _ _ _ _ _ _ _ _ _ _ _ _ _ _ _ _ _] -> w1066
            tunnel: [_ _ _ _ _ _ _ _ _ _ _ _ _ w1714 _ _ _ _ _ _ _ _ _ _ _ _ _ _ _ _ _ _ _ _ _ _ _ _ _ _ _ _ _ _ _ _ _ _ _ _ _ _ _ _ _ _ _ _ _ _ _ _ _ _ _ _ _ _ _ _ _ _] -> w1065
            tunnel: w1053 -> [_ _ _ _ _ _ _ _ _ _ _ _ _ _ _ _ w1803 _ _ _ w1914 w1950 w1979 w2010 _ _ _ _ w2113 w2158 w2193 w2224 _ _ _ _ w2330 w2381 _ _ _ _ _ _ _ _ _ _ _ _ _ _ _ _ _ _ _ _ _ _ _ _ _ _ _ _ _ _ _ _ _ _]
            tunnel: [_ _ _ _ _ _ _ _ _ _ _ _ _ _ _ _ w1803 _ _ w1885 w1914 w1950 w1979 w2010 _ _ _ _ w2113 w2158 w2193 w2224 _ _ _ _ w2330 w2381 _ _ _ _ _ _ _ _ _ _ _ _ _ _ _ _ _ _ _ _ _ _ _ _ _ _ _ _ _ _ _ _ _ _] -> w1052
            tunnel: w1051 -> [_ _ _ _ _ _ _ _ _ _ _ _ _ _ _ _ w1802 _ _ _ w1913 w1949 w1978 w2009 _ _ _ _ w2112 w2157 w2192 w2223 _ _ _ _ w2328 w2385 _ _ _ _ _ _ _ _ _ _ _ _ _ _ _ _ _ _ _ _ _ _ _ _ _ _ _ _ _ _ _ _ _ _]
            tunnel: [_ _ _ _ _ _ _ _ _ _ _ _ _ _ _ _ w1802 _ _ w1884 w1913 w1949 w1978 w2009 _ _ _ _ w2112 w2157 w2192 w2223 _ _ _ _ w2328 w2385 _ _ _ _ _ _ _ _ _ _ _ _ _ _ _ _ _ _ _ _ _ _ _ _ _ _ _ _ _ _ _ _ _ _] -> w1050
            frame "Start1", Default {
            }
            frame "Start2" {
            }
            frame "Start3" {
            }
            frame "saveSettings1" {
              n604 = call "myRIO_BRig_RT_dataExp_Audio_freq__L.vi"() -> ("output_Audio_freq__L"=w1266:i32)  [unwired: 11 in]
              n605 = call "myRIO_BRig_RT_dataExp_Audio_freq__R.vi"() -> ("output_Audio_freq__R"=w1265:i32)  [unwired: 11 in]
              n606 = call "myRIO_BRig_RT_dataExp_Audio_amp__L.vi"() -> ("output_Audio_amp__L"=w1264:i32)  [unwired: 11 in]
              n607 = call "myRIO_BRig_RT_dataExp_Audio_amp__R.vi"() -> ("output_Audio_amp__R"=w1262:i32)  [unwired: 11 in]
              n608 = call "myRIO_BRig_RT_dataExp_TPB_min__L.vi"() -> ("output_TPB_min__L"=w1274:i32)  [unwired: 11 in]
              n609 = call "myRIO_BRig_RT_dataExp_TPB_min__R.vi"() -> ("output_TPB_min__R"=w1272:i32)  [unwired: 11 in]
              n610 = call "myRIO_BRig_RT_dataExp_TPB_max__L.vi"() -> ("output_TPB_max__L"=w1270:i32)  [unwired: 11 in]
              n611 = call "myRIO_BRig_RT_dataExp_TPB_max__R.vi"() -> ("output_TPB_max__R"=w1268:i32)  [unwired: 11 in]
              n612 = call "myRIO_BRig_RT_dataExp_ItrialUntilReward.vi"() -> ("output_I_trialUntilReward"=w1287:i32)  [unwired: 11 in]
              n613 = call "myRIO_BRig_RT_dataExp_IblockUntilReward.vi"() -> ("output_I_blockUntilReward"=w1283:i32)  [unwired: 11 in]
              n614 = call "myRIO_BRig_RT_dataExp_CueCycles.vi"() -> ("output_CueCycles"=w1282:i32)  [unwired: 11 in]
              n615 = call "myRIO_BRig_RT_dataExp_ENL_min.vi"() -> ("output_ENL_min"=w1280:i32)  [unwired: 11 in]
              n616 = call "myRIO_BRig_RT_dataExp_ENL_max.vi"() -> ("output_ENL_max"=w1278:i32)  [unwired: 11 in]
              n617 = call "myRIO_BRig_RT_dataExp_ENL_penalty.vi"() -> ("output_ENL_penalty"=w1276:i32)  [unwired: 11 in]
              n618 = local read "Audio_Freq__L"() -> (w1240:u8)
              n619 = local read "Audio_Freq__R"() -> (w1238:u8)
              n620 = local read "Audio_Amp__L"() -> (w1263:u16)
              n621 = local read "TpB_Min_L"() -> (w1273:u16)
              n622 = local read "TpB_Min_R"() -> (w1271:u16)
              n623 = local read "TpB_Max_L"() -> (w1269:u16)
              n624 = local read "TpB_Max_R"() -> (w1267:u16)
              n625 = local read "Audio_Amp__R"() -> (w1261:u16)
              n626 = local read "TrialUntilReward"() -> (w1286:bool)
              n627 = local read "CueCycles"() -> (w1281:u16)
              n628 = local read "Tcycle_ENL_min"() -> (w1279:u16)
              n629 = local read "Tcycle_ENL_max"() -> (w1277:u16)
              n630 = local read "Tcycle_ENLPenalty"() -> (w1275:u16)
              n631 = To Unsigned Word Integer(number=w1238) -> (unsigned 16bit integer=w1237:u16)
              n632 = To Unsigned Word Integer(number=w1240) -> (unsigned 16bit integer=w1239:u16)
              n633 = Boolean To (0,1)(Boolean=w1286) -> (0, 1=w1285:i16)
              n634 = To Unsigned Word Integer(number=w1285) -> (unsigned 16bit integer=w1284:u16)
              n635 = local read "BUR_min"() -> (w1255:u16)
              n636 = local read "BUR_max"() -> (w1256:u16)
              n637 = Not Equal To 0?(x=w1255) -> (x != 0?=w1254:bool)
              n638 = Not Equal To 0?(x=w1256) -> (x != 0?=w1253:bool)
              n639 = And(x=w1254, y=w1253) -> (x .and. y?=w1252:bool)
              n640 = Boolean To (0,1)(Boolean=w1252) -> (0, 1=w1257:i16)
              n641 = To Unsigned Word Integer(number=w1257) -> (unsigned 16bit integer=w1251:u16)
              n642 = Replace Array Subset(array=w1289, new element #1=w1284, index #1=w1287, new element #2=w1251, index #2=w1283, new element #3=w1281, index #3=w1282, new element #4=w1279, index #4=w1280, new element #5=w1277, index #5=w1278, new element #6=w1275, index #6=w1276, new element #7=w1273, index #7=w1274, new element #8=w1271, index #8=w1272, new element #9=w1269, index #9=w1270, new element #10=w1267, index #10=w1268, new element #11=w1239, index #11=w1266, new element #12=w1237, index #12=w1265, new element #13=w1263, index #13=w1264, new element #14=w1261, index #14=w1262) -> (w1288:u16[])
            }
            frame "saveSettings2" {
              n643 = call "myRIO_BRig_RT_dataExp_Tcycle_RewardPost.vi"() -> ("output_Tcycle_RewardPost"=w1326:i32)  [unwired: 11 in]
              n644 = call "myRIO_BRig_RT_dataExp_Tcycle_Wrong.vi"() -> ("output_Tcycle_Wrong"=w1324:i32)  [unwired: 11 in]
              n645 = call "myRIO_BRig_RT_dataExp_Tcycle_Timeout.vi"() -> ("output_Tcycle_Timeout"=w1322:i32)  [unwired: 11 in]
              n646 = call "myRIO_BRig_RT_dataExp_Tcycle_Cue_min.vi"() -> ("output_Tcycle_Cue_min"=w1320:i32)  [unwired: 11 in]
              n647 = call "myRIO_BRig_RT_dataExp_Tcycle_Cue_max.vi"() -> ("output_Tcycle_Cue_max"=w1319:i32)  [unwired: 11 in]
              n648 = call "myRIO_BRig_RT_dataExp_Tcycle_CuePenalty.vi"() -> ("output_Tcycle_CuePenalty"=w1318:i32)  [unwired: 11 in]
              n649 = call "myRIO_BRig_RT_dataExp_SolenoidProbability_L.vi"() -> ("output_SolenoidProbability_L"=w1298:i32)  [unwired: 11 in]
              n650 = call "myRIO_BRig_RT_dataExp_SolenoidProbability_R.vi"() -> ("output_SolenoidProbability_R"=w1297:i32)  [unwired: 11 in]
              n651 = call "myRIO_BRig_RT_dataExp_nBlock.vi"() -> ("output_nBlock"=w1335:i32)  [unwired: 11 in]
              n652 = call "myRIO_BRig_RT_dataExp_nTrial.vi"() -> ("output_nTrial"=w1334:i32)  [unwired: 11 in]
              n653 = call "myRIO_BRig_RT_dataExp_runTime_seconds.vi"() -> ("output_RunTime_minutes"=w1333:i32)  [unwired: 11 in]
              n654 = call "myRIO_BRig_RT_dataExp_Tcycle_Selection.vi"() -> ("output_Tcycle_Selection"=w1332:i32)  [unwired: 11 in]
              n655 = call "myRIO_BRig_RT_dataExp_Tcycle_Reward__L.vi"() -> ("output_Tcycle_Reward__L"=w1330:i32)  [unwired: 11 in]
              n656 = call "myRIO_BRig_RT_dataExp_Tcycle_Reward__R.vi"() -> ("output_Tcycle_Reward__R"=w1328:i32)  [unwired: 11 in]
              n657 = local read "Tcycle_RewardPost"() -> (w1325:u16)
              n658 = local read "Tcycle_Wrong"() -> (w1323:u16)
              n659 = local read "Tcycle_Timeout"() -> (w1321:u16)
              n660 = local read "Tcycle_CuePenalty"() -> (w1311:u16)
              n661 = local read "Tcycle_Cue_max"() -> (w1299:u16)
              n662 = local read "Tcycle_Cue_min"() -> (w1300:u16)
              n663 = local read "Tcycle_Selection"() -> (w1331:u16)
              n664 = local read "Tcycle_Reward_L"() -> (w1329:u16)
              n665 = local read "Tcycle_Reward_R"() -> (w1327:u16)
              n666 = local read "SolenoidProbability_R"() -> (w1295:u16)
              n667 = local read "SolenoidProbability_L"() -> (w1296:u16)
              n668 = Replace Array Subset(array=w1337, new element #1=u16 0, index #1=w1335, new element #2=u16 0, index #2=w1334, new element #3=u16 0, index #3=w1333, new element #4=w1331, index #4=w1332, new element #5=w1329, index #5=w1330, new element #6=w1327, index #6=w1328, new element #7=w1325, index #7=w1326, new element #8=w1323, index #8=w1324, new element #9=w1321, index #9=w1322, new element #10=w1300, index #10=w1320, new element #11=w1299, index #11=w1319, new element #12=w1311, index #12=w1318, new element #13=w1296, index #13=w1298, new element #14=w1295, index #14=w1297) -> (w1336:u16[])
            }
            frame "saveSettings3" {
              w1347 = 100.0 ("y")
              n669 = call "myRIO_BRig_RT_dataExp_laser_Freq.vi"() -> ("output_laser_Freq"=w1380:i32)  [unwired: 11 in]
              n670 = call "myRIO_BRig_RT_dataExp_laser_Tpeak.vi"() -> ("output_laser_Tpeak"=w1375:i32)  [unwired: 11 in]
              n671 = call "myRIO_BRig_RT_dataExp_laser_Tshutter.vi"() -> ("output_laser_Tshutter"=w1370:i32)  [unwired: 11 in]
              n672 = call "myRIO_BRig_RT_dataExp_laser_f_millisec2count.vi"() -> ("output_laser_f_millisec2count"=w1365:i32)  [unwired: 11 in]
              n673 = call "myRIO_BRig_RT_dataExp_laser_Power_min.vi"() -> ("output_laser_Power_min"=w1360:i32)  [unwired: 11 in]
              n674 = call "myRIO_BRig_RT_dataExp_laser_Power_max.vi"() -> ("output_laser_Power_max"=w1353:i32)  [unwired: 11 in]
              n675 = call "myRIO_BRig_RT_dataExp_laser_Power_step.vi"() -> ("output_laser_Power_step"=w1352:i32)  [unwired: 11 in]
              n676 = call "myRIO_BRig_RT_dataExp_laser_duration.vi"() -> ("output_laser_duration"=w1355:i32)  [unwired: 11 in]
              n677 = call "myRIO_BRig_RT_dataExp_BUR_min.vi"() -> ("output_BUR_min"=w1402:i32)  [unwired: 11 in]
              n678 = call "myRIO_BRig_RT_dataExp_BUR_max.vi"() -> ("output_BUR_max"=w1400:i32)  [unwired: 11 in]
              n679 = call "myRIO_BRig_RT_dataExp_Audio_sp__L.vi"() -> ("output_Audio_sp__L"=w1397:i32)  [unwired: 11 in]
              n680 = call "myRIO_BRig_RT_dataExp_Audio_sp__R.vi"() -> ("output_Audio_sp__R"=w1396:i32)  [unwired: 11 in]
              n681 = local read "laser_Tshutter"() -> (w1367:dbl)
              n682 = local read "f_millisec2count"() -> (w1362:dbl)
              n683 = local read "laser_Tpeak"() -> (w1372:dbl)
              n684 = local read "laser_power_min"() -> (w1357:dbl)
              n685 = local read "laser_power_max"() -> (w1346:dbl)
              n686 = local read "laser_power_step"() -> (w1345:dbl)
              n687 = local read "laser_Freq"() -> (w1379:dbl)
              n688 = local read "sp_LeftSpout"() -> (w1395:u16)
              n689 = local read "BUR_max"() -> (w1399:u16)
              n690 = local read "sp_RightSpout"() -> (w1394:u16)
              n691 = local read "BUR_min"() -> (w1401:u16)
              n692 = Multiply(x=w1379, y=w1347) -> (x*y=w1378:dbl)
              n693 = Multiply(x=w1372, y=w1347) -> (x*y=w1374:dbl)
              n694 = Multiply(x=w1367, y=w1347) -> (x*y=w1369:dbl)
              n695 = Multiply(x=w1362, y=w1347) -> (x*y=w1364:dbl)
              n696 = Multiply(x=w1357, y=w1347) -> (x*y=w1359:dbl)
              n697 = Multiply(x=w1346, y=w1347) -> (x*y=w1351:dbl)
              n698 = Multiply(x=w1345, y=w1347) -> (x*y=w1349:dbl)
              n699 = Round To Nearest(number=w1378) -> (nearest integer value=w1377:dbl)
              n700 = Round To Nearest(number=w1374) -> (nearest integer value=w1373:dbl)
              n701 = Round To Nearest(number=w1369) -> (nearest integer value=w1368:dbl)
              n702 = Round To Nearest(number=w1364) -> (nearest integer value=w1363:dbl)
              n703 = Round To Nearest(number=w1359) -> (nearest integer value=w1358:dbl)
              n704 = Round To Nearest(number=w1351) -> (nearest integer value=w1350:dbl)
              n705 = Round To Nearest(number=w1349) -> (nearest integer value=w1348:dbl)
              n706 = To Unsigned Word Integer(number=w1377) -> (unsigned 16bit integer=w1376:u16)
              n707 = To Unsigned Word Integer(number=w1373) -> (unsigned 16bit integer=w1371:u16)
              n708 = To Unsigned Word Integer(number=w1368) -> (unsigned 16bit integer=w1366:u16)
              n709 = To Unsigned Word Integer(number=w1363) -> (unsigned 16bit integer=w1361:u16)
              n710 = To Unsigned Word Integer(number=w1358) -> (unsigned 16bit integer=w1356:u16)
              n711 = To Unsigned Word Integer(number=w1350) -> (unsigned 16bit integer=w1344:u16)
              n712 = To Unsigned Word Integer(number=w1348) -> (unsigned 16bit integer=w1343:u16)
              n713 = local read "laser_duration"() -> (w1354:u16)
              n714 = call "myRIO_BRig_RT_dataCurrent_LaserPulse_duration.vi"() -> ("output_LaserPulse_duration"=w1381:i32)  [unwired: 11 in]
              n715 = Replace Array Subset(array=w1403, new element #1=w1401, index #1=w1402, new element #2=w1399, index #2=w1400, new element #3=w1395, index #3=w1397, new element #4=w1394, index #4=w1396, new element #5=w1376, index #5=w1380, new element #6=w1371, index #6=w1375, new element #7=w1366, index #7=w1370, new element #8=w1361, index #8=w1365, new element #9=w1356, index #9=w1360, new element #10=w1344, index #10=w1353, new element #11=w1343, index #11=w1352, new element #12=w1354, index #12=w1355) -> (w1398:u16[])
              n716 = Replace Array Subset(array=w1383, new element=w1354, index=w1381) -> (w1382:u16[])
            }
            frame "saveSettings4_LC_ENL" {
              # "Selection First"
              # "Count"
              # "Tdelay"
              # "Probability"
              # "OnOff"
              # "Block"
              # "delayOpt"
              # "Count"
              # "Tdelay"
              # "Probability"
              # "OnOff"
              # "Block"
              # "ENL1 All"
              # "delayOpt"
              # "Count"
              # "Tdelay"
              # "Probability"
              # "OnOff"
              # "Block"
              # "ENL1 First"
              n717 = call "myRIO_BRig_RT_dataLC_ENL1_All_Block.vi"() -> ("output_ENL1_All_Block"=w1438:i32)  [unwired: 11 in]
              n718 = call "myRIO_BRig_RT_dataLC_ENL1_All_OnOff.vi"() -> ("output_ENL1_All_OnOff"=w1428:i32)  [unwired: 11 in]
              n719 = call "myRIO_BRig_RT_dataLC_ENL1_All_Probability.vi"() -> ("output_ENL1_All_Probability"=w1427:i32)  [unwired: 11 in]
              n720 = call "myRIO_BRig_RT_dataLC_ENL1_All_Tdelay.vi"() -> ("output_ENL1_All_Tdelay"=w1426:i32)  [unwired: 11 in]
              n721 = call "myRIO_BRig_RT_dataLC_ENL1_All_Count.vi"() -> ("output_ENL1_All_Count"=w1425:i32)  [unwired: 11 in]
              n722 = call "myRIO_BRig_RT_dataLC_ENL1_All_delayOpt.vi"() -> ("output_ENL1_All_delayOpt"=w1424:i32)  [unwired: 11 in]
              n723 = call "myRIO_BRig_RT_dataLC_ENL1_First_Block.vi"() -> ("output_ENL1_First_Block"=w1464:i32)  [unwired: 11 in]
              n724 = call "myRIO_BRig_RT_dataLC_ENL1_First_OnOff.vi"() -> ("output_ENL1_First_OnOff"=w1462:i32)  [unwired: 11 in]
              n725 = call "myRIO_BRig_RT_dataLC_ENL1_First_Probability.vi"() -> ("output_ENL1_First_Probability"=w1458:i32)  [unwired: 11 in]
              n726 = call "myRIO_BRig_RT_dataLC_ENL1_First_Tdelay.vi"() -> ("output_ENL1_First_Tdelay"=w1456:i32)  [unwired: 11 in]
              n727 = call "myRIO_BRig_RT_dataLC_ENL1_First_Count.vi"() -> ("output_ENL1_First_Count"=w1454:i32)  [unwired: 11 in]
              n728 = call "myRIO_BRig_RT_dataLC_ENL1_First_delayOpt.vi"() -> ("output_ENL1_First_delayOpt"=w1440:i32)  [unwired: 11 in]
              n729 = local read "LC_ENL1_First_delayOpt"() -> (w1441:bool)
              n730 = local read "LC_ENL1_First_Count"() -> (w1453:u16)
              n731 = call "myRIO_BRig_RT_dataLC_Selection_First_Block.vi"() -> ("output_Selection_First_Block"=w1422:i32)  [unwired: 11 in]
              n732 = call "myRIO_BRig_RT_dataLC_Selection_First_OnOff.vi"() -> ("output_Selection_First_OnOff"=w1421:i32)  [unwired: 11 in]
              n733 = call "myRIO_BRig_RT_dataLC_Selection_First_Probability.vi"() -> ("output_Selection_First_Probability"=w1420:i32)  [unwired: 11 in]
              n734 = call "myRIO_BRig_RT_dataLC_Selection_First_Tdelay.vi"() -> ("output_Selection_First_Tdelay"=w1419:i32)  [unwired: 11 in]
              n735 = call "myRIO_BRig_RT_dataLC_Selection_First_Count.vi"() -> ("output_Selection_First_Count"=w1418:i32)  [unwired: 11 in]
              n736 = local read "LC_ENL1_First_Probability"() -> (w1457:u16)
              n737 = local read "LC_ENL1_First_Block"() -> (w1463:u16)
              n738 = local read "LC_ENL1_First_Tdelay"() -> (w1455:u16)
              n739 = local read "LC_ENL1_First_OnOff"() -> (w1461:bool)
              n740 = local read "LC_ENL1_All_OnOff"() -> (w1434:bool)
              n741 = local read "LC_ENL1_All_Probability"() -> (w1432:u16)
              n742 = local read "LC_ENL1_All_delayOpt"() -> (w1430:bool)
              n743 = local read "LC_ENL1_All_Tdelay"() -> (w1423:u16)
              n744 = local read "LC_ENL1_All_Block"() -> (w1435:u16)
              n745 = local read "LC_ENL1_All_Count"() -> (w1431:u16)
              n746 = local read "LC_Sel_First_Probability"() -> (w1413:u16)
              n747 = local read "LC_Sel_First_Tdelay"() -> (w1412:u16)
              n748 = local read "LC_Sel_First_OnOff"() -> (w1416:bool)
              n749 = local read "LC_Sel_First_Count"() -> (w1411:u16)
              n750 = local read "LC_Sel_First_Block"() -> (w1415:u16)
              n751 = Boolean To (0,1)(Boolean=w1441) -> (0, 1=w1442:i16)
              n752 = Boolean To (0,1)(Boolean=w1461) -> (0, 1=w1460:i16)
              n753 = Boolean To (0,1)(Boolean=w1434) -> (0, 1=w1437:i16)
              n754 = To Unsigned Word Integer(number=w1442) -> (unsigned 16bit integer=w1439:u16)
              n755 = To Unsigned Word Integer(number=w1460) -> (unsigned 16bit integer=w1459:u16)
              n756 = Boolean To (0,1)(Boolean=w1430) -> (0, 1=w1436:i16)
              n757 = To Unsigned Word Integer(number=w1437) -> (unsigned 16bit integer=w1433:u16)
              n758 = Boolean To (0,1)(Boolean=w1416) -> (0, 1=w1417:i16)
              n759 = To Unsigned Word Integer(number=w1436) -> (unsigned 16bit integer=w1429:u16)
              n760 = To Unsigned Word Integer(number=w1417) -> (unsigned 16bit integer=w1414:u16)
              n761 = Replace Array Subset(array=w1465, new element #1=w1463, index #1=w1464, new element #2=w1459, index #2=w1462, new element #3=w1457, index #3=w1458, new element #4=w1455, index #4=w1456, new element #5=w1453, index #5=w1454, new element #6=w1439, index #6=w1440, new element #7=w1435, index #7=w1438, new element #8=w1433, index #8=w1428, new element #9=w1432, index #9=w1427, new element #10=w1423, index #10=w1426, new element #11=w1431, index #11=w1425, new element #12=w1429, index #12=w1424, new element #13=w1415, index #13=w1422, new element #14=w1414, index #14=w1421, new element #15=w1413, index #15=w1420, new element #16=w1412, index #16=w1419, new element #17=w1411, index #17=w1418) -> (w1466:u16[])
            }
            frame "saveSettings5_LC_Cue" {
              # "Selection All"
              # "Count"
              # "Tdelay"
              # "Probability"
              # "OnOff"
              # "Block"
              # "delayOpt"
              # "Count"
              # "Tdelay"
              # "Probability"
              # "OnOff"
              # "Block"
              # "Cue1 All"
              # "delayOpt"
              # "Count"
              # "Tdelay"
              # "Probability"
              # "OnOff"
              # "Block"
              # "Cue1 First"
              n762 = call "myRIO_BRig_RT_dataLC_Cue1_First_delayOpt.vi"() -> ("output_Cue1_First_delayOpt"=w1505:i32)  [unwired: 11 in]
              n763 = call "myRIO_BRig_RT_dataLC_Cue1_First_Block.vi"() -> ("output_Cue1_First_Block"=w1528:i32)  [unwired: 11 in]
              n764 = call "myRIO_BRig_RT_dataLC_Cue1_First_OnOff.vi"() -> ("output_Cue1_First_OnOff"=w1526:i32)  [unwired: 11 in]
              n765 = call "myRIO_BRig_RT_dataLC_Cue1_First_Probability.vi"() -> ("output_Cue1_First_Probability"=w1522:i32)  [unwired: 11 in]
              n766 = call "myRIO_BRig_RT_dataLC_Cue1_First_Tdelay.vi"() -> ("output_Cue1_First_Tdelay"=w1520:i32)  [unwired: 11 in]
              n767 = call "myRIO_BRig_RT_dataLC_Cue1_First_Count.vi"() -> ("output_Cue1_First_Count"=w1518:i32)  [unwired: 11 in]
              n768 = call "myRIO_BRig_RT_dataLC_Cue1_All_Block.vi"() -> ("output_Cue1_All_Block"=w1502:i32)  [unwired: 11 in]
              n769 = call "myRIO_BRig_RT_dataLC_Cue1_All_OnOff.vi"() -> ("output_Cue1_All_OnOff"=w1501:i32)  [unwired: 11 in]
              n770 = call "myRIO_BRig_RT_dataLC_Cue1_All_Probability.vi"() -> ("output_Cue1_All_Probability"=w1500:i32)  [unwired: 11 in]
              n771 = call "myRIO_BRig_RT_dataLC_Cue1_All_Tdelay.vi"() -> ("output_Cue1_All_Tdelay"=w1499:i32)  [unwired: 11 in]
              n772 = call "myRIO_BRig_RT_dataLC_Cue1_All_Count.vi"() -> ("output_Cue1_All_Count"=w1498:i32)  [unwired: 11 in]
              n773 = call "myRIO_BRig_RT_dataLC_Cue1_All_delayOpt.vi"() -> ("output_Cue1_All_delayOpt"=w1497:i32)  [unwired: 11 in]
              n774 = local read "LC_Cue1_First_delayOpt"() -> (w1504:bool)
              n775 = local read "LC_Cue1_First_Count"() -> (w1517:u16)
              n776 = local read "LC_Cue1_First_Probability"() -> (w1521:u16)
              n777 = local read "LC_Cue1_First_Block"() -> (w1527:u16)
              n778 = local read "LC_Cue1_First_Tdelay"() -> (w1519:u16)
              n779 = local read "LC_Cue1_First_OnOff"() -> (w1525:bool)
              n780 = call "myRIO_BRig_RT_dataLC_Selection_All_Block.vi"() -> ("output_Selection_All_Block"=w1486:i32)  [unwired: 11 in]
              n781 = call "myRIO_BRig_RT_dataLC_Selection_All_OnOff.vi"() -> ("output_Selection_All_OnOff"=w1485:i32)  [unwired: 11 in]
              n782 = call "myRIO_BRig_RT_dataLC_Selection_All_Probability.vi"() -> ("output_Selection_All_Probability"=w1484:i32)  [unwired: 11 in]
              n783 = call "myRIO_BRig_RT_dataLC_Selection_All_Tdelay.vi"() -> ("output_Selection_All_Tdelay"=w1483:i32)  [unwired: 11 in]
              n784 = call "myRIO_BRig_RT_dataLC_Selection_All_Count.vi"() -> ("output_Selection_All_Count"=w1476:i32)  [unwired: 11 in]
              n785 = local read "LC_Cue1_All_OnOff"() -> (w1493:bool)
              n786 = local read "LC_Cue1_All_delayOpt"() -> (w1494:bool)
              n787 = local read "LC_Cue1_All_Probability"() -> (w1490:u16)
              n788 = local read "LC_Cue1_All_Tdelay"() -> (w1489:u16)
              n789 = local read "LC_Cue1_All_Count"() -> (w1488:u16)
              n790 = local read "LC_Cue1_All_Block"() -> (w1492:u16)
              n791 = local read "LC_Sel_All_Probability"() -> (w1478:u16)
              n792 = local read "LC_Sel_All_Tdelay"() -> (w1477:u16)
              n793 = local read "LC_Sel_All_OnOff"() -> (w1480:bool)
              n794 = local read "LC_Sel_All_Count"() -> (w1475:u16)
              n795 = local read "LC_Sel_All_Block"() -> (w1482:u16)
              n796 = Boolean To (0,1)(Boolean=w1504) -> (0, 1=w1506:i16)
              n797 = Boolean To (0,1)(Boolean=w1525) -> (0, 1=w1524:i16)
              n798 = Boolean To (0,1)(Boolean=w1493) -> (0, 1=w1496:i16)
              n799 = To Unsigned Word Integer(number=w1506) -> (unsigned 16bit integer=w1503:u16)
              n800 = To Unsigned Word Integer(number=w1524) -> (unsigned 16bit integer=w1523:u16)
              n801 = To Unsigned Word Integer(number=w1496) -> (unsigned 16bit integer=w1491:u16)
              n802 = Boolean To (0,1)(Boolean=w1494) -> (0, 1=w1495:i16)
              n803 = Boolean To (0,1)(Boolean=w1480) -> (0, 1=w1481:i16)
              n804 = To Unsigned Word Integer(number=w1495) -> (unsigned 16bit integer=w1487:u16)
              n805 = To Unsigned Word Integer(number=w1481) -> (unsigned 16bit integer=w1479:u16)
              n806 = Replace Array Subset(array=w1529, new element #1=w1527, index #1=w1528, new element #2=w1523, index #2=w1526, new element #3=w1521, index #3=w1522, new element #4=w1519, index #4=w1520, new element #5=w1517, index #5=w1518, new element #6=w1503, index #6=w1505, new element #7=w1492, index #7=w1502, new element #8=w1491, index #8=w1501, new element #9=w1490, index #9=w1500, new element #10=w1489, index #10=w1499, new element #11=w1488, index #11=w1498, new element #12=w1487, index #12=w1497, new element #13=w1482, index #13=w1486, new element #14=w1479, index #14=w1485, new element #15=w1478, index #15=w1484, new element #16=w1477, index #16=w1483, new element #17=w1475, index #17=w1476) -> (w1530:u16[])
            }
            frame "saveSettings6_LC_Other" {
              # "Trial"
              # "Tdelay"
              # "Probability"
              # "OnOff"
              # "Block"
              # "Wrong"
              # "Trial"
              # "Tdelay"
              # "Probability"
              # "OnOff"
              # "Block"
              # "Reward"
              n807 = call "myRIO_BRig_RT_dataLC_Wrong_Block.vi"() -> ("output_Wrong_Block"=w1560:i32)  [unwired: 11 in]
              n808 = call "myRIO_BRig_RT_dataLC_Wrong_OnOff.vi"() -> ("output_Wrong_OnOff"=w1559:i32)  [unwired: 11 in]
              n809 = call "myRIO_BRig_RT_dataLC_Wrong_Probability.vi"() -> ("output_Wrong_Probability"=w1558:i32)  [unwired: 11 in]
              n810 = call "myRIO_BRig_RT_dataLC_Wrong_Tdelay.vi"() -> ("output_Wrong_Tdelay"=w1557:i32)  [unwired: 11 in]
              n811 = call "myRIO_BRig_RT_dataLC_Wrong_Trial.vi"() -> ("output_Wrong_Trial"=w1556:i32)  [unwired: 11 in]
              n812 = call "myRIO_BRig_RT_dataLC_Reward_Block.vi"() -> ("output_Reward_Block"=w1572:i32)  [unwired: 11 in]
              n813 = call "myRIO_BRig_RT_dataLC_Reward_OnOff.vi"() -> ("output_Reward_OnOff"=w1570:i32)  [unwired: 11 in]
              n814 = call "myRIO_BRig_RT_dataLC_Reward_Probability.vi"() -> ("output_Reward_Probability"=w1566:i32)  [unwired: 11 in]
              n815 = call "myRIO_BRig_RT_dataLC_Reward_Tdelay.vi"() -> ("output_Reward_Tdelay"=w1564:i32)  [unwired: 11 in]
              n816 = call "myRIO_BRig_RT_dataLC_Reward_Trial.vi"() -> ("output_Reward_Trial"=w1562:i32)  [unwired: 11 in]
              n817 = local read "LC_Wrong_OnOff"() -> (w1554:bool)
              n818 = local read "LC_Wrong_Probability"() -> (w1551:u16)
              n819 = local read "LC_Wrong_Block"() -> (w1553:u16)
              n820 = local read "LC_Wrong_Tdelay"() -> (w1550:u16)
              n821 = local read "LC_Wrong_Trial"() -> (w1549:u16)
              n822 = local read "LC_Reward_Probability"() -> (w1565:u16)
              n823 = local read "LC_Reward_Block"() -> (w1571:u16)
              n824 = local read "LC_Reward_Tdelay"() -> (w1563:u16)
              n825 = local read "LC_Reward_OnOff"() -> (w1569:bool)
              n826 = local read "LC_Reward_Trial"() -> (w1561:u16)
              n827 = Boolean To (0,1)(Boolean=w1554) -> (0, 1=w1555:i16)
              n828 = Boolean To (0,1)(Boolean=w1569) -> (0, 1=w1568:i16)
              n829 = To Unsigned Word Integer(number=w1555) -> (unsigned 16bit integer=w1552:u16)
              n830 = To Unsigned Word Integer(number=w1568) -> (unsigned 16bit integer=w1567:u16)
              n831 = Replace Array Subset(array=w1573, new element #1=w1571, index #1=w1572, new element #2=w1567, index #2=w1570, new element #3=w1565, index #3=w1566, new element #4=w1563, index #4=w1564, new element #5=w1561, index #5=w1562, new element #6=w1553, index #6=w1560, new element #7=w1552, index #7=w1559, new element #8=w1551, index #8=w1558, new element #9=w1550, index #9=w1557, new element #10=w1549, index #10=w1556) -> (w1574:u16[])
            }
            frame "setSettings_Audio" {
              # "amp_L"
              # "amp_R"
              # "freq_L"
              # "freq_R"
              n832 = call "myRIO_BRig_RT_dataExp_Audio_amp__L.vi"() -> ("output_Audio_amp__L"=w1599:i32)  [unwired: 11 in]
              n833 = call "myRIO_BRig_RT_dataExp_Audio_amp__R.vi"() -> ("output_Audio_amp__R"=w1598:i32)  [unwired: 11 in]
              n834 = call "myRIO_BRig_RT_dataExp_Audio_freq__L.vi"() -> ("output_Audio_freq__L"=w1597:i32)  [unwired: 11 in]
              n835 = call "myRIO_BRig_RT_dataExp_Audio_freq__R.vi"() -> ("output_Audio_freq__R"=w1596:i32)  [unwired: 11 in]
              n836 = Index Array(array=w1595, index #1=w1599, index #2=w1598, index #3=w1597, index #4=w1596) -> (element #1=w1594:u16, element #2=w1593:u16, element #3=w1586:u16, element #4=w1584:u16)
              n837 = To Unsigned Byte Integer(number=w1586) -> (unsigned 8bit integer=w1585:u8)
              n838 = To Unsigned Byte Integer(number=w1584) -> (unsigned 8bit integer=w1583:u8)
            }
            frame "setSettings_Laser" {
              (unwired) u32 0 ("tDelay_laser_rew")
              # "Wrong tDelay"
              # "Reward tDelay"
              n839 = call "myRIO_BRig_RT_dataLC_Reward_Tdelay.vi"() -> ("output_Reward_Tdelay"=w1626:i32)  [unwired: 11 in]
              n840 = call "myRIO_BRig_RT_dataLC_Wrong_Tdelay.vi"() -> ("output_Wrong_Tdelay"=w1627:i32)  [unwired: 11 in]
              n841 = Index Array(array=w1623, index #1=w1626, index #2=w1627) -> (element #1=w1625:u16, element #2=w1624:u16)
              n842 = call "myRIO_BRig_RT__calc_Tvalley.vi"("input_peakWidth"="laser_Tpeak", "input_freq"="laser_Freq") -> ("output_Tvalley"=w1633:dbl)  [unwired: 9 in]
              n843 = To Double Precision Float(number=w1625) -> (double precision float=w1620:dbl)
              n844 = To Double Precision Float(number=w1624) -> (double precision float=w1617:dbl)
              n845 = Multiply(x="f_millisec2count", y="laser_Tpeak") -> (x*y=w1642:dbl)
              n846 = Multiply(x="f_millisec2count", y=w1633) -> (x*y=w1639:dbl)
              n847 = Multiply(x="f_millisec2count", y="laser_Tshutter") -> (x*y=w1637:dbl)
              n848 = Round Toward +Infinity(x="laser_Tshutter") -> (ceil(x): smallest int >= x=w1628:dbl)
              n849 = Multiply(x="f_millisec2count", y=w1620) -> (x*y=w1621:dbl)
              n850 = Multiply(x="f_millisec2count", y=w1617) -> (x*y=w1618:dbl)
              n851 = To Unsigned Word Integer(number="f_millisec2count") -> (unsigned 16bit integer=w1608:u16)
              n852 = Round Toward +Infinity(x=w1642) -> (ceil(x): smallest int >= x=w1643:dbl)
              n853 = Round Toward +Infinity(x=w1639) -> (ceil(x): smallest int >= x=w1640:dbl)
              n854 = Round Toward +Infinity(x=w1637) -> (ceil(x): smallest int >= x=w1632:dbl)
              n855 = Round Toward +Infinity(x=w1621) -> (ceil(x): smallest int >= x=w1622:dbl)
              n856 = Round Toward +Infinity(x=w1618) -> (ceil(x): smallest int >= x=w1619:dbl)
              n857 = To Unsigned Long Integer(number=w1643) -> (unsigned 32bit integer=w1641:u32)
              n858 = To Unsigned Long Integer(number=w1640) -> (unsigned 32bit integer=w1638:u32)
              n859 = To Unsigned Long Integer(number=w1632) -> (unsigned 32bit integer=w1636:u32)
              n860 = To Unsigned Word Integer(number=w1628) -> (unsigned 16bit integer=w1631:u16)
              n861 = To Unsigned Long Integer(number=w1622) -> (unsigned 32bit integer=w1616:u32)
              n862 = To Unsigned Long Integer(number=w1619) -> (unsigned 32bit integer=w1615:u32)
              n863 = Add(x="laser_duration", y=w1631) -> (x+y=w1612:u16)
              n864 = To Double Precision Float(number=w1612) -> (double precision float=w1611:dbl)
              n865 = Multiply(x=w1611, y="f_millisec2count") -> (x*y=w1613:dbl)
              n866 = call "myRIO_BRig_RT_dataCurrent_LaserPulse_duration.vi"() -> ("output_LaserPulse_duration"=w1644:i32)  [unwired: 11 in]
              n867 = Round Toward +Infinity(x=w1613) -> (ceil(x): smallest int >= x=w1614:dbl)
              n868 = To Unsigned Long Integer(number=w1614) -> (unsigned 32bit integer=w1610:u32)
              n869 = xnode "Read/Write Control"("FPGA VI Reference In"=w1646, "error in"=w1647, "laser_Npeak"=w1641, "laser_Nvalley"=w1638, "laser_Nshutter"=w1636, "laser_selRew_Ndelay"=w1616, "laser_selWro_NDelay"=w1615, "laser_selRew_Ntotal"=w1610, "laser_selWro_Ntotal"=w1610, "k1__counter_per_ms"=w1608) -> ("error out"=→"error out":errorcluster)  [unwired: 1 out]
              n870 = Replace Array Subset(array=w1623, new element=w1612, index=w1644) -> (w1645:u16[])
            }
            frame "initBlock" {
              n871 = call "myRIO_Brig_RT__Case_Exp_State_initBlock.vi"("input_spout"=w1691, "input_dataExp"=w1689, "input_dataCurrent"=w1690) -> ("output_spout"=w1669:enum16{"Left", "Right"}, "output_state"=w1692:T2, "output_dataExp"=w1688:u16[], "output_dataCurrent"=w1674:u16[], "output_TpB_target"=→"TpB_target":u16)  [unwired: 4 in]
              "cSpout" <- w1669
              n872 = call "myRIO_BRig_RT_dataCurrent_iBlock.vi"() -> ("output_iBlock"=w1673:i32)  [unwired: 11 in]
              n873 = Index Array(array=w1674, index=w1673) -> (element=w1667:u16)
              "iBlock" <- w1667
            }
            frame "initBlock2" {
              n874 = local write "nRewards_cur"(u16 0 ("nRewards_cur")) -> ()
              n875 = call "myRIO_BRig_RT__Case_Exp_State_initBlock2.vi"("input_spout"=w1700, "input_dataBlock"=w1701, "input_dataCurrent"=w1699) -> ("idxDataBlock"=w1696:i32, "output_dataBlock"=w1698:u16[][])  [unwired: 7 in]
            }
            frame "initTrial" {
              n876 = call "myRIO_Brig_RT__Case_Exp_State_initTrial.vi"("input_spout"=w1719, "input_dataExp"=w1735, "input_dataCurrent"=w1736) -> ("output_state"=w1737:T2, "output_dataExp"=w1734:u16[], "output_dataCurrent"=w1724:u16[])  [unwired: 6 in]
              n877 = call "myRIO_BRig_RT_dataCurrent_iTrial.vi"() -> ("output_iTrial"=w1723:i32)  [unwired: 11 in]
              n878 = call "myRIO_BRig_RT_dataCurrent_SolenoidReward.vi"() -> ("output_SolenoidReward"=w1718:i32)  [unwired: 11 in]
              n879 = Index Array(array=w1724, index #1=w1723, index #2=w1718) -> (element #1=w1714:u16, element #2=w1717:u16)
              "iTrial" <- w1714
              n880 = Not Equal To 0?(x=w1717) -> (x != 0?=→"SolenoidReward":bool)
            }
            frame "initTrial2" {
              # "trialUntilReward"
              n881 = call "myRIO_BRig_RT__Case_Exp_subState_LC__initTrial.vi"("input_dataTrial"=w1744, "input_spout"=w1753, "input_dataCurrent"=w1742, "input_dataLC"=w1741) -> ("output_LC_Wrong"=w1754:bool, "output_LC_led_Wrong"=w1746:bool, "output_LC_Reward"=w1755:bool, "output_LC_led_Reward"=w1745:bool, "output_dataTrial"=w1743:u16[][])  [unwired: 2 in]
              n882 = Equal?(x=w1753, y=enum16{"Left", "Right"}."Right") -> (x = y?=w1751:bool)
              n883 = call "myRIO_BRig_RT_dataExp_ItrialUntilReward.vi"() -> ("output_I_trialUntilReward"=w1749:i32)  [unwired: 11 in]
              n884 = Index Array(array=w1750, index=w1749) -> (element=w1748:u16)
              n885 = Not Equal To 0?(x=w1748) -> (x != 0?=w1747:bool)
              n886 = xnode "Read/Write Control"("FPGA VI Reference In"=w1768, "error in"=w1767, "SelectionState"=FALSE, "laserResponse_reward"=w1755, "laserResponse_wrong"=w1754, "laserResponse_reward_LED"=w1745, "laserResponse_wrong_LED"=w1746, "Left(F)_or_Right(T)"=w1751, "ignoreWrong"=w1747) -> ("error out"=→"error_initTrial":errorcluster)  [unwired: 1 out]
            }
            frame "initTrial3" {
              n887 = call "myRIO_BRig_RT__Case_Exp_State_initTrial_dataTrial.vi"("input_spout"=w1783, "input_dataCurrent"=w1784, "input_dataExp"=w1782, "input_dataTrial"=w1786) -> ("output_dataTrial"=w1785:u16[][], "output_laserPower"=w1779:u16)  [unwired: 6 in]
              n888 = To Double Precision Float(number=w1779) -> (double precision float=w1781:dbl)
              n889 = Divide(x=w1781, y=100.0 ("x")) -> (x/y=w1775:dbl)
              "output_PortA" <- w1775
              n890 = call "myRIO__convert__Voltage_to_FPGAvalue.vi"("input_voltage"=w1775) -> ("output_PortC"=w1774:i16)  [unwired: 9 in, 1 out]
              n891 = xnode "Read/Write Control"("FPGA VI Reference In"=w1778, "error in"=w1777, "AnaOut_0"=w1774) -> ("error out"=→"error out 4":errorcluster)  [unwired: 1 out]
            }
            frame "initTrial4" {
              n892 = call "myRIO_BRig_RT_dataCurrent_idxDataTrial.vi"() -> ("output_idxDataTrial"=w1811:i32)  [unwired: 11 in]
              n893 = call "myRIO_BRig_RT_dataTrial_activeRecording.vi"() -> ("output_activeRecording"=w1808:i32)  [unwired: 11 in]
              n894 = Index Array(array=w1813, index=w1811) -> (element=w1810:u16)
              n895 = Boolean To (0,1)(Boolean="Recording") -> (0, 1=w1807:i16)
              n896 = To Long Integer(number=w1810) -> (32bit integer=w1809:i32)
              n897 = To Unsigned Word Integer(number=w1807) -> (unsigned 16bit integer=w1806:u16)
              n898 = Replace Array Subset(array=w1812, new element=w1806, index (row)=w1809, index (col)=w1808) -> (w1805:u16[][])
            }
            frame "initTrial_LC_ENL1" {
              n899 = call "myRIO_BRig_RT__Case_Exp_State_initTrial_LC_ENL1__v2.vi"("input_dataTrial"=w1837, "input_spout"=w1842, "input_dataBlock"=w1835, "input_dataLC"=w1843, "input_dataCurrent"=w1839) -> ("output_LC__ENL1"=w1841:bool, "output_LC_led__ENL1"=w1840:bool, "output_dataTrial"=w1836:u16[][], "output_dataCurrent"=w1838:u16[])  [unwired: 3 in]
            }
            frame "initTrial_LC_Cue1" {
              w1858 = TRUE ("Recording")
              n900 = call "myRIO_BRig_RT__Case_Exp_State_initTrial_LC_Cue1__v2.vi"("input_dataTrial"=w1865, "input_spout"=w1868, "input_dataBlock"=w1863, "input_dataLC"=w1869, "input_dataCurrent"=w1867) -> ("output_LC__Cue1"=w1861:bool, "output_LC_led__Cue1"=w1862:bool, "output_dataTrial"=w1864:u16[][], "output_dataCurrent"=w1866:u16[])  [unwired: 3 in]
            }
            frame "initTrial_LC_Sel" {
              n901 = call "myRIO_BRig_RT__Case_Exp_State_initTrial_LC_Sel__v2.vi"("input_dataTrial"=w1894, "input_spout"=w1897, "input_dataBlock"=w1892, "input_dataLC"=w1898, "input_dataCurrent"=w1896) -> ("output_LC__Sel"=w1884:bool, "output_LC_led__Sel"=w1885:bool, "output_dataTrial"=w1893:u16[][], "output_dataCurrent"=w1895:u16[])  [unwired: 3 in]
              n902 = local read "Recording"() -> (w1889:bool)
            }
            frame "ENL1_pre" {
              # "ENL1_n"
              # "Tcycle"
              # "counter"
              n903 = call "myRIO_BRig_RT_dataCurrent_Tcycle_generic.vi"() -> ("output_Tcycle_generic"=w1944:i32)  [unwired: 11 in]
              n904 = call "myRIO_BRig_RT_dataCurrent_count_generic.vi"() -> ("output_count_generic"=w1946:i32)  [unwired: 11 in]
              n905 = call "myRIO_BRig_RT_dataCurrent_ENL.vi"() -> ("output_ENL"=w1943:i32)  [unwired: 11 in]
              n906 = call "myRIO_BRig_RT_dataCurrent_ENL1_n.vi"() -> ("output_ENL1_n"=w1917:i32)  [unwired: 11 in]
              n907 = Index Array(array=w1937, index #1=w1943, index #2=w1917) -> (element #1=w1942:u16, element #2=w1916:u16)
              n908 = Increment(x=w1916) -> (x+1=w1915:u16)
              n909 = Replace Array Subset(array=w1937, new element #1=u16 0 ("new element/subarray"), index #1=w1946, new element #2=w1942, index #2=w1944, new element #3=w1915, index #3=w1917) -> (w1941:u16[])
              n910 = Select(t=myRIO_BRig_RT__Case_Exp_stateList."ENL1Penalty_pre" ("Enum"), s=w1925, f=myRIO_BRig_RT__Case_Exp_stateList."ENL1" ("Enum")) -> (s? t:f=w1922:T2)
            }
            frame "ENL1" {
              n911 = call "myRIO_BRig_RT__Case_Exp_State_ENL1__v2.vi"("input_LC"=w1953, "I_lick"=w1956, "input_LC_led"=w1954, "input_state"=w1962, "input_dataCurrent"=w1961) -> ("output_trigger_laser_led"=w1952:bool, "output_state"=w1959:T2, "output_dataCurrent"=w1960:u16[], "output_trigger_laser"=w1951:bool)  [unwired: 3 in]
            }
            frame "ENL1Penalty_pre" {
              # "Tcycle"
              # "counter"
              n912 = call "myRIO_BRig_RT_dataCurrent_Tcycle_generic.vi"() -> ("output_Tcycle_generic"=w2002:i32)  [unwired: 11 in]
              n913 = call "myRIO_BRig_RT_dataCurrent_count_generic.vi"() -> ("output_count_generic"=w2004:i32)  [unwired: 11 in]
              n914 = call "myRIO_BRig_RT_dataExp_ENL_penalty.vi"() -> ("output_ENL_penalty"=w1997:i32)  [unwired: 11 in]
              n915 = Index Array(array=w1998, index=w1997) -> (element=w2001:u16)
              n916 = Replace Array Subset(array=w1999, new element #1=u16 0 ("new element/subarray"), index #1=w2004, new element #2=w2001, index #2=w2002) -> (w2000:u16[])
            }
            frame "ENL1Penalty" {
              n917 = call "myRIO_BRig_RT__Case_Exp_State_ENL1Penalty.vi"("input_state"=w2027, "input_dataCurrent"=w2031) -> ("output_state"=w2028:T2, "output_dataCurrent"=w2030:u16[])  [unwired: 8 in]
            }
            frame "ENL2_pre" {
            }
            frame "ENL2" {
            }
            frame "ENL2Penalty_pre" {
            }
            frame "ENL2Penalty" {
            }
            frame "Cue1_pre" {
              # "Cue1_n"
              # "Tcycle_Cue1"
              # "0 = L, 1 = R, 2 = both"
              # "sp_R"
              # "sp_L"
              # "Tcycle"
              # "counter"
              n918 = Equal?(x=w2142, y=enum16{"Left", "Right"}."Left") -> (x = y?=w2141:bool)
              n919 = call "myRIO_BRig_RT_dataExp_Audio_sp__L.vi"() -> ("output_Audio_sp__L"=w2140:i32)  [unwired: 11 in]
              n920 = call "myRIO_BRig_RT_dataExp_Audio_sp__R.vi"() -> ("output_Audio_sp__R"=w2139:i32)  [unwired: 11 in]
              n921 = call "myRIO_BRig_RT_dataCurrent_Tcycle_generic.vi"() -> ("output_Tcycle_generic"=w2152:i32)  [unwired: 11 in]
              n922 = call "myRIO_BRig_RT_dataCurrent_count_generic.vi"() -> ("output_count_generic"=w2154:i32)  [unwired: 11 in]
              n923 = Select(t=w2140, s=w2141, f=w2139) -> (s? t:f=w2138:i32)
              n924 = call "myRIO_BRig_RT_dataCurrent_Cue1_n.vi"() -> ("output_Cue1_n"=w2116:i32)  [unwired: 11 in]
              n925 = call "myRIO_BRig_RT_dataCurrent_Tcycle_cue.vi"() -> ("output_Tcycle_cue"=w2125:i32)  [unwired: 11 in]
              n926 = Index Array(array=w2144, index=w2138) -> (element=w2136:u16)
              n927 = Index Array(array=w2126, index #1=w2125, index #2=w2116) -> (element #1=w2127:u16, element #2=w2118:u16)
              n928 = Increment(x=w2118) -> (x+1=w2117:u16)
              n929 = Not Equal To 0?(x=w2136) -> (x != 0?=w2134:bool)
              n930 = Not Equal?(x=w2136, y=u16 1) -> (x != y?=w2135:bool)
              n931 = Replace Array Subset(array=w2126, new element #1=u16 0 ("new element/subarray"), index #1=w2154, new element #2=w2127, index #2=w2152, new element #3=w2117, index #3=w2116) -> (w2151:u16[])
              n932 = Select(t=myRIO_BRig_RT__Case_Exp_stateList."Cue1Penalty_pre" ("Enum"), s=w2122, f=myRIO_BRig_RT__Case_Exp_stateList."Cue1" ("Enum")) -> (s? t:f=w2123:T2)
            }
            frame "Cue1" {
              n933 = call "myRIO_BRig_RT__Case_Exp_State_Cue1__v2.vi"("input_LC"=w2163, "I_lick"=w2166, "input_LC_led"=w2164, "input_state"=w2168, "input_dataCurrent"=w2186) -> ("output_trigger_laser_led"=w2161:bool, "output_state"=w2167:T2, "output_dataCurrent"=w2185:u16[], "output_trigger_laser"=w2162:bool)  [unwired: 3 in]
              n934 = Equal?(x=myRIO_BRig_RT__Case_Exp_stateList."Selection_pre", y=w2167) -> (x = y?=w2171:bool)
              n935 = xnode "Read/Write Control"("FPGA VI Reference In"=w2170, "error in"=w2169, "SelectionState"=w2171) -> ()  [unwired: 2 out]
            }
            frame "Cue1Penalty_pre" {
              # "Tcycle"
              # "counter"
              n936 = call "myRIO_BRig_RT_dataCurrent_Tcycle_generic.vi"() -> ("output_Tcycle_generic"=w2217:i32)  [unwired: 11 in]
              n937 = call "myRIO_BRig_RT_dataCurrent_count_generic.vi"() -> ("output_count_generic"=w2219:i32)  [unwired: 11 in]
              n938 = call "myRIO_BRig_RT_dataExp_Tcycle_CuePenalty.vi"() -> ("output_Tcycle_CuePenalty"=w2216:i32)  [unwired: 11 in]
              n939 = Index Array(array=w2211, index=w2216) -> (element=w2215:u16)
              n940 = Replace Array Subset(array=w2213, new element #1=u16 0 ("new element/subarray"), index #1=w2219, new element #2=w2215, index #2=w2217) -> (w2212:u16[])
            }
            frame "Cue1Penalty" {
              # "reset laserOccurred"
              n941 = call "myRIO_BRig_RT__Case_Exp_State_Cue1Penalty.vi"("input_state"=w2245, "input_dataCurrent"=w2246) -> ("output_state"=w2243:T2, "output_dataCurrent"=w2244:u16[])  [unwired: 8 in]
            }
            frame "Cue2_pre" {
              n942 = call "myRIO_BRig_RT__Case_Exp_subState_LC__Cue2.vi"("input_spout"=w2263, "input_dataCurrent"=w2264, "input_dataLC"=w2262) -> ()  [unwired: 6 in, 2 out]
            }
            frame "Cue2" {
            }
            frame "Cue2Penalty_pre" {
            }
            frame "Cue2Penalty" {
            }
            frame "Selection_pre" {
              # "Tcycle"
              # "counter"
              n943 = call "myRIO_BRig_RT_dataCurrent_Sel_laserTiming_start.vi"() -> ("output_Sel_laserTiming_start"=w2334:i32)  [unwired: 11 in]
              n944 = xnode "Read/Write Control"("FPGA VI Reference In"=w2344, "error in"=w2345) -> ("error out"=→"error_Selection_pre":errorcluster, "SelectReward"=w2338:bool, "SelectWrong"=w2339:bool)  [unwired: 1 out]
              n945 = call "myRIO_BRig_RT_dataExp_Tcycle_Selection.vi"() -> ("output_Tcycle_Selection"=w2364:i32)  [unwired: 11 in]
              n946 = call "myRIO_BRig_RT_dataCurrent_Tcycle_generic.vi"() -> ("output_Tcycle_generic"=w2365:i32)  [unwired: 11 in]
              n947 = call "myRIO_BRig_RT_dataCurrent_count_generic.vi"() -> ("output_count_generic"=w2367:i32)  [unwired: 11 in]
              n948 = Index Array(array=w2335, index=w2334) -> (element=w2333:u16)
              n949 = Index Array(array=w2361, index=w2364) -> (element=w2363:u16)
              n950 = Equal To 0?(x=w2333) -> (x = 0?=w2331:bool)
              n951 = Replace Array Subset(array=w2335, new element #1=u16 0 ("new element/subarray"), index #1=w2367, new element #2=w2363, index #2=w2365) -> (w2362:u16[])
              n952 = Or(x=w2338, y=w2339) -> (x .or. y?=w2329:bool)
              n953 = Not(x=w2329) -> (.not. x?=w2332:bool)
              n954 = Compound Arithmetic op=AND(w2332, w2331, w2330) -> (w2327:bool)
              n955 = And(x=w2327, y=w2328) -> (x .and. y?=w2326:bool)
              n956 = Select(t=myRIO_BRig_RT__Case_Exp_stateList."SelectReward_pre" ("Enum"), s=w2338, f=myRIO_BRig_RT__Case_Exp_stateList."SelectWrong_pre" ("Enum")) -> (s? t:f=w2343:T2)
              n957 = Select(t=w2343, s=w2329, f=myRIO_BRig_RT__Case_Exp_stateList."Selection" ("Enum")) -> (s? t:f=w2340:T2)
            }
            frame "Selection" {
              # "counter\nSelection"
              # "increment"
              # "get Tcycle"
              # "get count"
              n958 = call "myRIO_BRig_RT_dataCurrent_Tcycle_generic.vi"() -> ("output_Tcycle_generic"=w2401:i32)  [unwired: 11 in]
              n959 = call "myRIO_BRig_RT_dataCurrent_count_generic.vi"() -> ("output_count_generic"=w2397:i32)  [unwired: 11 in]
              n960 = call "myRIO_BRig_RT_dataCurrent_Sel_laserTiming_start.vi"() -> ("output_Sel_laserTiming_start"=w2389:i32)  [unwired: 11 in]
              n961 = call "myRIO_BRig_RT_dataCurrent_Sel_laserTiming_end.vi"() -> ("output_Sel_laserTiming_end"=w2388:i32)  [unwired: 11 in]
              n962 = call "myRIO_BRig_RT__increment_u16.vi"() -> ("output_increment__u16"=w2375:u16)  [unwired: 11 in]
              n963 = xnode "Read/Write Control"("FPGA VI Reference In"=w2408, "error in"=w2407) -> ("error out"=→"error_Selection":errorcluster, "SelectReward"=w2404:bool, "SelectWrong"=w2405:bool)  [unwired: 1 out]
              n964 = call "myRIO_BRig_RT_dataCurrent_Sel_laserTriggered.vi"() -> ("output_Sel_laserTriggered"=w2376:i32)  [unwired: 11 in]
              n965 = Index Array(array=w2402, index #1=w2401, index #2=w2397, index #3=w2389, index #4=w2388, index #5=w2376) -> (element #1=w2396:u16, element #2=w2374:u16, element #3=w2373:u16, element #4=w2379:u16, element #5=w2370:u16)
              n966 = Increment(x=w2370) -> (x+1=w2371:u16)
              n967 = Equal?(x=w2374, y=w2373) -> (x = y?=w2372:bool)
              n968 = Add(x=w2374, y=w2375) -> (x+y=w2380:u16)
              n969 = Greater Or Equal?(x=w2380, y=w2373) -> (x >= y?=w2377:bool)
              n970 = Less Or Equal?(x=w2380, y=w2379) -> (x <= y?=w2378:bool)
              n971 = Greater?(x=w2396, y=w2380) -> (0:w2382:bool)
              n972 = Select(t=w2371, s=w2372, f=w2370) -> (s? t:f=w2369:u16)
              n973 = Select(t=myRIO_BRig_RT__Case_Exp_stateList."SelectReward_pre" ("Enum"), s=w2404, f=myRIO_BRig_RT__Case_Exp_stateList."SelectWrong_pre" ("Enum")) -> (s? t:f=w2403:T2)
              n974 = Or(x=w2404, y=w2405) -> (x .or. y?=w2383:bool)
              n975 = Not(x=w2383) -> (.not. x?=w2384:bool)
              n976 = Select(t=w2400, s=w2382, f=myRIO_BRig_RT__Case_Exp_stateList."SelectTimeout_pre" ("Enum")) -> (s? t:f=w2391:T2)
              n977 = Compound Arithmetic op=AND(w2382, w2384, w2377, w2378, w2381) -> (w2386:bool)
              n978 = Select(t=w2380, s=w2382, f=w2396) -> (s? t:f=w2394:u16)
              n979 = Select(t=w2403, s=w2383, f=w2391) -> (s? t:f=w2406:T2)
              n980 = And(x=w2386, y=w2385) -> (x .and. y?=w2387:bool)
              n981 = call "myRIO_BRig_RT_dataCurrent_count_selection.vi"() -> ("output_count_generic"=w2395:i32)  [unwired: 11 in]
              n982 = Replace Array Subset(array=w2402, new element #1=w2394, index #1=w2397, new element #2=w2394, index #2=w2395, new element #3=w2369, index #3=w2376) -> (w2399:u16[])
            }
            frame "SelectReward_pre" {
              # "iState"
              # "Tcycle\nReward"
              # "nRewTrials"
              # "Tcycle\nGeneric"
              # "counter"
              n983 = call "myRIO_BRig_RT_dataCurrent_nRewTrials.vi"() -> ("output_nRewTrials"=w2440:i32)  [unwired: 11 in]
              n984 = Equal?(x=w2449, y=enum16{"Left", "Right"}."Left") -> (x = y?=w2450:bool)
              n985 = Index Array(array=w2441, index=w2440) -> (element=w2439:u16)
              n986 = call "myRIO_BRig_RT_dataExp_Tcycle_Reward__L.vi"() -> ("output_Tcycle_Reward__L"=w2453:i32)  [unwired: 11 in]
              n987 = call "myRIO_BRig_RT_dataExp_Tcycle_Reward__R.vi"() -> ("output_Tcycle_Reward__R"=w2454:i32)  [unwired: 11 in]
              n988 = Increment(x=w2439) -> (x+1=w2438:u16)
              n989 = Select(t=w2453, s=w2450, f=w2454) -> (s? t:f=w2452:i32)
              n990 = call "myRIO_BRig_RT__Case_Exp_subState_LC__Reward.vi"("input_spout"=w2449, "input_dataCurrent"=w2441, "input_dataLC"=w2448) -> ()  [unwired: 6 in, 2 out]
              n991 = call "myRIO_BRig_RT_dataCurrent_count_generic.vi"() -> ("output_count_generic"=w2443:i32)  [unwired: 11 in]
              n992 = call "myRIO_BRig_RT_dataCurrent_Tcycle_generic.vi"() -> ("output_Tcycle_generic"=w2444:i32)  [unwired: 11 in]
              n993 = Index Array(array=w2455, index=w2452) -> (element=w2445:u16)
              n994 = call "myRIO_BRig_RT_dataCurrent_iState.vi"() -> ("output_iState"=w2433:i32)  [unwired: 11 in]
              n995 = Replace Array Subset(array=w2441, new element #1=w2438, index #1=w2440, new element #2=u16 0 ("new element/subarray"), index #2=w2443, new element #3=w2445, index #3=w2444, new element #4=u16 1 ("new element/subarray"), index #4=w2433) -> (w2456:u16[])
            }
            frame "SelectReward" {
              n996 = call "myRIO_BRig_RT__Case_Exp_State_Reward.vi"("input_dataCurrent"=w2477, "input_state"=w2474, "input_spout"=w2472) -> ("output_dataCurrent"=w2476:u16[], "output_state"=w2475:T2, "output__L"=w2470:bool, "output__R"=w2471:bool)  [unwired: 9 in]
            }
            frame "SelectRewardPost_pre" {
              # "nRewards"
              # "nRewTrials"
              # "Tcycle"
              # "counter"
              n997 = call "myRIO_BRig_RT_dataBlock_nRewards__L.vi"() -> ("output_nRewards__L"=w2493:i32)  [unwired: 11 in]
              n998 = call "myRIO_BRig_RT_dataBlock_nRewards__R.vi"() -> ("output_nRewards__R"=w2492:i32)  [unwired: 11 in]
              n999 = call "myRIO_BRig_RT_dataCurrent_Tcycle_generic.vi"() -> ("output_Tcycle_generic"=w2512:i32)  [unwired: 11 in]
              n1000 = call "myRIO_BRig_RT_dataCurrent_count_generic.vi"() -> ("output_count_generic"=w2514:i32)  [unwired: 11 in]
              n1001 = case shown="\"Left\", Default" w2486 {
                tunnel: w2498 -> [w2519 w2523]
                tunnel: [w2518 w2523] -> w2497
                tunnel: [w2520 w2521] -> w2496
                tunnel: w2495 -> [w2520 w2522]
                frame "Left", Default {
                  n1002 = Increment(x=w2519) -> (x+1=w2518:u16)
                }
                frame "Right" {
                  n1003 = Increment(x=w2522) -> (x+1=w2521:u16)
                }
              }
              "nRewards_Left" <- w2497
              "nRewards_Right" <- w2496
              n1004 = Equal?(x=w2486, y=enum16{"Left", "Right"}."Left") -> (x = y?=w2485:bool)
              n1005 = Select(t=w2493, s=w2485, f=w2492) -> (s? t:f=w2491:i32)
              n1006 = call "myRIO_BRig_RT_dataExp_Tcycle_RewardPost.vi"() -> ("output_Tcycle_RewardPost"=w2508:i32)  [unwired: 11 in]
              n1007 = call "myRIO_BRig_RT_dataCurrent_nRewTrials.vi"() -> ("output_nRewTrials"=w2494:i32)  [unwired: 11 in]
              n1008 = Index Array(array=w2509, index=w2508) -> (element=w2511:u16)
              n1009 = Index Array(array=w2488, index=w2494) -> (element=w2483:u16)
              n1010 = Replace Array Subset(array=w2488, new element #1=u16 0 ("new element/subarray"), index #1=w2514, new element #2=w2511, index #2=w2512) -> (w2510:u16[])
              n1011 = Replace Array Subset(array=w2490, new element=w2483, index (row)=w2484, index (col)=w2491) -> (w2489:u16[][])
              n1012 = local write "nRewards_cur"(w2483) -> ()
            }
            frame "SelectRewardPost" {
              n1013 = call "myRIO_BRig_RT__Case_Exp_State_RewardPost.vi"("input_state"=w2538, "input_dataCurrent"=w2541) -> ("output_state"=w2539:T2, "output_dataCurrent"=w2540:u16[])  [unwired: 8 in]
            }
            frame "SelectWrong_pre" {
              # "iState"
              # "Tcycle"
              # "counter"
              n1014 = call "myRIO_BRig_RT_dataCurrent_Tcycle_generic.vi"() -> ("output_Tcycle_generic"=w2566:i32)  [unwired: 11 in]
              n1015 = call "myRIO_BRig_RT_dataCurrent_count_generic.vi"() -> ("output_count_generic"=w2568:i32)  [unwired: 11 in]
              n1016 = call "myRIO_BRig_RT_dataExp_Tcycle_Wrong.vi"() -> ("output_Tcycle_Wrong"=w2564:i32)  [unwired: 11 in]
              n1017 = call "myRIO_BRig_RT__Case_Exp_subState_LC__Wrong.vi"("input_spout"=w2560, "input_dataCurrent"=w2561, "input_dataLC"=w2558) -> ()  [unwired: 6 in, 2 out]
              n1018 = Index Array(array=w2562, index=w2564) -> (element=w2565:u16)
              n1019 = call "myRIO_BRig_RT_dataCurrent_iState.vi"() -> ("output_iState"=w2552:i32)  [unwired: 11 in]
              n1020 = Replace Array Subset(array=w2561, new element #1=u16 0 ("new element/subarray"), index #1=w2568, new element #2=w2565, index #2=w2566, new element #3=u16 2 ("new element/subarray"), index #3=w2552) -> (w2563:u16[])
            }
            frame "SelectWrong" {
              n1021 = call "myRIO_BRig_RT__Case_Exp_State_Wrong.vi"("input_state"=w2582, "input_dataCurrent"=w2591) -> ("output_state"=w2579:T2, "output_dataCurrent"=w2590:u16[])  [unwired: 8 in]
              n1022 = Not Equal?(x=w2582, y=w2579) -> (x != y?=w2581:bool)
              n1023 = Select(t=myRIO_BRig_RT__Case_Exp_stateList."SelectWrong_post" ("Enum"), s=w2581, f=w2579) -> (s? t:f=w2578:T2)
            }
            frame "SelectWrong_post" {
            }
            frame "SelectTimeout_pre" {
              # "iState"
              # "Tcycle"
              # "counter"
              n1024 = xnode "Read/Write Control"("FPGA VI Reference In"=w2618, "error in"=w2617, "SelectionState"=FALSE) -> ("error out"=→"error out 3":errorcluster)  [unwired: 1 out]
              n1025 = call "myRIO_BRig_RT_dataCurrent_Tcycle_generic.vi"() -> ("output_Tcycle_generic"=w2640:i32)  [unwired: 11 in]
              n1026 = call "myRIO_BRig_RT_dataCurrent_count_generic.vi"() -> ("output_count_generic"=w2638:i32)  [unwired: 11 in]
              n1027 = call "myRIO_BRig_RT_dataExp_Tcycle_Timeout.vi"() -> ("output_Tcycle_Timeout"=w2642:i32)  [unwired: 11 in]
              n1028 = call "myRIO_BRig_RT__Case_Exp_subState_LC__Timeout.vi"("input_spout"=w2633, "input_dataCurrent"=w2634, "input_dataLC"=w2632) -> ()  [unwired: 6 in, 2 out]
              n1029 = Index Array(array=w2636, index=w2642) -> (element=w2641:u16)
              n1030 = call "myRIO_BRig_RT_dataCurrent_iState.vi"() -> ("output_iState"=w2626:i32)  [unwired: 11 in]
              n1031 = Replace Array Subset(array=w2634, new element #1=u16 0 ("new element/subarray"), index #1=w2638, new element #2=w2641, index #2=w2640, new element #3=u16 3 ("new element/subarray"), index #3=w2626) -> (w2637:u16[])
            }
            frame "SelectTimeout" {
              n1032 = call "myRIO_BRig_RT__Case_Exp_State_Timeout.vi"("input_dataLC"=w2661, "input_state"=w2652, "input_dataCurrent"=w2666) -> ("output_state"=w2653:T2, "output_dataCurrent"=w2665:u16[])  [unwired: 6 in, 1 out]
              n1033 = Not Equal?(x=w2652, y=w2653) -> (x != y?=w2656:bool)
              n1034 = Select(t=myRIO_BRig_RT__Case_Exp_stateList."SelectTimeout_post" ("Enum"), s=w2656, f=w2653) -> (s? t:f=w2654:T2)
            }
            frame "SelectTimeout_post" {
            }
            frame "endTrial1" {
              # "Update dataBlock"
              n1035 = call "myRIO_BRig_RT__Case_Exp_State_endTrial1.vi"("input_spout"=w2699, "input_dataBlock"=w2698, "input_dataCurrent"=w2696) -> ("output_dataBlock"=w2697:u16[][], "output_dataCurrent"=w2695:u16[])  [unwired: 7 in]
            }
            frame "endTrial2" {
              # "update dataTrial"
              n1036 = call "myRIO_BRig_RT__Case_Exp_State_endTrial2.vi"("input_spout"=w2718, "input_dataTrial"=w2722, "input_dataCurrent"=w2720) -> ("output_dataTrial"=w2721:u16[][], "output_dataCurrent"=w2719:u16[])  [unwired: 7 in]
            }
            frame "endTrial3" {
              w2748 = myRIO_BRig_RT__Case_Exp_stateList."endBlock" ("Enum")
              # "nRewTrials"
              # "iTrial"
              # "I_blockUntilReward"
              # "TPB"
              # "end block?"
              n1037 = local read "STOP_endTrial"() -> (w2746:bool)
              n1038 = local read "STOP_abort"() -> (w2745:bool)
              n1039 = xnode "Read/Write Control"("FPGA VI Reference In"=w2734, "error in"=w2733, "SelectionState"=FALSE) -> ("error out"=→"error out 2":errorcluster)  [unwired: 1 out]
              n1040 = local read "START"() -> (w2743:bool)
              n1041 = call "myRIO_BRig_RT_dataExp_IblockUntilReward.vi"() -> ("output_I_blockUntilReward"=w2755:i32)  [unwired: 11 in]
              n1042 = Index Array(array=w2739, index=w2755) -> (element=w2735:u16)
              n1043 = Not(x=w2743) -> (.not. x?=w2744:bool)
              n1044 = Not Equal To 0?(x=w2735) -> (x != 0?=w2753:bool)
              n1045 = Compound Arithmetic op=OR(w2746, w2744, w2745) -> (w2747:bool)
              n1046 = call "myRIO_BRig_RT_dataCurrent_nRewTrials.vi"() -> ("output_nRewTrials"=w2751:i32)  [unwired: 11 in]
              n1047 = call "myRIO_BRig_RT_dataCurrent_iTrial.vi"() -> ("output_iTrial"=w2752:i32)  [unwired: 11 in]
              n1048 = Select(t=w2751, s=w2753, f=w2752) -> (s? t:f=w2750:i32)
              n1049 = call "myRIO_BRig_RT_dataCurrent_TpB.vi"() -> ("output_TpB"=w2754:i32)  [unwired: 11 in]
              n1050 = Index Array(array=w2740, index #1=w2754, index #2=w2750) -> (element #1=w2741:u16, element #2=w2742:u16)
              n1051 = Less Or Equal?(x=w2741, y=w2742) -> (x <= y?=w2738:bool)
              n1052 = Select(t=w2748, s=w2738, f=myRIO_BRig_RT__Case_Exp_stateList."empty_endTrial1" ("Enum")) -> (s? t:f=w2749:T2)
              n1053 = Select(t=w2748, s=w2747, f=w2749) -> (s? t:f=w2736:T2)
            }
            frame "endBlock" {
              # "R"
              # "L"
              # "idxDataBlock"
              n1054 = Equal?(x=w2779, y=enum16{"Left", "Right"}."Left") -> (x = y?=w2778:bool)
              n1055 = call "myRIO_BRig_RT_dataCurrent_idxDataBlockL.vi"() -> ("output_idxDataBlock__L"=w2782:i32)  [unwired: 11 in]
              n1056 = call "myRIO_BRig_RT_dataCurrent_idxDataBlockR.vi"() -> ("output_idxDataBlock__R"=w2781:i32)  [unwired: 11 in]
              n1057 = Increment(x=w2773) -> (x+1=w2772:i32)
              n1058 = Select(t=w2782, s=w2778, f=w2781) -> (s? t:f=w2776:i32)
              n1059 = To Unsigned Word Integer(number=w2772) -> (unsigned 16bit integer=w2774:u16)
              n1060 = local read "START"() -> (w2802:bool)
              n1061 = local read "STOP_endBlock"() -> (w2797:bool)
              n1062 = local read "STOP_endTrial"() -> (w2800:bool)
              n1063 = local read "STOP_abort"() -> (w2799:bool)
              n1064 = Replace Array Subset(array=w2777, new element=w2774, index=w2776) -> (w2775:u16[])
              n1065 = Not(x=w2802) -> (.not. x?=w2801:bool)
              n1066 = Compound Arithmetic op=OR(w2801, w2797, w2800, w2799) -> (w2798:bool)
              n1067 = Select(t=myRIO_BRig_RT__Case_Exp_stateList."endExp" ("Enum"), s=w2798, f=myRIO_BRig_RT__Case_Exp_stateList."empty_endBlock1" ("Enum")) -> (s? t:f=w2806:T2)
            }
            frame "endExp" {
            }
            frame "commConnect" {
              n1068 = call "myRIO_BRig_RT_comm_webdav_connect.vi"("input_password"="Host Password", "input_username"="Host UserName") -> ("output_Iconnected"=w2827:bool, "output_hSession"=w2845:T6)  [unwired: 7 in, 1 out]
              "Connected To Host?" <- w2827
              n1069 = case shown="False" w2827 {
                frame False {
                  n1070 = One Button Dialog(message="Connection Failed!\nData not being saved!") -> ()  [unwired: 1 in, 1 out]
                }
                frame True {
                }
              }
            }
            frame "commUpload_pre" {
              n1071 = Select(t=myRIO_BRig_RT__Case_Exp_stateList."commUpload_dataBlock" ("Enum"), s=w2852, f=myRIO_BRig_RT__Case_Exp_stateList."endTrial3") -> (s? t:f=w2850:T2)
            }
            frame "commUpload_dataBlock" {
              n1072 = call "myRIO_BRig_RT_comm_webdav_uploadFile__data.vi"("input_fileName_prefix"=w2873, "input_fileName"="dataBlock" ("input_filename"), "input_hSession"=w2875) -> ()  [unwired: 8 in, 1 out]
            }
            frame "commUpload_dataCurrent" {
              n1073 = call "myRIO_BRig_RT_comm_webdav_uploadFile__data.vi"("input_fileName_prefix"=w2894, "input_fileName"="dataCurrent" ("input_filename"), "input_hSession"=w2896) -> ()  [unwired: 8 in, 1 out]
            }
            frame "commUpload_dataExp" {
              n1074 = call "myRIO_BRig_RT_comm_webdav_uploadFile__data.vi"("input_fileName_prefix"=w2915, "input_fileName"="dataExp" ("input_filename"), "input_hSession"=w2917) -> ()  [unwired: 8 in, 1 out]
            }
            frame "commUpload_dataLC" {
              n1075 = call "myRIO_BRig_RT_comm_webdav_uploadFile__data.vi"("input_fileName_prefix"=w2936, "input_fileName"="dataLC" ("input_filename"), "input_hSession"=w2938) -> ()  [unwired: 8 in, 1 out]
            }
            frame "commUpload_dataTrial" {
              n1076 = call "myRIO_BRig_RT_comm_webdav_uploadFile__data.vi"("input_fileName_prefix"=w2960, "input_fileName"="dataTrial" ("input_filename"), "input_hSession"=w2962) -> ()  [unwired: 8 in, 1 out]
            }
            frame "saveData_dataBlock" {
              # "idxDataBlockR"
              # "idxDataBlockL"
              n1077 = call "myRIO_BRig_RT_dataCurrent_idxDataBlockL.vi"() -> ("output_idxDataBlock__L"=w2986:i32)  [unwired: 11 in]
              n1078 = call "myRIO_BRig_RT_dataCurrent_idxDataBlockR.vi"() -> ("output_idxDataBlock__R"=w2987:i32)  [unwired: 11 in]
              n1079 = Index Array(array=w2988, index #1=w2986, index #2=w2987) -> (element #1=w2985:u16, element #2=w2984:u16)
              n1080 = Greater?(x=w2985, y=w2984) -> (0:w2983:bool)
              n1081 = Select(t=w2985, s=w2983, f=w2984) -> (s? t:f=w2981:u16)
              n1082 = Increment(x=w2981) -> (x+1=w2980:u16)
              n1083 = To Long Integer(number=w2980) -> (32bit integer=w2979:i32)
              n1084 = Array Subset(array=w2982, length (row)=w2979) -> (w2978:u16[][])  [unwired: 3 in]
              n1085 = call "myRIO_BRig_RT_comm_webdav_saveArrayToFile__2D_u16.vi"("Array"=w2978, "input_filename"="dataBlock") -> ()  [unwired: 10 in]
            }
            frame "saveData_dataCurrent" {
              n1086 = call "myRIO_BRig_RT_comm_webdav_saveArrayToFile__1D_u16.vi"("Array"=w3007, "input_filename"="dataCurrent") -> ()  [unwired: 10 in]
            }
            frame "saveData_dataExp" {
              # "runTime"
              n1087 = Get Date/Time In Seconds() -> (seconds since 1Jan1904=w3035:timestamp)
              n1088 = To Double Precision Float(number=w3035) -> (double precision float=w3034:dbl)
              n1089 = call "myRIO_BRig_RT_dataExp_runTime_seconds.vi"() -> ("output_RunTime_minutes"=w3033:i32)  [unwired: 11 in]
              n1090 = Subtract(x=w3034, y=w3032) -> (x-y=w3029:dbl)
              n1091 = To Unsigned Word Integer(number=w3029) -> (unsigned 16bit integer=w3028:u16)
              n1092 = Replace Array Subset(array=w3027, new element=w3028, index=w3033) -> (w3030:u16[])
              n1093 = call "myRIO_BRig_RT_comm_webdav_saveArrayToFile__1D_u16.vi"("Array"=w3030, "input_filename"="dataExp") -> ()  [unwired: 10 in]
            }
            frame "saveData_dataLC" {
              n1094 = call "myRIO_BRig_RT_comm_webdav_saveArrayToFile__1D_u16.vi"("Array"=w3054, "input_filename"="dataLC") -> ()  [unwired: 10 in]
            }
            frame "saveData_dataTrial" {
              # "idxTrial"
              n1095 = call "myRIO_BRig_RT_dataCurrent_idxDataTrial.vi"() -> ("output_idxDataTrial"=w3079:i32)  [unwired: 11 in]
              n1096 = Index Array(array=w3080, index=w3079) -> (element=w3076:u16)
              n1097 = Increment(x=w3076) -> (x+1=w3075:u16)
              n1098 = To Long Integer(number=w3075) -> (32bit integer=w3074:i32)
              n1099 = Array Subset(array=w3077, length (row)=w3074) -> (w3078:u16[][])  [unwired: 3 in]
              n1100 = call "myRIO_BRig_RT_comm_webdav_saveArrayToFile__2D_u16.vi"("Array"=w3078, "input_filename"="dataTrial") -> ()  [unwired: 10 in]
            }
            frame "empty_endBlock1" {
            }
            frame "empty_endBlock2" {
            }
            frame "empty_endTrial1" {
            }
            frame "empty_endTrial2" {
            }
            frame "empty_endTrial3" {
            }
            frame "empty_endTrial4" {
            }
            frame "empty_endTrial5" {
            }
          }
          n1101 = Select(t=w1076, s=w1079, f=w1077) -> (s? t:f=w1078:bool)
          n1102 = case shown="True" w1150 {
            tunnel: w1147 -> [w1171 w1179]
            tunnel: w1149 -> [_ w1175]
            tunnel: w1148 -> [_ w1174]
            tunnel: w1049 -> [_ w1173]
            tunnel: w1117 -> [_ w1172]
            tunnel: [w1171 w1178] -> w1146
            tunnel: w1145 -> [w1170 w1177]
            tunnel: [w1170 w1176] -> w1144
            frame False {
            }
            frame True {
              n1103 = call "myRIO_BRig_RT__Case_Exp__recordLick.vi"("intput_state__trialEnd"=w1172, "intput_state__trialStart"=w1173, "input_lick__R"=w1174, "input_lick__L"=w1175, "input_dataCurrent"=w1177, "input_dataLick"=w1179) -> ("output_dataCurrent"=w1176:u16[], "output_dataLick"=w1178:u16[][])  [unwired: 4 in]
            }
          }
          n1104 = Or(x=w1119, y=w1120) -> (x .or. y?=w1106:bool)
          n1105 = Or(x=w1123, y=w1103) -> (x .or. y?=w1092:bool)
          n1106 = Or(x=w1102, y=w1124) -> (x .or. y?=w1118:bool)
          n1107 = Or(x=w1122, y=w1121) -> (x .or. y?=w1107:bool)
          n1108 = Or(x=w1151, y="STOP_abort") -> (x .or. y?=w1153:bool)
          n1109 = Or(x=w1082, y=w1083) -> (x .or. y?=w1080:bool)
          n1110 = Or(x=w1084, y=w1083) -> (x .or. y?=w1081:bool)
          n1111 = Select(t=w1065, s=w1066, f=w1064) -> (s? t:f=w1048:u16)
          n1112 = Select(t=w1067, s=w1069, f=w1068) -> (s? t:f=w1047:u16)
          n1113 = Select(t=u16 0, s=w1072, f=w1071) -> (s? t:f=w1056:u16)
          n1114 = xnode "Read/Write Control"("FPGA VI Reference In"=w1094, "error in"=w1093, "A1_SR"=w1107, "A3_SL"=w1106, "A6_Act"=w1078, "audioTrigger_L"=w1092, "audioAmp_L"=w1133, "audioFreq_L_kHz"=w1101, "audioTrigger_R"=w1118, "audioAmp_R"=w1134, "audioFreq_R_kHz"=w1135, "laserledMTrig"=w1080, "laserMTrig"=w1081) -> ("FPGA VI Reference Out"=w1143:refnum<k20>, "error out"=w1142:errorcluster, "AnaIn_0"=w1055:i16, "AnaIn_1"=w1054:i16)
          n1115 = local write "tempAI0"(w1055) -> ()
          n1116 = call "myRIO_BRig_RT_dataAnalog_enterData__PortC.vi"("input_iState"=w1049, "input_AI0"=w1055, "input_iEvent"=w1056, "input_AI1"=w1054, "input_iTrial"=w1048, "input_iBlock"=w1047, "input_index"=w1057, "input_dataAnalog"=w1075) -> ("output_dataAnalog"=w1074:u16[][])  [unwired: 3 in]
          n1117 = call "myRIO_BRig_RT_TCP__v2.vi"("input_hTCP"=w1062, "input_AI1"=w1054, "input_AI0"=w1055, "input_I_connected_TCP"=w1058, "input_iBlock"=w1047, "input_spout"=w1046, "input_iTrial"=w1048, "input_error"=w1060, "input_iState"=w1049) -> ("output_hTCP"=w1061:refnum<k5>, "output_error"=w1059:errorcluster)  [unwired: 5 in]
          n1118 = node-c288() -> ()  [unwired: 1 in, 1 out]
          n1119 = Increment(x=w1056) -> (x+1=w1063:u16)
          n1120 = Increment(x=w1057) -> (x+1=w1073:i32)
          "cState" <- w1049
        }
        n1121 = node-c288(w996) -> ()  [unwired: 1 out]
        n1122 = flat-sequence {
          tunnel: w992 -> [w1041]
          tunnel: w991 -> [w1040]
          tunnel: [w1039] -> w984
          tunnel: [w1038] -> w983
          tunnel: [w1044] -> w985
          tunnel: [w1045] -> w990
          tunnel: w984 -> [w1045]
          tunnel: w983 -> [w1044]
          frame #0 {
            w1035 = u8 0
            w1036 = u16 0 ("AudioLeft_phase_inc")
            w1037 = FALSE
            n1123 = xnode "Read/Write Control"("FPGA VI Reference In"=w1041, "error in"=w1040, "Counts_Reset"=TRUE, "audioTrigger_L"=w1037, "audioFreq_L_kHz"=w1035, "audioAmp_L"=w1036, "audioTrigger_R"=w1037, "audioFreq_R_kHz"=w1035, "audioAmp_R"=w1036, "A3_SL"=w1037, "A1_SR"=w1037, "A6_Act"=w1037) -> ("FPGA VI Reference Out"=w1039:refnum<k20>, "error out"=w1038:errorcluster)
          }
          frame #1 {
            w1043 = FALSE ("START")
            n1124 = local write "START"(w1043) -> ()
            n1125 = local write "STOP_endTrial"(w1043) -> ()
            n1126 = local write "STOP_endBlock"(w1043) -> ()
          }
        }
        n1127 = stacked-sequence {
          tunnel: w968 -> [w1015 _]
          tunnel: w966 -> [w1016 _]
          tunnel: w965 -> [_ w1021]
          tunnel: w964 -> [_ w1020]
          tunnel: w963 -> [_ w1019]
          tunnel: w962 -> [w1009 _]
          tunnel: w936 -> [w1006 _]
          tunnel: w935 -> [w1005 _]
          frame #0 {
            n1128 = call "myRIO_BRig_RT_dataCurrent_idxDataLick.vi"() -> ("output_idxDataLick"=w1010:i32)  [unwired: 11 in]
            n1129 = Index Array(array=w1009, index=w1010) -> (element=w1012:u16)
            n1130 = Array Subset(array=w1006, length (row)=w1005) -> (w1007:u16[][])  [unwired: 3 in]
            n1131 = Increment(x=w1012) -> (x+1=w1013:u16)
            n1132 = call "myRIO_BRig_RT_comm_webdav_saveArrayToFile__1D_u16.vi"("Array"=w1016, "input_filename"="dataMTrig") -> ()  [unwired: 10 in]
            n1133 = To Long Integer(number=w1013) -> (32bit integer=w1011:i32)
            n1134 = Array Subset(array=w1015, length (row)=w1011) -> (w1014:u16[][])  [unwired: 3 in]
            n1135 = call "myRIO_BRig_RT_comm_webdav_saveArrayToFile__2D_u16.vi"("Array"=w1014, "input_filename"="dataLick") -> ()  [unwired: 10 in]
            n1136 = call "myRIO_BRig_RT_comm_webdav_saveArrayToFile__2D_u16.vi"("Array"=w1007, "input_filename"="dataAnalog") -> ()  [unwired: 10 in]
          }
          frame #1 {
            n1137 = case shown="True" w1021 {
              tunnel: w1020 -> [_ w1023]
              tunnel: w1019 -> [_ w1022]
              frame False {
              }
              frame True {
                n1138 = stacked-sequence {
                  tunnel: w1023 -> [w1025 w1032 w1034]
                  tunnel: w1022 -> [w1026 w1031 _]
                  frame #0 {
                    n1139 = call "myRIO_BRig_RT_comm_webdav_uploadFile__announce.vi"("input_addText"=TRUE, "input_fileName_prefix"=w1026, "intput_fileName"="curExp_end", "intput_hSession"=w1025) -> ("output_Isuccess"=w1024:bool)  [unwired: 6 in, 1 out]
                    n1140 = case shown="True" w1024 {
                      frame False {
                        n1141 = One Button Dialog(message="!!! Warning !!! Your data is located at C:\\BehaviorRig\\commTransfer") -> ()  [unwired: 1 in, 1 out]
                      }
                      frame True {
                        n1142 = Wait (ms)(milliseconds to wait=u32 20) -> ()  [unwired: 1 out]
                      }
                    }
                  }
                  frame #1 {
                    n1143 = call "myRIO_BRig_RT__endExp_sendData.vi"("input_fileName_prefix"=w1031, "input_hSession"=w1032) -> ()  [unwired: 8 in, 2 out]
                  }
                  frame #2 {
                    n1144 = local write "Connected To Host?"(FALSE ("Connected To Host?")) -> ()
                    n1145 = call <vilib>:"Close Session.vi"("session handle"=w1034) -> ()  [unwired: 14 in, 1 out]
                  }
                }
              }
            }
          }
        }
      }
    }
    n1146 = local read "STOP_abort"() -> (w43:bool)
  }
  n1147 = case shown="True" w3 {
    tunnel: w2 -> [_ w3234]
    tunnel: w1 -> [_ w3233]
    frame False {
    }
    frame True {
      n1148 = call "myRIO__TCP_disconnect_forWrite.vi"("input_error"=w3233, "input_hTCP"=w3234) -> ()  [unwired: 9 in, 1 out]
    }
  }
  n1149 = xnode "Read/Write Control"("FPGA VI Reference In"=w15, "error in"=w14, "FPGA_Stop"=TRUE) -> ("FPGA VI Reference Out"=w20:refnum<k20>, "error out"=w21:errorcluster)
  n1150 = xnode "Close FPGA VI Reference"("FPGA VI Reference In"=w20, "error in"=w21) -> ("error out"=w19:errorcluster)
  n1151 = call <vilib>:"Reset myRIO.vi"("error in (no error)"=w19) -> ()  [unwired: 10 in, 1 out]
